vi "SQL_CLIENT_MAIN.vi"() -> ()   [LabVIEW 2020]
uses:
  SQL_CLIENT/MAIN/REF_EDITOR/REF_EDIT_type_filter.ctl
  SQL_CLIENT/MAIN/REPORTS/REPORTS_filters.ctl
  SQL_CLIENT/MAIN/REPORTS/REPORT_filter.ctl
  SQL_CLIENT/MAIN/REPORTS/GEAR/typedef/REPORT_GEAR_header_data_display.ctl
  SQL_CLIENT/MAIN/REPORTS/OPERATION/typedef/REPORT_OPRTN_operation.ctl
  SQL_CLIENT/MAIN/REPORTS/CONFIG_HISTORY/typedef/REPORT_CFG_types.ctl
  SQL_CLIENT/MAIN/REPORTS/REWORKS/typedef/REPORT_REWORKS_stations.ctl
  SQL_CLIENT/ini/typedef/CLIENT_all_config_info.ctl
  SQL_CLIENT/ini/typedef/CLIENT_main_ini_file.ctl
  SQL_CLIENT/queues/typedef/CLIENT_queue_refnums.ctl
  SQL_CLIENT/queues/typedef/SQL_EDITOR_queue_element.ctl
  SQL_CLIENT/MAIN/SQL_EDITOR/SQL_EDITOR_sequence_state.ctl
  SQL_CLIENT/queues/typedef/CLIENT_SCANNER_queue_element.ctl
  SQL_CLIENT/MAIN/SCANNER/SCANNER_sequence_state.ctl
  SQL_CLIENT/queues/typedef/CLIENT_REF_CHG_queue_element.ctl
  SQL_CLIENT/MAIN/reference_changed_connection/CLIENT_REF_CHG_sequence_state.ctl
  SQL_CLIENT/FGV/error_buffer/FGV_CLIENT_error_buffer.ctl
  SQL_CLIENT/FGV/SQL_EDITOR_records_display/FGV_SQL_EDITOR_records_display.ctl
  SQL_CLIENT/FGV/SQL_EDITOR_status_display/FGV_SQL_EDITOR_status_display.ctl
  SQL_CLIENT/FGV/SQL_connection/FGV_CLIENT_SQL_connection.ctl
  SQL_CLIENT/FGV/REF_EDITOR_records_display/FGV_REF_EDITOR_records_display.ctl
  SQL_CLIENT/FGV/REF_EDITOR_status_display/FGV_REF_EDITOR_status_display.ctl
  SQL_CLIENT/MAIN/CLIENT_event_structure_shift_register.ctl
  SQL_CLIENT/FGV/ARCH_EDITOR_status_display/FGV_ARCH_EDITOR_status_display.ctl
  SQL_CLIENT/FGV/ARCH_EDITOR_records_display/FGV_ARCH_EDITOR_records_display.ctl
  SQL_CLIENT/FGV/SQL_TEXT_status_display/FGV_SQL_TEXT_status_display.ctl
  SQL_CLIENT/FGV/SQL_TEXT_records_display/FGV_SQL_TEXT_records_display.ctl
  SQL_CLIENT/FGV/USER_EDITOR_status_display/FGV_USER_EDITOR_status_display.ctl
  SQL_CLIENT/FGV/USER_EDITOR_records_display/FGV_USER_EDITOR_records_display.ctl
  SQL_CLIENT/FGV/login/FGV_login.ctl
  SQL_CLIENT/FGV/REPORTS_status_display/FGV_REPORTS_status_display.ctl
  SQL_CLIENT/FGV/REPORTS_records_display/FGV_REPORTS_records_display.ctl
  SQL_CLIENT/FGV/REPORTS_records_display/REPORTS_references.ctl
  _misc/directions.ctl
  SQL_CLIENT/MAIN/REPORTS/AUDIT/typedef/REPORT_AUDIT_filters.ctl
  <vilib>/Utility/miscctls.llb/LVRowAndColumnTypeDef.ctl
  SQL_CLIENT/MAIN/REPORTS/CONFIG_HISTORY/typedef/REPORT_CFG_filters.ctl
  SQL_CLIENT/MAIN/REPORTS/DATES/typedef/REPORT_DATES_filters.ctl
  SQL_CLIENT/MAIN/REPORTS/OPERATION/typedef/REPORT_OPRTN_filters.ctl
  SQL_CLIENT/MAIN/REPORTS/PRODUCTION_BATCH/typedef/REPORT_PBATCH_filters.ctl
  SQL_CLIENT/MAIN/thread_name.ctl
  _misc/AULocalize/SubVIs/RegisterVI.vi
  _misc/AULocalize/SubVIs/Get Localized Phrase Compact Interface 0D.vi
  <vilib>/Instr/_visa.llb/VISA Configure Serial Port (Instr).vi
  <vilib>/regexp/Match Regular Expression.xnode
panel:
  out "app_title":string caption="A603 - SQL Client"
  out "PLC_PROXY_connection_indicator":bool=TRUE caption="PLC Proxy Connection Status:"
  in  "USER_login_logout":bool
  out "SQL_connection_indicator":bool=TRUE caption="SQL Connection Status:"
  in  "STOP":bool
  out "error_indicator_global":bool caption="Application Status:"
  in  "current_access_level":i32=10 caption="Access level:"
  in  "current_username":string="jlonga" caption="Logged in as:"
  in  "main_tab":T1(tab)
  in  "REPORT_save_csv":bool
  in  "REPORT_clear":bool
  out "REPORT_page_counter":string
  in  "REPORT_page_last":bool
  in  "REPORT_page_next":bool
  in  "REPORT_page_previous":bool
  in  "REPORT_page_first":bool
  in  "REPORT_save_pdf":bool
  in  "REPORT_get":bool
  in  "REPORT_filters":T2
  out "REPORT_GEAR_serial_display":string
  in  "REPORT_GEAR_toggle_all_results":bool
  in  "REPORT_GEAR_station":T3 caption="OP Filter:" items=["ALL", "10", "20", "30", "40"]
  in  "REPORT_GEAR_scan_barcode":bool
  in  "REPORT_GEAR_serial":string caption="Gear Serial:"
  out "REPORT_GEAR_header_data_display":T4
  out "gear_info_summary_header":string caption="GEAR INFO SUMMARY"
  in  "REPORT_DATES_last_status":T3 caption="Last Status:" items=["ALL", "0", "IN OPERATION", "INTERRUPTED", "NOK", "OK"]
  in  "REPORT_DATES_last_op":T3 caption="Last OP:" items=["ALL", "0", "10", "20", "40", "50", "60", "70", "80", "90", "100", "110", "120", "130", "160", "165"]
  in  "REPORT_DATES_time_end":timestamp caption="End:" format="%<%H:%M:%S>T"
  in  "REPORT_DATES_time_start":timestamp caption="Start:" format="%<%H:%M:%S>T"
  in  "REPORT_DATES_start":timestamp caption="From:" format="%<%x %H:%M:%S>T"
  in  "REPORT_DATES_start_btn":bool
  in  "REPORT_DATES_end":timestamp caption="To:" format="%<%x %H:%M:%S>T"
  in  "REPORT_DATES_end_btn":bool
  in  "REPORT_DATES_order_selection":enum32{"old_to_new", "new_to_old"}(radio)
  out "timeframe_header":string caption="TIMEFRAME"
  out "timeofday_header":string caption="TIME OF DAY / SHIFT"
  out "order_header":string caption="ORDER"
  out "filters_header":string caption="FILTERS"
  in  "REPORT_PBATCH_last_status":T3 caption="Last Status:" items=[" -"]
  in  "REPORT_PBATCH_last_op":T3 caption="Last OP:" items=[" -"]
  in  "REPORT_PBATCH_order_selection":enum32{"old_to_new", "new_to_old"}(radio)
  in  "REPORT_PBATCH_batch_no":string caption="Batch No:"
  out "batch_header":string caption="BATCH"
  out "order_header":string caption="ORDER"
  out "filters_header":string caption="FILTERS"
  in  "REPORT_OPRTN_order_selection":enum32{"old_to_new", "new_to_old"}(radio)
  in  "REPORT_OPRTN_end_btn":bool
  in  "REPORT_OPRTN_end":timestamp caption="To:" format="%<%x %H:%M:%S>T"
  in  "REPORT_OPRTN_start_btn":bool
  in  "REPORT_OPRTN_start":timestamp caption="From:" format="%<%x %H:%M:%S>T"
  in  "REPORT_OPRTN_time_start":timestamp caption="Start:" format="%<%H:%M:%S>T"
  in  "REPORT_OPRTN_time_end":timestamp caption="End:" format="%<%H:%M:%S>T"
  in  "REPORT_OPRTN_last_status":T3 caption="Last Status:" items=[" -"]
  in  "REPORT_OPRTN_operation":T5 caption="OP:" items=["10"=10, "20"=20, "30"=30, "40"=40, "50"=50, "60"=60, "70"=70, "80"=80, "90"=90, "100"=100, "110"=110, "120"=120, "130"=130, "140"=140, "150"=150, "160"=160, "165"=165]
  in  "REPORT_OPRTN_filter_columns":bool
  in  "REPORT_OPRTN_unfilter_columns":bool
  out "operation_header":string caption="OPERATION"
  out "timeframe_header":string caption="TIMEFRAME"
  out "timeofday_header":string caption="TIME OF DAY / SHIFT"
  out "order_header":string caption="ORDER"
  out "filters_header":string caption="FILTERS"
  in  "REPORT_CFG_type":T6 caption="Config:"
  in  "REPORT_CFG_time_end":timestamp caption="End:" format="%<%H:%M:%S>T"
  in  "REPORT_CFG_time_start":timestamp caption="Start:" format="%<%H:%M:%S>T"
  in  "REPORT_CFG_start":timestamp caption="From:" format="%<%x %H:%M:%S>T"
  in  "REPORT_CFG_start_btn":bool
  in  "REPORT_CFG_end":timestamp caption="To:" format="%<%x %H:%M:%S>T"
  in  "REPORT_CFG_end_btn":bool
  in  "REPORT_CFG_order_selection":enum32{"old_to_new", "new_to_old"}(radio)
  in  "REPORT_CFG_op_filter":T3 caption="OP:" items=[" -"]
  out "configtype_header":string caption="CONFIG TYPE"
  out "timeframe_header":string caption="TIMEFRAME"
  out "timeofday_header":string caption="TIME OF DAY / SHIFT"
  out "order_header":string caption="ORDER"
  out "filters_header":string caption="FILTERS"
  in  "REPORT_AUDIT_order_selection":enum32{"old_to_new", "new_to_old"}(radio)
  in  "REPORT_AUDIT_end_btn":bool
  in  "REPORT_AUDIT_end":timestamp caption="To:" format="%<%x %H:%M:%S>T"
  in  "REPORT_AUDIT_start_btn":bool
  in  "REPORT_AUDIT_start":timestamp caption="From:" format="%<%x %H:%M:%S>T"
  in  "REPORT_AUDIT_time_start":timestamp caption="Start:" format="%<%H:%M:%S>T"
  in  "REPORT_AUDIT_time_end":timestamp caption="End:" format="%<%H:%M:%S>T"
  in  "REPORT_AUDIT_OP_filter":T3 caption="Audit OP:" items=["ALL", "10", "20", "30", "40", "50", "60", "70", "80", "90", "100", "120", "165"]
  in  "REPORT_AUDIT_status_filter":T3 caption="Audit Status:" items=["ALL", "0", "NOK", "OK"]
  out "timeframe_header":string caption="TIMEFRAME"
  out "timeofday_header":string caption="TIME OF DAY / SHIFT"
  out "order_header":string caption="ORDER"
  out "filters_header":string caption="FILTERS"
  in  "REPORT_AUDIT_toggle_all_results":bool
  in  "REPORT_OKNOK_time_end":timestamp caption="End:" format="%<%H:%M:%S>T"
  in  "REPORT_OKNOK_time_start":timestamp caption="Start:" format="%<%H:%M:%S>T"
  in  "REPORT_OKNOK_start":timestamp caption="From:" format="%<%x %H:%M:%S>T"
  in  "REPORT_OKNOK_start_btn":bool
  in  "REPORT_OKNOK_end":timestamp caption="To:" format="%<%x %H:%M:%S>T"
  in  "REPORT_OKNOK_end_btn":bool
  out "timeframe_header":string caption="TIMEFRAME"
  out "timeofday_header":string caption="TIME OF DAY / SHIFT"
  in  "REPORT_REWORKS_end_btn":bool
  in  "REPORT_REWORKS_end":timestamp caption="To:" format="%<%x %H:%M:%S>T"
  in  "REPORT_REWORKS_start_btn":bool
  in  "REPORT_REWORKS_start":timestamp caption="From:" format="%<%x %H:%M:%S>T"
  in  "REPORT_REWORKS_time_start":timestamp caption="Start:" format="%<%H:%M:%S>T"
  in  "REPORT_REWORKS_time_end":timestamp caption="End:" format="%<%H:%M:%S>T"
  in  "REPORT_REWORKS_to_OP":T7 caption="To OP:" items=["0"=0, "10"=10, "20"=20, "30"=30, "40"=40, "50"=50, "60"=60, "70"=70, "80"=80, "90"=90, "100"=100, "110"=110, "120"=120, "130"=130, "140"=140, "150"=150, "160"=160, "165"=165]
  in  "REPORT_REWORKS_from_OP":T7 caption="From OP:" items=["0"=0, "10"=10, "20"=20, "30"=30, "40"=40, "50"=50, "60"=60, "70"=70, "80"=80, "90"=90, "100"=100, "110"=110, "120"=120, "130"=130, "140"=140, "150"=150, "160"=160, "165"=165]
  in  "REPORT_REWORKS_order_selection":enum32{"old_to_new", "new_to_old"}(radio)
  out "timeframe_header":string caption="TIMEFRAME"
  out "timeofday_header":string caption="TIME OF DAY / SHIFT"
  out "sourcedestination_header":string caption="SOURCE AND DESTIONATION"
  out "order_header":string caption="ORDER"
  in  "REPORT_PACE_end_btn":bool
  in  "REPORT_PACE_end":timestamp caption="To:" format="%<%x %H:%M:%S>T"
  in  "REPORT_PACE_start_btn":bool
  in  "REPORT_PACE_start":timestamp caption="From:" format="%<%x %H:%M:%S>T"
  in  "REPORT_PACE_time_start":timestamp caption="Start:" format="%<%H:%M:%S>T"
  in  "REPORT_PACE_time_end":timestamp caption="End:" format="%<%H:%M:%S>T"
  in  "REPORT_PACE_low_limit":u16 caption="Low:" step=1
  in  "REPORT_PACE_high_limit":u16 caption="High:" step=1
  out "timeframe_header":string caption="TIMEFRAME"
  out "timeofday_header":string caption="TIME OF DAY / SHIFT"
  out "pacelimits_header":string caption="PACE LIMITS (SECONDS)"
  in  "REPORT_CBATCH_batch_code":string caption="Batch:"
  in  "REPORT_CBATCH_scan_barcode":bool
  in  "REPORT_CBATCH_order_selection":enum32{"old_to_new", "new_to_old"}(radio)
  out "order_header":string caption="ORDER"
  in  "REPORT_CMPNT_scan_barcode":bool
  in  "REPORT_CMPNT_gear_serial":string caption="Gear Serial:"
  in  "REPORT_records":i32(listbox)=-1
  out "REPORT_status":string
  in  "REF_EDIT_type_filter":T8 caption="Type:"
  in  "REF_EDIT_records":i32(listbox)
  in  "REF_EDIT_station":u16(ring) caption="Station:" items=["10", "20", "30", "40", "50", "60", "70", "80", "90", "100", "110", "120", "130", "160", "165"]
  out "REF_EDIT_status":string
  in  "REF_EDIT_refresh":bool
  in  "REF_EDIT_delete":bool
  in  "REF_EDIT_insert_update":bool
  in  "REF_EDIT_clear_status":bool
  in  "REF_EDIT_discard":bool
  in  "ARCH_EDIT_type_filter":T8 caption="Type:"
  in  "ARCH_EDIT_records":i32(listbox)
  in  "ARCH_EDIT_station":u16(ring) caption="Station:" items=["10", "20", "30", "40", "50", "60", "70", "80", "90", "100", "110", "120", "130", "140", "160", "165"]
  out "ARCH_EDIT_status":string
  in  "ARCH_EDIT_refresh":bool
  in  "ARCH_EDIT_delete":bool
  in  "ARCH_EDIT_insert_update":bool
  in  "ARCH_EDIT_clear_status":bool
  in  "ARCH_EDIT_discard":bool
  in  "USER_EDIT_refresh":bool
  out "USER_EDIT_status":string
  in  "USER_EDIT_records":i32(listbox)
  in  "USER_EDIT_insert_update":bool
  in  "USER_EDIT_delete":bool
  in  "USER_EDIT_clear_status":bool
  in  "USER_EDIT_discard":bool
  in  "USER_EDIT_update_barcode":bool
  in  "SQL_EDIT_asc_desc":enum32{"ASC", "DESC"}(radio)
  in  "SQL_EDIT_order_by":u16(ring) caption="Order by:" items=["ID", "CREATION_TIME", "REFERENCE_NAME", "STATION_NMB", "DESCRIPTION", "UNIT", "PLC_TAG_TYPE", "PLC_TAG_ADDRESS", "CREATED_BY"]
  in  "SQL_EDIT_discard":bool
  in  "SQL_EDIT_clear_status":bool
  in  "SQL_EDIT_select":bool
  in  "SQL_EDIT_value":string caption="Value:"
  in  "SQL_EDIT_table":u16(ring) caption="Table:" items=["ARCHIVISATION_AUDIT", "ARCHIVISATION_CFG", "ARCHIVISATION_CFG_HISTORY", "AUDIT_RESULTS", "AUDIT_RESULTS_REAL", "DOCK_AUDIT_BATCH_COUNT", "DOCK_AUDIT_BATCH_SIZE", "DOCK_AUDIT_BATCHES", "MAX_REPEAT_COUNT", "OEE_AVAILABILITY", "OEE_CONFIG", "OEE_SHIFT_TIMES", "OEE_tmp_operations_memory_optimized", "PRODUCTION_BATCHES", "PRODUCTION_BATCHES_OPERATIONS", "PRODUCTION_PARTS", "PRODUCTION_PARTS_OPERATIONS", "PRODUCTION_PARTS_OPERATIONS_RESULTS_REAL", "PRODUCTION_PARTS_OPERATIONS_RESULTS_STRING", "PRODUCTION_PINIONS", "REFERENCE", "REFERENCE_HISTORY", "REWORK", "ROUTING", "USER_DATA", "USER_DATA_HISTORY"]
  in  "SQL_EDIT_column":u16(ring) caption="Column:" items=["ID", "CREATION_TIME", "REFERENCE_NAME", "STATION_NMB", "DESCRIPTION", "UNIT", "PLC_TAG_TYPE", "PLC_TAG_ADDRESS", "CREATED_BY"]
  in  "SQL_EDIT_insert_update":bool
  in  "SQL_EDIT_delete":bool
  in  "SQL_EDIT_records":i32(listbox)=-1
  out "SQL_EDIT_status":string
  in  "SQL_TEXT_execute":bool
  in  "SQL_TEXT_clear_status":bool
  in  "SQL_TEXT_input":string
  out "SQL_TEXT_status":string
  in  "SQL_TEXT_records":i32(listbox)
  in  "main_error":i32(listbox)
  in  "ERRORS_clear":bool
  out "error_indicator_tab":bool
  # "Access Levels:"
  # "1 - Operator, 2 - Leader, 3 - Maintenance, 7 - Engineer, 10 - Admin"
  # "WARNING! - SQL COMMANDS EXECUTED IN THIS WINDOW ARE NOT VALIDATED IN ANY WAY AND CAN IRREVERSIBLY DAMAGE THE DATABASE! - PROCEED WITH EXTREME CAUTION!"
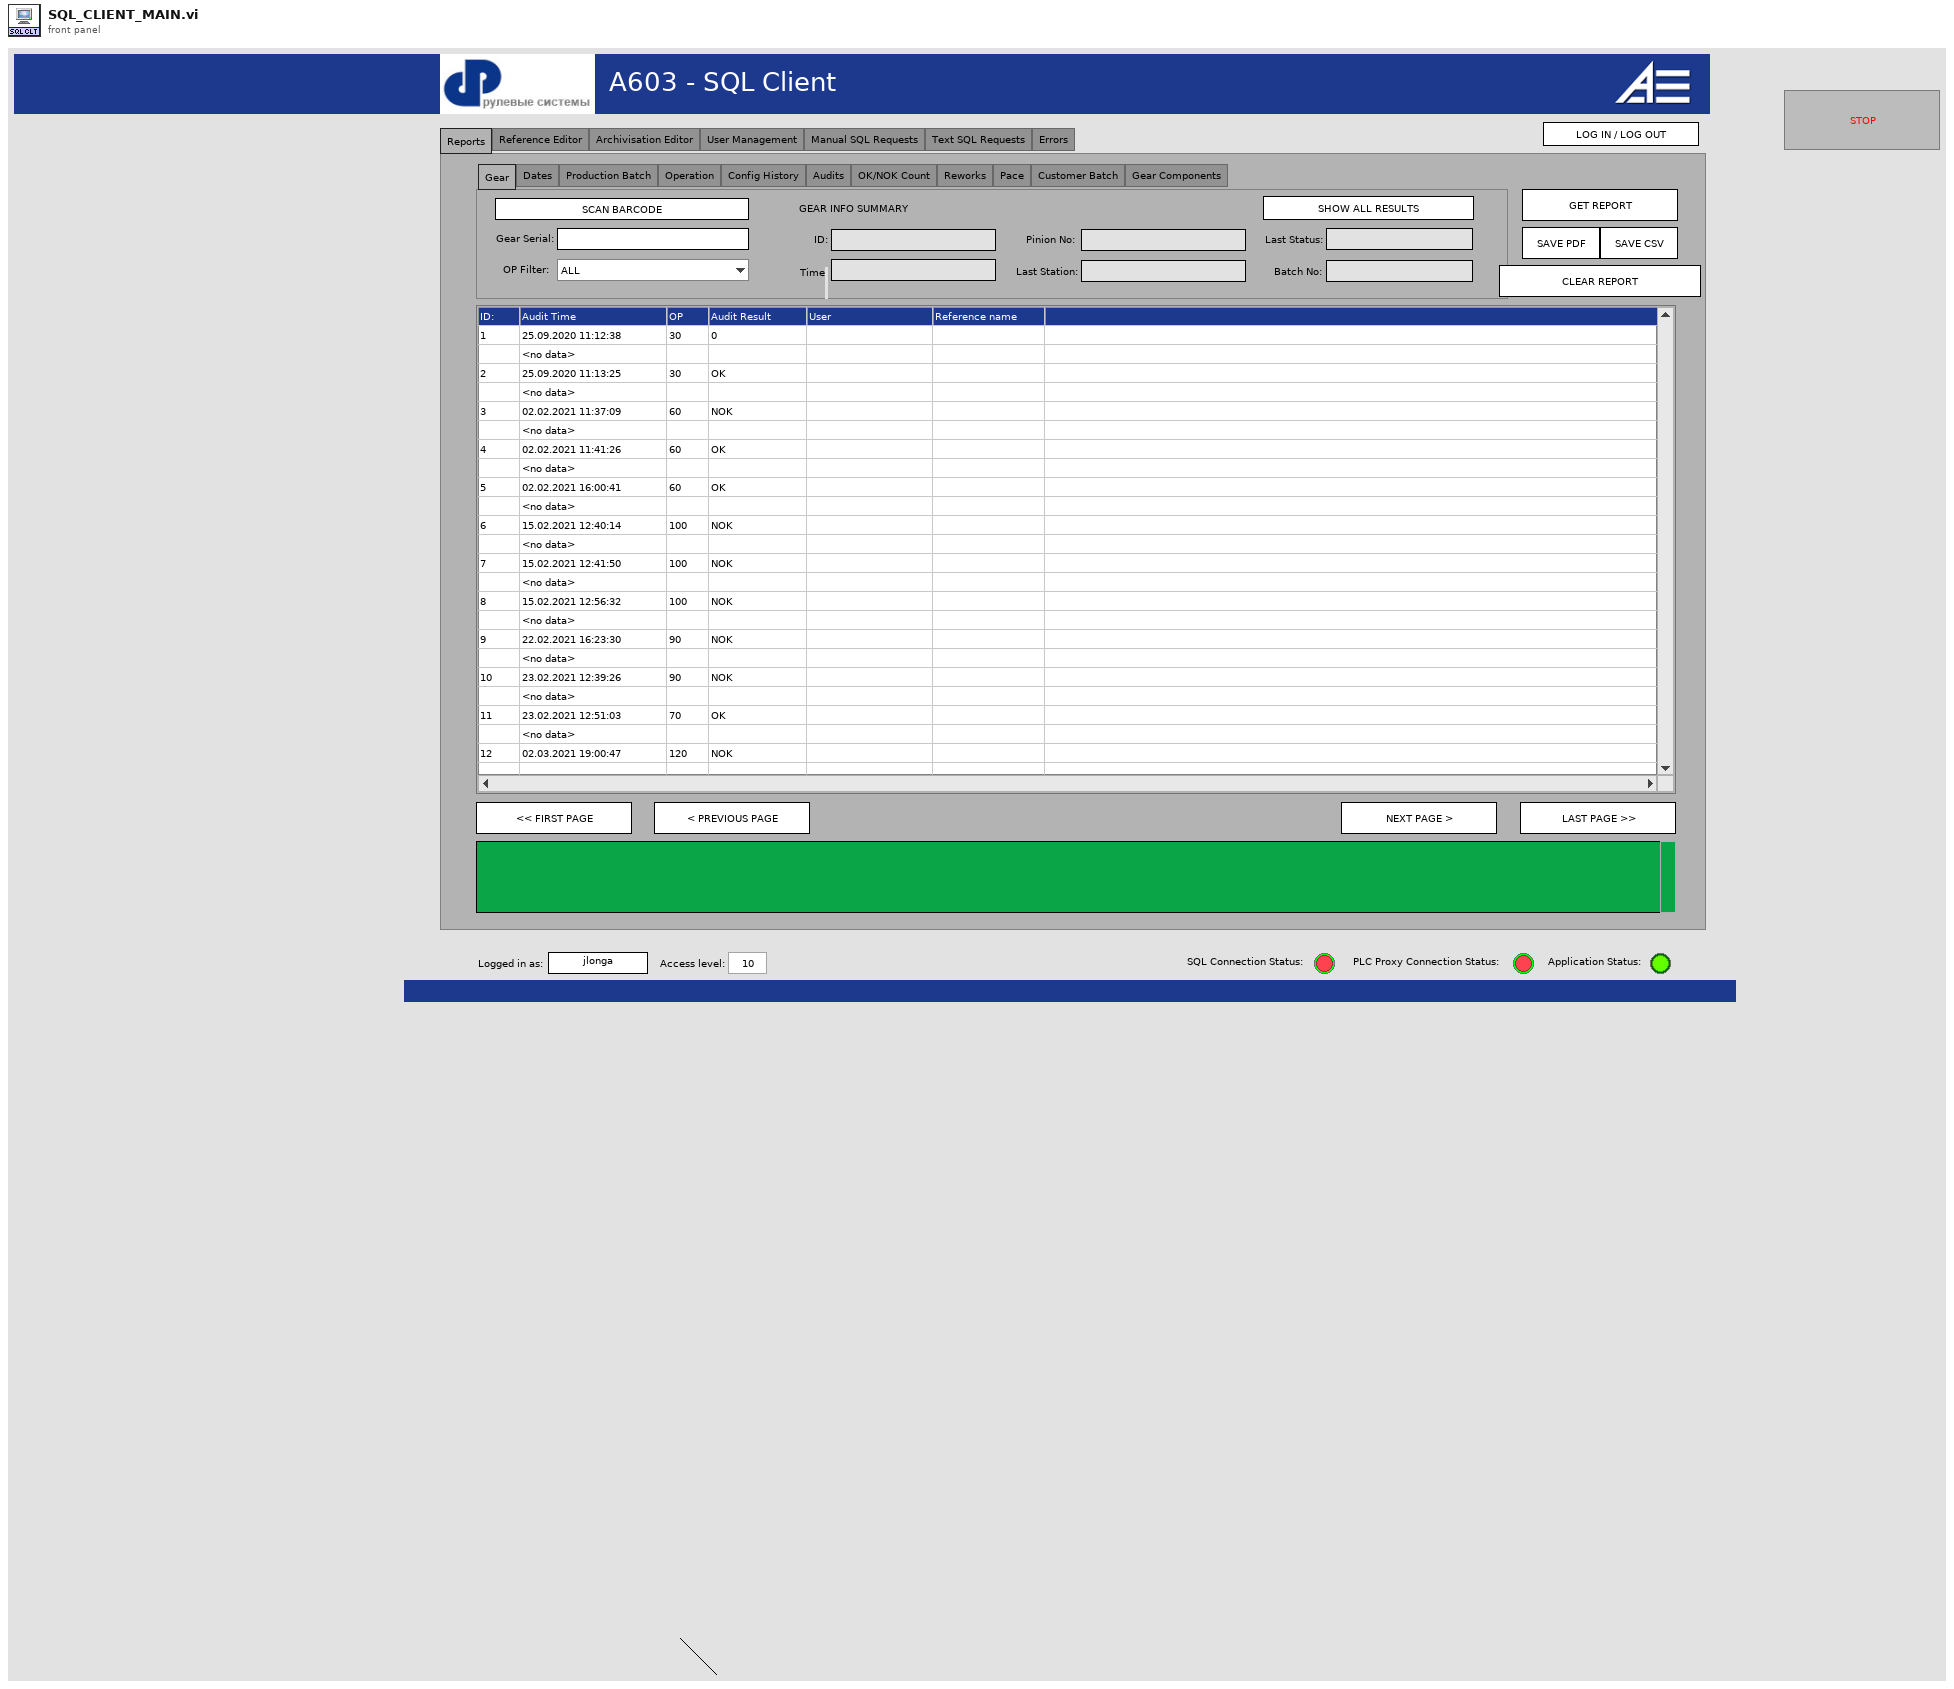
[diagram p1: front panel]
types:
  T1 = enum32{"Reports", "Reference Editor", "Archivisation Editor", "User Management", "Manual SQL Requests", "Text SQL Requests", "Errors"}
  T2 = typedef "REPORTS_filters.ctl" = enum32{"Gear", "Dates", "Production Batch", "Operation", "Config History", "Audits", "OK/NOK Count", "Reworks", "Pace", "Customer Batch", "Gear Components"}
  T3 = typedef "REPORT_filter.ctl" = u16
  T4 = typedef "REPORT_GEAR_header_data_display.ctl" = cluster{"ID":string, "creation_time":string, "last_station":string, "last_status":string, "pinion_serial":string, "batch_code":string}
  T5 = typedef "REPORT_OPRTN_operation.ctl" = u16
  T6 = typedef "REPORT_CFG_types.ctl" = enum16{"REFERENCE", "ARCHIVISATION", "USERS"}
  T7 = typedef "REPORT_REWORKS_stations.ctl" = u16
  T8 = typedef "REF_EDIT_type_filter.ctl" = enum32{"ALL", "INT", "REAL", "STRING"}
  T9 = typedef "CLIENT_REF_CHG_sequence_state.ctl" = enum16{"initialize", "get_next_state", "reference_changed", "ping", "error", "stop"}
  T10 = typedef "REPORTS_references.ctl" = cluster{"front_panel_reference":refnum<vi>, "SQL_listbox_reference":refnum<vi>, "REPORT_page_first":refnum<vi>, "REPORT_page_previous":refnum<vi>, "REPORT_page_next":refnum<vi>, "REPORT_page_last":refnum<vi>, "REPORT_page_counter":refnum<vi>, "REPORT_GEAR_serial":refnum<vi>, "REPORT_GEAR_serial_display":refnum<vi>, "REPORT_GEAR_station":refnum<vi>, "REPORT_GEAR_header_data_display":refnum<vi>, "REPORT_DATES_start":refnum<vi>, "REPORT_DATES_end":refnum<vi>, "REPORT_DATES_time_start":refnum<vi>, "REPORT_DATES_time_end":refnum<vi>, "REPORT_DATES_order_selection":refnum<vi>, "REPORT_DATES_last_OP":refnum<vi>, "REPORT_DATES_last_status":refnum<vi>, "REPORT_PBATCH_batch_no":refnum<vi>, "REPORT_PBATCH_order_selection":refnum<vi>, "REPORT_PBATCH_last_op":refnum<vi>, "REPORT_PBATCH_last_status":refnum<vi>, "REPORT_OPRTN_operation":refnum<vi>, "REPORT_OPRTN_start":refnum<vi>, "REPORT_OPRTN_end":refnum<vi>, "REPORT_OPRTN_time_start":refnum<vi>, "REPORT_OPRTN_time_end":refnum<vi>, "REPORT_OPRTN_order_selection":refnum<vi>, "REPORT_OPRTN_last_status":refnum<vi>, "REPORT_CFG_type":refnum<vi>, "REPORT_CFG_start":refnum<vi>, "REPORT_CFG_end":refnum<vi>, "REPORT_CFG_time_start":refnum<vi>, "REPORT_CFG_time_end":refnum<vi>, "REPORT_CFG_order_selection":refnum<vi>, "REPORT_CFG_op_filter":refnum<vi>, "REPORT_AUDIT_start":refnum<vi>, "REPORT_AUDIT_end":refnum<vi>, "REPORT_AUDIT_time_start":refnum<vi>, "REPORT_AUDIT_time_end":refnum<vi>, "REPORT_AUDIT_order_selection":refnum<vi>, "REPORT_AUDIT_op_filter":refnum<vi>, "REPORT_AUDIT_status_filter":refnum<vi>, "REPORT_OKNOK_start":refnum<vi>, "REPORT_OKNOK_end":refnum<vi>, "REPORT_OKNOK_time_start":refnum<vi>, "REPORT_OKNOK_time_end":refnum<vi>, "REPORT_REWORKS_start":refnum<vi>, "REPORT_REWORKS_end":refnum<vi>, "REPORT_REWORKS_time_start":refnum<vi>, "REPORT_REWORKS_time_end":refnum<vi>, "REPORT_REWORKS_from_OP":refnum<vi>, "REPORT_REWORKS_to_OP":refnum<vi>, "REPORT_REWORKS_order_selection":refnum<vi>, "REPORT_PACE_start":refnum<vi>, "REPORT_PACE_end":refnum<vi>, "REPORT_PACE_time_start":refnum<vi>, "REPORT_PACE_time_end":refnum<vi>, "REPORT_PACE_low_limit":refnum<vi>, "REPORT_PACE_high_limit":refnum<vi>, "REPORT_CBATCH_batch_code":refnum<vi>, "REPORT_CBATCH_order_selection":refnum<vi>, "REPORT_CMPNT_gear_serial":refnum<vi>}
  T11 = typedef "FGV_REPORTS_records_display.ctl" = enum16{"initialize", "GEAR_set_serial", "GEAR_set_header", "GEAR_set_operations", "GEAR_set_results", "GEAR_set_batches", "GEAR_get_serial", "GEAR_get_operation_IDs", "GEAR_toggle_results", "GEAR_show_all_results", "GEAR_hide_all_results", "GEAR_display", "GEAR_filter", "GEAR_restore", "GEAR_clear", "GEAR_get_all_info", "DATES_set_dates", "DATES_set_gears", "DATES_display", "DATES_filter", "DATES_first_page", "DATES_previous_page", "DATES_next_page", "DATES_last_page", "DATES_restore", "DATES_clear", "DATES_get_all_info", "PBATCH_set_batch_no", "PBATCH_set_gears", "PBATCH_display", "PBATCH_filter", "PBATCH_first_page", "PBATCH_previous_page", "PBATCH_next_page", "PBATCH_last_page", "PBATCH_restore", "PBATCH_clear", "PBATCH_get_all_info", "OPRTN_set_OP", "OPRTN_set_dates", "OPRTN_set_gears", "OPRTN_set_hidden_columns", "OPRTN_display", "OPRTN_filter", "OPRTN_filter_no_page_reset", "OPRTN_first_page", "OPRTN_previous_page", "OPRTN_next_page", "OPRTN_last_page", "OPRTN_restore", "OPRTN_clear", "OPRTN_get_all_info", "CFG_set_type", "CFG_set_dates", "CFG_set_records", "CFG_display", "CFG_filter", "CFG_first_page", "CFG_previous_page", "CFG_next_page", "CFG_last_page", "CFG_restore", "CFG_clear", "CFG_get_all_info", "AUDIT_set_dates", "AUDIT_set_records", "AUDIT_display", "AUDIT_filter", "AUDIT_first_page", "AUDIT_previous_page", "AUDIT_next_page", "AUDIT_last_page", "AUDIT_restore", "AUDIT_clear", "AUDIT_set_results", "AUDIT_get_all_info", "AUDIT_toggle_results", "AUDIT_show_all_results", "AUDIT_hide_all_results", "OKNOK_set_dates", "OKNOK_set_records", "OKNOK_display", "OKNOK_restore", "OKNOK_clear", "OKNOK_get_all_info", "REWORKS_set_dates", "REWORKS_set_from_to", "REWORKS_set_records", "REWORKS_display", "REWORKS_filter", "REWORKS_first_page", "REWORKS_previous_page", "REWORKS_next_page", "REWORKS_last_page", "REWORKS_restore", "REWORKS_clear", "REWORKS_get_all_info", "PACE_set_dates", "PACE_set_limits", "PACE_set_records", "PACE_display", "PACE_restore", "PACE_clear", "PACE_get_all_info", "CBATCH_set_code", "CBATCH_set_records", "CBATCH_display", "CBATCH_filter", "CBATCH_first_page", "CBATCH_previous_page", "CBATCH_next_page", "CBATCH_last_page", "CBATCH_restore", "CBATCH_clear", "CBATCH_get_all_info", "CMPNT_set_serial", "CMPNT_set_records", "CMPNT_display", "CMPNT_first_page", "CMPNT_previous_page", "CMPNT_next_page", "CMPNT_last_page", "CMPNT_restore", "CMPNT_clear", "CMPNT_get_all_info", "clear"}
  T12 = typedef "FGV_REPORTS_status_display.ctl" = enum16{"initialize", "display", "clear"}
  T13 = typedef "FGV_login.ctl" = enum16{"initialize", "login", "logout", "get_login_info"}
  T14 = typedef "FGV_USER_EDITOR_records_display.ctl" = enum16{"initialize", "set_user_edit_tables_names", "set_headers", "set_records", "get_user_edit_table_name", "get_user_edit_hist_table_name", "get_headers", "get_uneditable_columns", "get_all_info", "record_added?", "record_inserted?", "record_edited?", "record_updated?", "record_deleted?", "discard_changes"}
  T15 = typedef "FGV_USER_EDITOR_status_display.ctl" = enum16{"initialize", "display", "clear"}
  T16 = typedef "FGV_SQL_TEXT_records_display.ctl" = enum16{"initialize", "set", "clear"}
  T17 = typedef "FGV_SQL_TEXT_status_display.ctl" = enum16{"initialize", "display", "clear"}
  T18 = typedef "SCANNER_sequence_state.ctl" = enum16{"initialize", "get_next_state", "read", "cancel_read", "error", "stop"}
  T19 = typedef "FGV_ARCH_EDITOR_records_display.ctl" = enum16{"initialize", "set_arch_cfg_tables_names", "set_station_number", "set_type_filter", "set_headers", "set_records", "get_arch_cfg_table_name", "get_arch_cfg_hist_table_name", "get_station_number", "get_type_filter", "get_headers", "get_uneditable_columns", "get_all_info", "record_added?", "record_inserted?", "record_edited?", "record_updated?", "record_deleted?", "discard_changes"}
  T20 = typedef "FGV_ARCH_EDITOR_status_display.ctl" = enum16{"initialize", "display", "clear"}
  T21 = typedef "CLIENT_event_structure_shift_register.ctl" = cluster{"REF_EDIT_clicked_row":i32, "REF_EDIT_selected_row":i32, "SQL_EDIT_clicked_row":i32, "SQL_EDIT_selected_row":i32, "ARCH_EDIT_selected_row":i32, "ARCH_EDIT_clicked_row":i32, "USER_EDIT_selected_row":i32, "USER_EDIT_clicked_row":i32, "REPORT_GEAR_toggle_all_results":bool, "REPORT_AUDIT_toggle_all_results":bool}
  T22 = typedef "FGV_REF_EDITOR_status_display.ctl" = enum16{"initialize", "display", "clear"}
  T23 = typedef "FGV_REF_EDITOR_records_display.ctl" = enum16{"initialize", "set_reference_tables_names", "set_station_number", "set_type_filter", "set_headers", "set_records", "get_ref_table_name", "get_ref_hist_table_name", "get_station_number", "get_type_filter", "get_headers", "get_uneditable_columns", "get_all_info", "record_added?", "record_inserted?", "record_edited?", "record_updated?", "record_deleted?", "discard_changes"}
  T24 = typedef "FGV_CLIENT_SQL_connection.ctl" = enum16{"initialize", "connect", "read_tables", "read_columns", "SELECT", "INSERT", "UPDATE", "DELETE", "EXEC + headers", "EXEC", "TRANSACTION", "connection_active?", "disconnect"}
  T25 = typedef "SQL_EDITOR_sequence_state.ctl" = enum16{"initialize", "get_next_state", "REF_read_columns", "REF_read_stations", "REF_select_station_records", "REF_insert_record", "REF_update_record", "REF_delete_record", "REF_send_reference_updated_to_PLC", "ARCH_read_columns", "ARCH_read_stations", "ARCH_select_station_records", "ARCH_insert_record", "ARCH_update_record", "ARCH_delete_record", "USER_read_columns", "USER_select_records", "USER_insert_record", "USER_update_record", "USER_delete_record", "USER_update_barcode", "USER_login", "USER_logout", "SQL_read_tables", "SQL_read_columns", "SQL_select_records", "SQL_insert_record", "SQL_update_record", "SQL_delete_record", "SQL_TEXT_execute", "REPORT_GEAR_scan_barcode", "REPORT_GEAR_get", "REPORT_DATES_get", "REPORT_PBATCH_get", "REPORT_OPRTN_get", "REPORT_CFG_get", "REPORT_AUDIT_get", "REPORT_OKNOK_get", "REPORT_REWORKS_get", "REPORT_PACE_get", "REPORT_CBATCH_scan_barcode", "REPORT_CBATCH_get", "REPORT_CMPNT_scan_barcode", "REPORT_CMPNT_get", "REPORT_save_pdf", "REPORT_save_csv", "error", "stop"}
  T26 = typedef "FGV_SQL_EDITOR_status_display.ctl" = enum16{"initialize", "display", "clear"}
  T27 = typedef "FGV_SQL_EDITOR_records_display.ctl" = enum16{"initialize", "set_table_name", "set_column_name", "set_value_to_select", "set_order_by", "set_asc_desc", "set_headers", "set_records", "get_table_name", "get_column_name", "get_value_to_select", "get_headers", "get_all_info", "record_added?", "record_inserted?", "record_edited?", "record_updated?", "record_deleted?", "discard_changes"}
  T28 = typedef "FGV_CLIENT_error_buffer.ctl" = enum16{"initialize", "clear", "display", "get_status"}
  T29 = typedef "CLIENT_all_config_info.ctl" = cluster{"main_ini_file":T30, "SQL Password":string, "queue_refnums":T31}
  T30 = typedef "CLIENT_main_ini_file.ctl" = cluster{"SQL Driver":string, "SQL Server":string, "SQL Database":string, "SQL UID":string, "Reference table":string, "Reference history":string, "Archivisation CFG table":string, "Archivisation CFG history":string, "User table":string, "User history":string, "logout timeout [ms]":i32, "records per page":i32, "default language":string, "REF CHG connection IP":string, "REF CHG remote port":i32, "REF CHG local port":i32, "SCANNER COM port":u16, "SCANNER Baud rate":u32, "SCANNER Data bits":u16, "SCANNER Pairity":enum16{"None", "Odd", "Even", "Mark", "Space"}, "SCANNER Stop bits":u16, "SCANNER Flow control":u16, "SCANNER Termination char":u8}
  T31 = typedef "CLIENT_queue_refnums.ctl" = cluster{"SQL_EDITOR_queue":refnum<queue>, "SCANNER_queue":refnum<queue>, "SCANNER_data":refnum<queue>, "CLIENT_REF_CHG_queue":refnum<queue>}
  T32 = typedef "SQL_EDITOR_queue_element.ctl" = cluster{"state":T25, "variable":variant}
  T33 = typedef "directions.ctl" = enum16{"UP", "DOWN", "LEFT", "RIGHT"}
  T34 = enum32{"Page Enabled", "Page Disabled", "Page Disabled & Grayed"}
  T35 = typedef "REPORT_AUDIT_filters.ctl" = cluster{"order_selection":enum32{"old_to_new", "new_to_old"}, "OP_filter":string, "status_filter":string, "show_hidden?":bool}
  T36 = typedef "LVRowAndColumnTypeDef.ctl" = cluster{"Row":i32, "Column":i32}
  T37 = typedef "REPORT_CFG_filters.ctl" = cluster{"order_selection":enum32{"old_to_new", "new_to_old"}, "OP":string}
  T38 = typedef "REPORT_DATES_filters.ctl" = cluster{"order_selection":enum32{"old_to_new", "new_to_old"}, "last_OP":string, "last_status":string}
  T39 = typedef "REPORT_OPRTN_filters.ctl" = cluster{"order_selection":enum32{"old_to_new", "new_to_old"}, "last_status":string}
  T40 = typedef "REPORT_PBATCH_filters.ctl" = cluster{"order_selection":enum32{"old_to_new", "new_to_old"}, "last_OP":string, "last_status":string}
  T41 = typedef "CLIENT_REF_CHG_queue_element.ctl" = cluster{"state":T9, "variable":variant}
  T42 = typedef "CLIENT_SCANNER_queue_element.ctl" = cluster{"state":T18, "variable":variant}
  T43 = typedef "ARCH_EDITOR_all_info.ctl" = cluster{"station_number":string, "type_filter":string, "archivisation_cfg_table":string, "archivisation_cfg_history":string, "column_names":string[], "uneditable_columns":string[], "uneditable_columns":i32[], "editable_columns":i32[], "values_in_database":string[][], "size":cluster{"columns":i32, "SQL_rows":i32, "disp_rows":i32}, "ARCH_record_states":T44[]}
  T44 = typedef "SQL_record_states.ctl" = enum16{"Equal", "Added", "Edited", "Deleted"}
  T45 = typedef "LVPoint32TypeDef.ctl" = cluster{"Horizontal":i32, "Vertical":i32}
  T46 = enum32{"Reports", "Reference Editor", "Archivisation Editor", "User Management", "Manual SQL Requests", "Text SQL Requests", "Errors"}[]
  T47 = typedef "REF_EDITOR_all_info.ctl" = cluster{"station_number":string, "type_filter":string, "reference_table":string, "reference_history":string, "headers":string[], "uneditable_columns":string[], "uneditable_columns":i32[], "editable_columns":i32[], "values_in_database":string[][], "size":cluster{"columns":i32, "SQL_rows":i32, "disp_rows":i32}, "REF_record_states":T44[]}
  T48 = typedef "SQL_EDITOR_all_info.ctl" = cluster{"table":string, "column":string, "value_to_select":string, "order_by":string, "asc_desc":string, "headers":string[], "uneditable_columns":string[], "uneditable_columns":i32[], "editable_columns":i32[], "values_in_database":string[][], "size":cluster{"columns":i32, "SQL_rows":i32, "disp_rows":i32}, "SQL_record_states":T44[]}
  T49 = typedef "USER_EDITOR_all_info.ctl" = cluster{"user_table":string, "user_history":string, "headers":string[], "uneditable_columns":string[], "uneditable_columns":i32[], "editable_columns":i32[], "values_in_database":string[][], "size":cluster{"columns":i32, "SQL_rows":i32, "disp_rows":i32}, "USER_record_states":T44[]}
  T50 = typedef "thread_name.ctl" = enum16{"MAIN"}
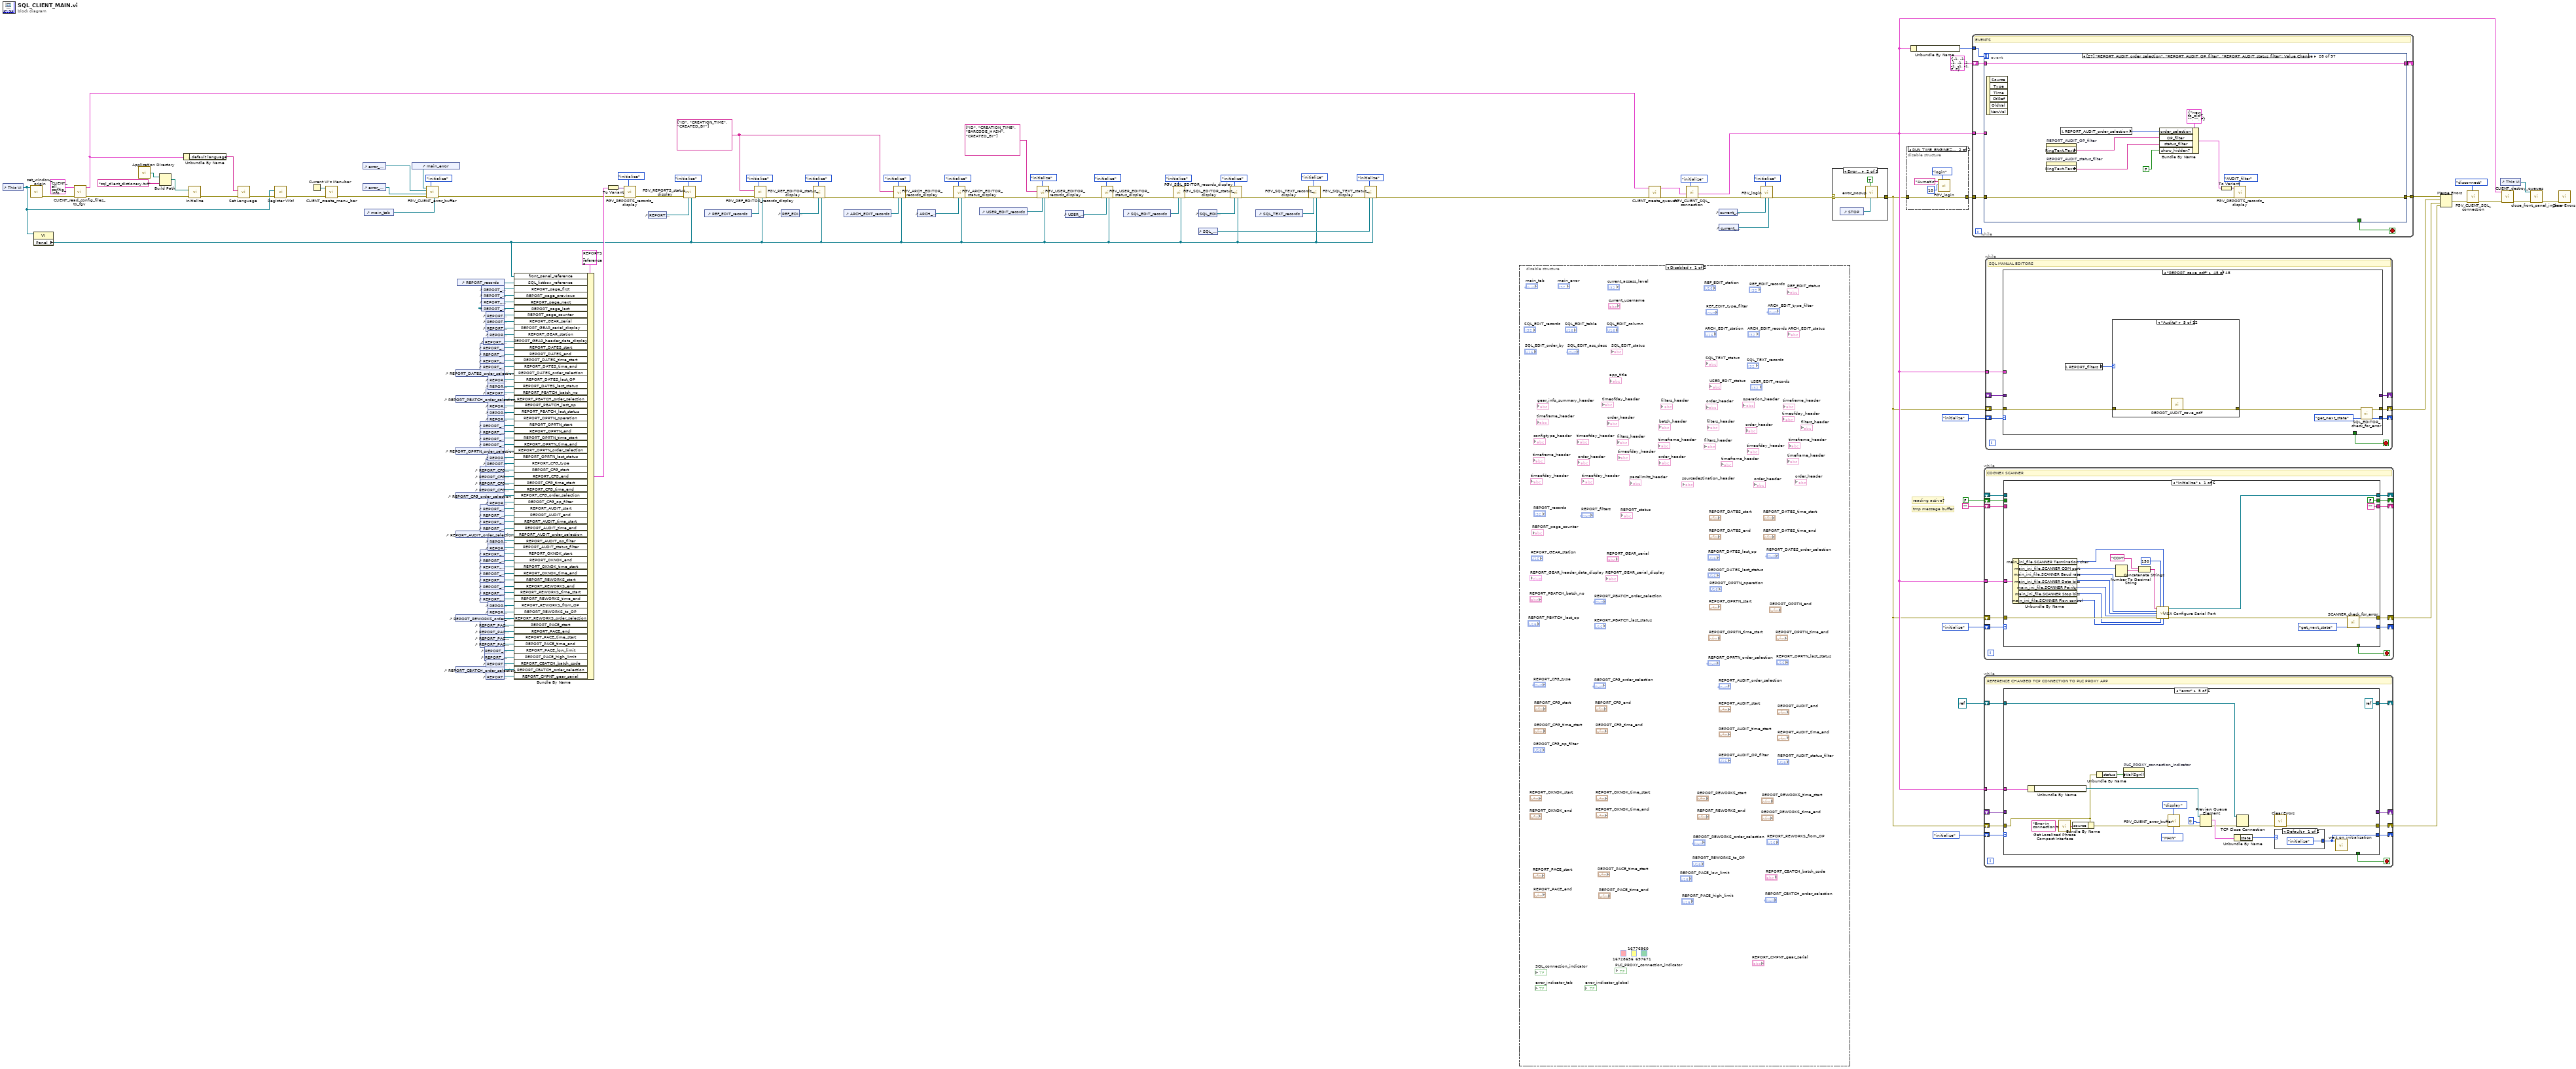
[diagram p0: block diagram]
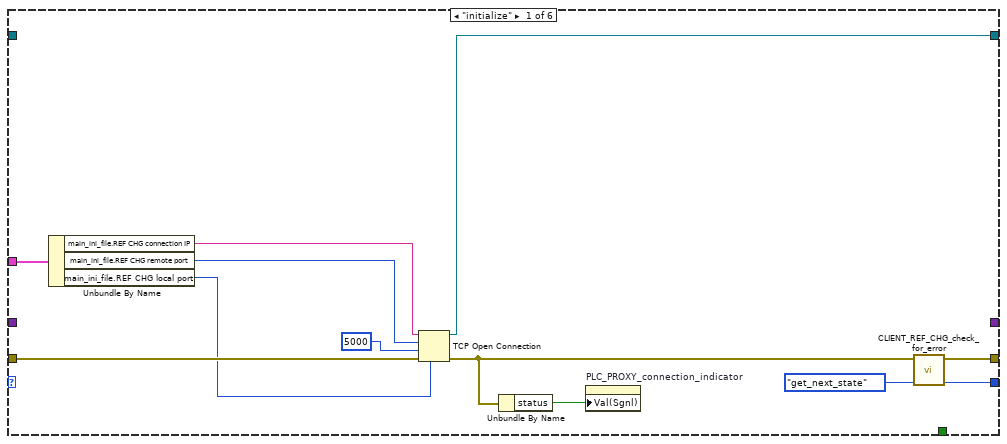
[diagram p3: hidden frame]
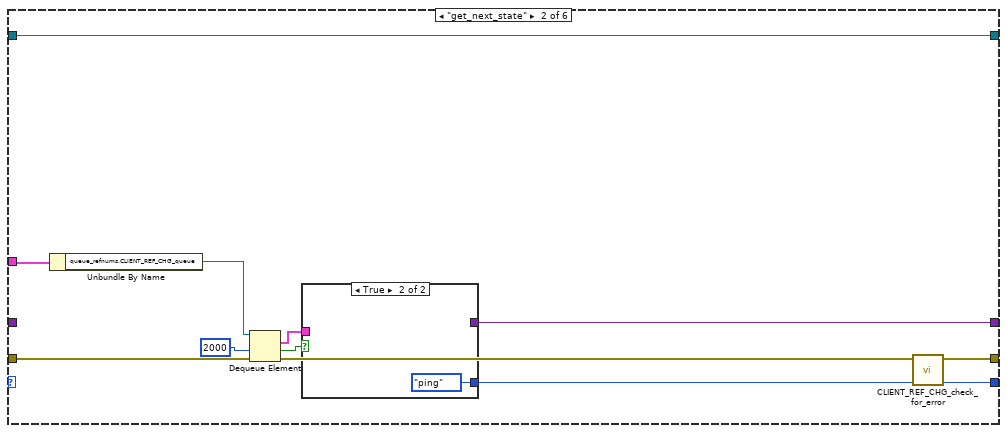
[diagram p4: hidden frame]
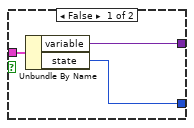
[diagram p5: hidden frame]
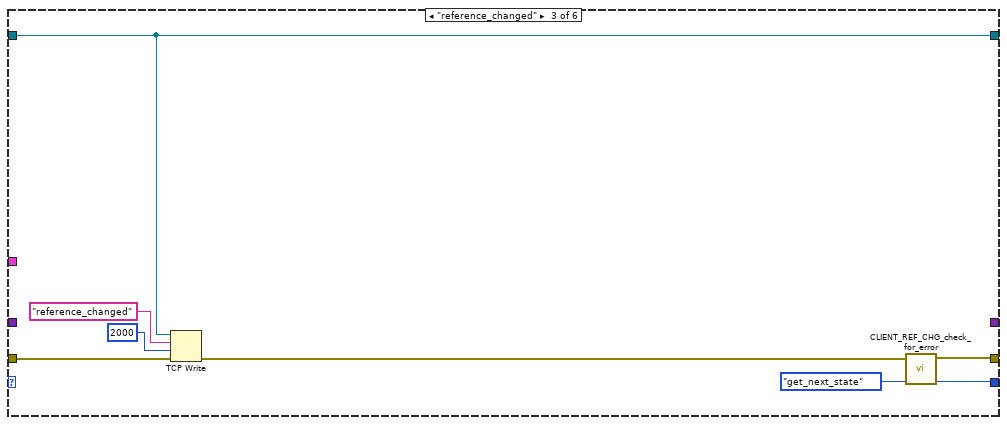
[diagram p6: hidden frame]
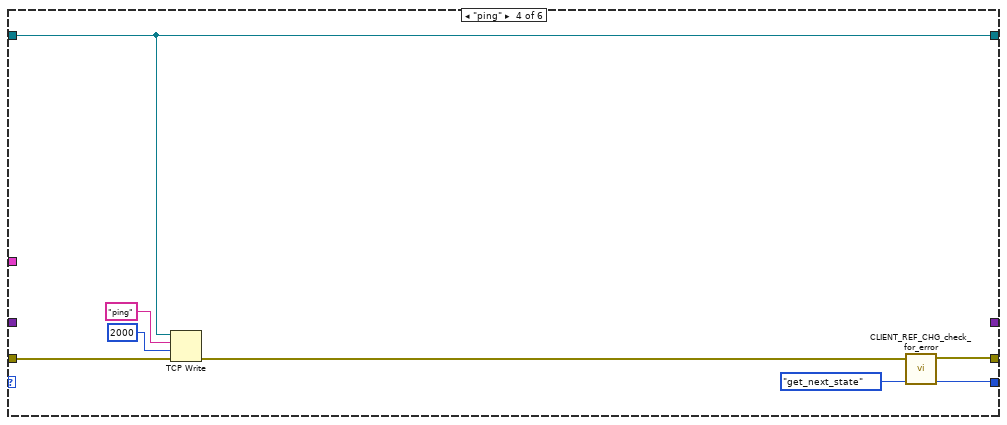
[diagram p7: hidden frame]
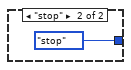
[diagram p8: hidden frame]
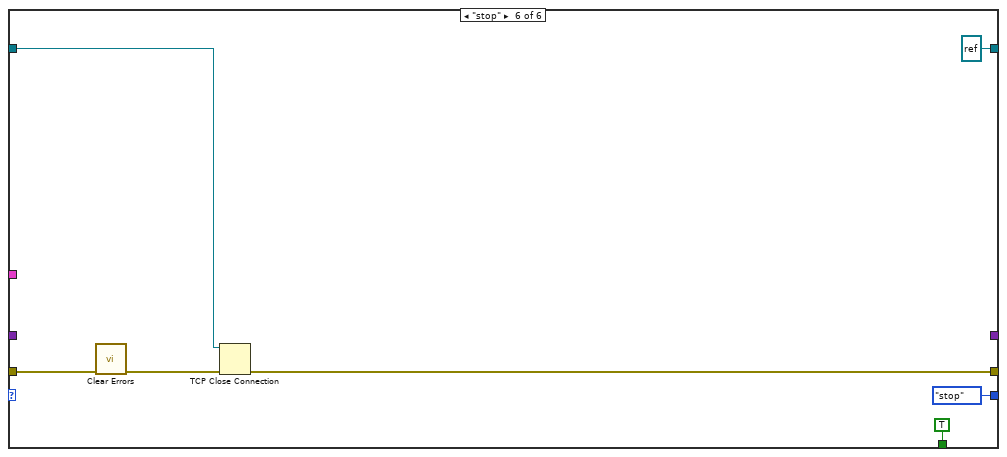
[diagram p9: hidden frame]
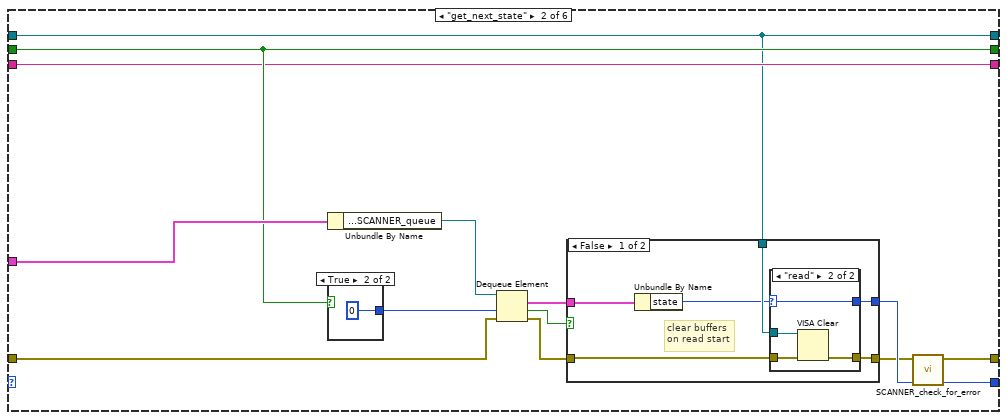
[diagram p10: hidden frame]
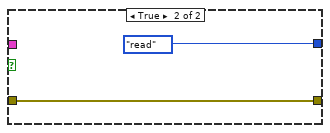
[diagram p12: hidden frame]
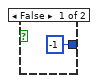
[diagram p13: hidden frame]
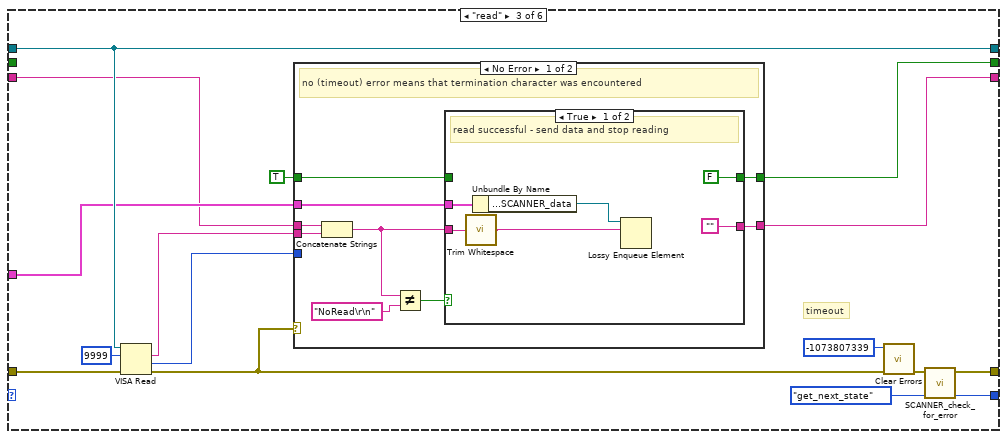
[diagram p14: hidden frame]
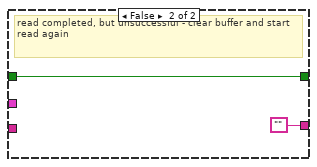
[diagram p15: hidden frame]
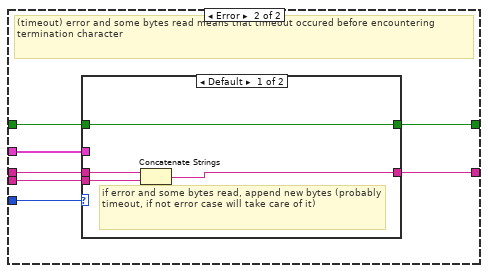
[diagram p16: hidden frame]
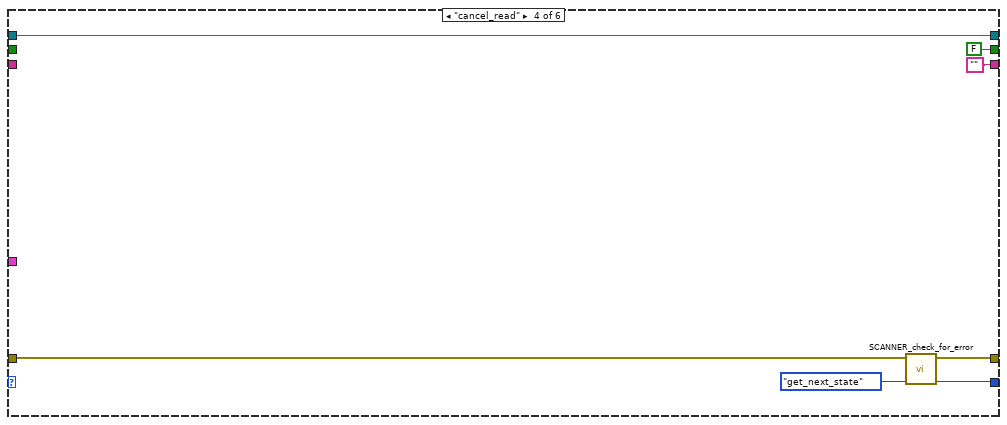
[diagram p18: hidden frame]
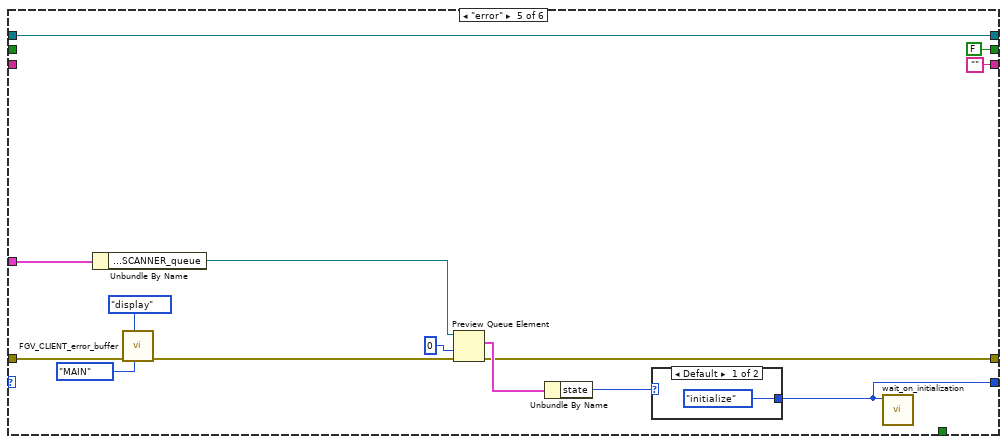
[diagram p19: hidden frame]
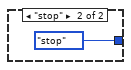
[diagram p20: hidden frame]
diagram:
  w122 = string[] ["ID", "CREATION_TIME", "CREATED_BY"]
  # "tmp message buffer"
  # "reading active?"
  n1 = control-ref of="This VI"() -> (w2:refnum<vi>)
  n2 = call "set_window_origin.vi"("this_vi_reference"=w2) -> ("error_out"=w12:errorcluster)  [unwired: 10 in]
  n3 = property class="VI"(reference=w2) -> ("Panel"=w88:refnum<vi>)  [unwired: 1 in, 2 out]
  n4 = call "CLIENT_read_config_files_to_fgv.vi"("error_in"=w12, "all_config_info_in"=T29 {"main_ini_file"={"SQL Driver"="", "SQL Server"="", "SQL Database"="", "SQL UID"="", "Reference table"="", "Reference history"="", "Archivisation CFG table"="", "Archivisation CFG history"="", "User table"="", "User history"="", "logout timeout [ms]"=0, "records per page"=0, "default language"="", "REF CHG connection IP"="", "REF CHG remote port"=0, "REF CHG local port"=0, "SCANNER COM port"=0, "SCANNER Baud rate"=0, "SCANNER Data bits"=0, "SCANNER Pairity"=enum."None", "SCANNER Stop bits"=10, "SCANNER Flow control"=0, "SCANNER Termination char"=0}, "SQL Password"="", "queue_refnums"={"SQL_EDITOR_queue"=refnum, "SCANNER_queue"=refnum, "SCANNER_data"=refnum, "CLIENT_REF_CHG_queue"=refnum}} ("all_config_info")) -> ("error_out"=w3:errorcluster, "all_config_info_out"=w1:T29)  [unwired: 8 in]
  n5 = call <vilib>:"Application Directory.vi"() -> ("Application Directory"=w10:path)
  n6 = Build Path(base path=w10, name or relative path="sql_client_dictionary.txt") -> (appended path=w8:path)
  n7 = Unbundle By Name(w1) -> ("main_ini_file.default language"=w5:string)
  n8 = call "Initialize.vi"("Dictionary File Path"=w8, "error in"=w3) -> ("error out"=w7:errorcluster)  [unwired: 8 in, 5 out]
  n9 = call "Set Language.vi"("error in"=w7, "Target Language (current lang)"=w5) -> ("error out"=w6:errorcluster)  [unwired: 8 in, 1 out]
  n10 = call-poly "Register VI(s).vi"("error in"=w6, "VI Ref"=w2) -> ("error out"=w4:errorcluster)  [unwired: 8 in, 1 out]
  n11 = Current VI's Menubar() -> (w13:refnum<k9>)
  n12 = call "CLIENT_create_menu_bar.vi"("error_in"=w4, "menu_bar_refnum"=w13) -> ("error_out"=w11:errorcluster)  [unwired: 9 in]
  n13 = control-ref of="error_indicator_tab"() -> (w120:refnum<vi>)
  n14 = control-ref of="error_indicator_global"() -> (w119:refnum<vi>)
  n15 = control-ref of="main_tab"() -> (w18:refnum<vi>)
  n16 = control-ref of="main_error"() -> (w148:refnum<vi>)
  n17 = call "FGV_CLIENT_error_buffer.vi"("main_tab"=w18, "option"=FGV_CLIENT_error_buffer."initialize", "error_in"=w11, "error_indicator_global"=w119, "error_indicator_tab"=w120, "error_display_ref"=w148) -> ("error_out"=w24:errorcluster)  [unwired: 4 in, 1 out]
  n18 = control-ref of="REPORT_DATES_order_selection"() -> (w79:refnum<vi>)
  n19 = control-ref of="REPORT_PBATCH_order_selection"() -> (w66:refnum<vi>)
  n20 = control-ref of="REPORT_OPRTN_order_selection"() -> (w59:refnum<vi>)
  n21 = control-ref of="REPORT_CFG_order_selection"() -> (w53:refnum<vi>)
  n22 = control-ref of="REPORT_AUDIT_order_selection"() -> (w46:refnum<vi>)
  n23 = control-ref of="REPORT_REWORKS_order_selection"() -> (w33:refnum<vi>)
  n24 = control-ref of="REPORT_CBATCH_order_selection"() -> (w25:refnum<vi>)
  n25 = control-ref of="REPORT_records"() -> (w89:refnum<vi>)
  n26 = control-ref of="REPORT_DATES_start"() -> (w83:refnum<vi>)
  n27 = control-ref of="REPORT_DATES_end"() -> (w82:refnum<vi>)
  n28 = control-ref of="REPORT_DATES_time_start"() -> (w81:refnum<vi>)
  n29 = control-ref of="REPORT_DATES_time_end"() -> (w80:refnum<vi>)
  n30 = control-ref of="REPORT_OPRTN_start"() -> (w63:refnum<vi>)
  n31 = control-ref of="REPORT_OPRTN_end"() -> (w62:refnum<vi>)
  n32 = control-ref of="REPORT_OPRTN_time_start"() -> (w61:refnum<vi>)
  n33 = control-ref of="REPORT_OPRTN_time_end"() -> (w60:refnum<vi>)
  n34 = control-ref of="REPORT_CFG_start"() -> (w57:refnum<vi>)
  n35 = control-ref of="REPORT_CFG_end"() -> (w56:refnum<vi>)
  n36 = control-ref of="REPORT_CFG_time_start"() -> (w55:refnum<vi>)
  n37 = control-ref of="REPORT_CFG_time_end"() -> (w54:refnum<vi>)
  n38 = control-ref of="REPORT_AUDIT_start"() -> (w50:refnum<vi>)
  n39 = control-ref of="REPORT_AUDIT_end"() -> (w49:refnum<vi>)
  n40 = control-ref of="REPORT_AUDIT_time_start"() -> (w48:refnum<vi>)
  n41 = control-ref of="REPORT_AUDIT_time_end"() -> (w47:refnum<vi>)
  n42 = control-ref of="REPORT_OKNOK_start"() -> (w43:refnum<vi>)
  n43 = control-ref of="REPORT_OKNOK_end"() -> (w42:refnum<vi>)
  n44 = control-ref of="REPORT_OKNOK_time_start"() -> (w41:refnum<vi>)
  n45 = control-ref of="REPORT_OKNOK_time_end"() -> (w40:refnum<vi>)
  n46 = control-ref of="REPORT_REWORKS_start"() -> (w39:refnum<vi>)
  n47 = control-ref of="REPORT_REWORKS_end"() -> (w38:refnum<vi>)
  n48 = control-ref of="REPORT_REWORKS_time_start"() -> (w37:refnum<vi>)
  n49 = control-ref of="REPORT_REWORKS_time_end"() -> (w36:refnum<vi>)
  n50 = control-ref of="REPORT_PACE_start"() -> (w32:refnum<vi>)
  n51 = control-ref of="REPORT_PACE_end"() -> (w31:refnum<vi>)
  n52 = control-ref of="REPORT_PACE_time_start"() -> (w30:refnum<vi>)
  n53 = control-ref of="REPORT_PACE_time_end"() -> (w29:refnum<vi>)
  n54 = control-ref of="REPORT_page_first"() -> (w72:refnum<vi>)
  n55 = control-ref of="REPORT_page_previous"() -> (w71:refnum<vi>)
  n56 = control-ref of="REPORT_page_next"() -> (w70:refnum<vi>)
  n57 = control-ref of="REPORT_page_last"() -> (w69:refnum<vi>)
  n58 = control-ref of="REPORT_GEAR_header_data_display"() -> (w87:refnum<vi>)
  n59 = control-ref of="REPORT_PACE_low_limit"() -> (w28:refnum<vi>)
  n60 = control-ref of="REPORT_PACE_high_limit"() -> (w27:refnum<vi>)
  n61 = control-ref of="REPORT_page_counter"() -> (w76:refnum<vi>)
  n62 = control-ref of="REPORT_GEAR_serial"() -> (w75:refnum<vi>)
  n63 = control-ref of="REPORT_GEAR_serial_display"() -> (w74:refnum<vi>)
  n64 = control-ref of="REPORT_PBATCH_batch_no"() -> (w65:refnum<vi>)
  n65 = control-ref of="REPORT_CFG_type"() -> (w52:refnum<vi>)
  n66 = control-ref of="REPORT_CBATCH_batch_code"() -> (w26:refnum<vi>)
  n67 = control-ref of="REPORT_CMPNT_gear_serial"() -> (w17:refnum<vi>)
  n68 = control-ref of="REPORT_GEAR_station"() -> (w73:refnum<vi>)
  n69 = control-ref of="REPORT_DATES_last_OP"() -> (w78:refnum<vi>)
  n70 = control-ref of="REPORT_DATES_last_status"() -> (w77:refnum<vi>)
  n71 = control-ref of="REPORT_PBATCH_last_op"() -> (w68:refnum<vi>)
  n72 = control-ref of="REPORT_PBATCH_last_status"() -> (w67:refnum<vi>)
  n73 = control-ref of="REPORT_OPRTN_operation"() -> (w64:refnum<vi>)
  n74 = control-ref of="REPORT_OPRTN_last_status"() -> (w58:refnum<vi>)
  n75 = control-ref of="REPORT_CFG_op_filter"() -> (w51:refnum<vi>)
  n76 = control-ref of="REPORT_AUDIT_op_filter"() -> (w45:refnum<vi>)
  n77 = control-ref of="REPORT_AUDIT_status_filter"() -> (w44:refnum<vi>)
  n78 = control-ref of="REPORT_REWORKS_from_OP"() -> (w35:refnum<vi>)
  n79 = control-ref of="REPORT_REWORKS_to_OP"() -> (w34:refnum<vi>)
  n80 = Bundle By Name(cluster=T10 {"front_panel_reference"=refnum, "SQL_listbox_reference"=refnum, "REPORT_page_first"=refnum, "REPORT_page_previous"=refnum, "REPORT_page_next"=refnum, "REPORT_page_last"=refnum, "REPORT_page_counter"=refnum, "REPORT_GEAR_serial"=refnum, "REPORT_GEAR_serial_display"=refnum, "REPORT_GEAR_station"=refnum, "REPORT_GEAR_header_data_display"=refnum, "REPORT_DATES_start"=refnum, "REPORT_DATES_end"=refnum, "REPORT_DATES_time_start"=refnum, "REPORT_DATES_time_end"=refnum, "REPORT_DATES_order_selection"=refnum, "REPORT_DATES_last_OP"=refnum, "REPORT_DATES_last_status"=refnum, "REPORT_PBATCH_batch_no"=refnum, "REPORT_PBATCH_order_selection"=refnum, "REPORT_PBATCH_last_op"=refnum, "REPORT_PBATCH_last_status"=refnum, "REPORT_OPRTN_operation"=refnum, "REPORT_OPRTN_start"=refnum, "REPORT_OPRTN_end"=refnum, "REPORT_OPRTN_time_start"=refnum, "REPORT_OPRTN_time_end"=refnum, "REPORT_OPRTN_order_selection"=refnum, "REPORT_OPRTN_last_status"=refnum, "REPORT_CFG_type"=refnum, "REPORT_CFG_start"=refnum, "REPORT_CFG_end"=refnum, "REPORT_CFG_time_start"=refnum, "REPORT_CFG_time_end"=refnum, "REPORT_CFG_order_selection"=refnum, "REPORT_CFG_op_filter"=refnum, "REPORT_AUDIT_start"=refnum, "REPORT_AUDIT_end"=refnum, "REPORT_AUDIT_time_start"=refnum, "REPORT_AUDIT_time_end"=refnum, "REPORT_AUDIT_order_selection"=refnum, "REPORT_AUDIT_op_filter"=refnum, "REPORT_AUDIT_status_filter"=refnum, "REPORT_OKNOK_start"=refnum, "REPORT_OKNOK_end"=refnum, "REPORT_OKNOK_time_start"=refnum, "REPORT_OKNOK_time_end"=refnum, "REPORT_REWORKS_start"=refnum, "REPORT_REWORKS_end"=refnum, "REPORT_REWORKS_time_start"=refnum, "REPORT_REWORKS_time_end"=refnum, "REPORT_REWORKS_from_OP"=refnum, "REPORT_REWORKS_to_OP"=refnum, "REPORT_REWORKS_order_selection"=refnum, "REPORT_PACE_start"=refnum, "REPORT_PACE_end"=refnum, "REPORT_PACE_time_start"=refnum, "REPORT_PACE_time_end"=refnum, "REPORT_PACE_low_limit"=refnum, "REPORT_PACE_high_limit"=refnum, "REPORT_CBATCH_batch_code"=refnum, "REPORT_CBATCH_order_selection"=refnum, "REPORT_CMPNT_gear_serial"=refnum} ("REPORTS_references"), "front_panel_reference"=w88, "SQL_listbox_reference"=w89, "REPORT_page_first"=w72, "REPORT_page_previous"=w71, "REPORT_page_next"=w70, "REPORT_page_last"=w69, "REPORT_page_counter"=w76, "REPORT_GEAR_serial"=w75, "REPORT_GEAR_serial_display"=w74, "REPORT_GEAR_station"=w73, "REPORT_GEAR_header_data_display"=w87, "REPORT_DATES_start"=w83, "REPORT_DATES_end"=w82, "REPORT_DATES_time_start"=w81, "REPORT_DATES_time_end"=w80, "REPORT_DATES_order_selection"=w79, "REPORT_DATES_last_OP"=w78, "REPORT_DATES_last_status"=w77, "REPORT_PBATCH_batch_no"=w65, "REPORT_PBATCH_order_selection"=w66, "REPORT_PBATCH_last_op"=w68, "REPORT_PBATCH_last_status"=w67, "REPORT_OPRTN_operation"=w64, "REPORT_OPRTN_start"=w63, "REPORT_OPRTN_end"=w62, "REPORT_OPRTN_time_start"=w61, "REPORT_OPRTN_time_end"=w60, "REPORT_OPRTN_order_selection"=w59, "REPORT_OPRTN_last_status"=w58, "REPORT_CFG_type"=w52, "REPORT_CFG_start"=w57, "REPORT_CFG_end"=w56, "REPORT_CFG_time_start"=w55, "REPORT_CFG_time_end"=w54, "REPORT_CFG_order_selection"=w53, "REPORT_CFG_op_filter"=w51, "REPORT_AUDIT_start"=w50, "REPORT_AUDIT_end"=w49, "REPORT_AUDIT_time_start"=w48, "REPORT_AUDIT_time_end"=w47, "REPORT_AUDIT_order_selection"=w46, "REPORT_AUDIT_op_filter"=w45, "REPORT_AUDIT_status_filter"=w44, "REPORT_OKNOK_start"=w43, "REPORT_OKNOK_end"=w42, "REPORT_OKNOK_time_start"=w41, "REPORT_OKNOK_time_end"=w40, "REPORT_REWORKS_start"=w39, "REPORT_REWORKS_end"=w38, "REPORT_REWORKS_time_start"=w37, "REPORT_REWORKS_time_end"=w36, "REPORT_REWORKS_from_OP"=w35, "REPORT_REWORKS_to_OP"=w34, "REPORT_REWORKS_order_selection"=w33, "REPORT_PACE_start"=w32, "REPORT_PACE_end"=w31, "REPORT_PACE_time_start"=w30, "REPORT_PACE_time_end"=w29, "REPORT_PACE_low_limit"=w28, "REPORT_PACE_high_limit"=w27, "REPORT_CBATCH_batch_code"=w26, "REPORT_CBATCH_order_selection"=w25, "REPORT_CMPNT_gear_serial"=w17) -> (w90:T10)
  n81 = To Variant(anything=w90) -> (Variant=w91:variant)
  n82 = call "FGV_REPORTS_records_display.vi"("options"=FGV_REPORTS_records_display."initialize", "error_in"=w24, "input"=w91) -> ("error_out"=w94:errorcluster)  [unwired: 7 in, 1 out]
  n83 = control-ref of="REPORT_status"() -> (w96:refnum<vi>)
  n84 = call "FGV_REPORTS_status_display.vi"("front_panel_reference"=w88, "REP_status_display_reference"=w96, "options"=FGV_REPORTS_status_display."initialize", "error_in"=w94) -> ("error_out"=w97:errorcluster)  [unwired: 7 in]
  n85 = control-ref of="REF_EDIT_records"() -> (w133:refnum<vi>)
  n86 = call "FGV_REF_EDITOR_records_display.vi"("front_panel_reference"=w88, "SQL_listbox_reference"=w133, "options"=FGV_REF_EDITOR_records_display."initialize", "error_in"=w97, "uneditable_columns"=w122) -> ("error_out"=w129:errorcluster)  [unwired: 3 in, 3 out]
  n87 = control-ref of="REF_EDIT_status"() -> (w131:refnum<vi>)
  n88 = call "FGV_REF_EDITOR_status_display.vi"("front_panel_reference"=w88, "REF_status_display_reference"=w131, "options"=FGV_REF_EDITOR_status_display."initialize", "error_in"=w129) -> ("error_out"=w126:errorcluster)  [unwired: 7 in]
  n89 = control-ref of="ARCH_EDIT_records"() -> (w123:refnum<vi>)
  n90 = call "FGV_ARCH_EDITOR_records_display.vi"("front_panel_reference"=w88, "SQL_listbox_reference"=w123, "options"=FGV_ARCH_EDITOR_records_display."initialize", "error_in"=w126, "uneditable_columns"=w122) -> ("error_out"=w125:errorcluster)  [unwired: 3 in, 3 out]
  n91 = control-ref of="ARCH_EDIT_status"() -> (w127:refnum<vi>)
  n92 = call "FGV_ARCH_EDITOR_status_display.vi"("front_panel_reference"=w88, "ARCH_status_display_reference"=w127, "options"=FGV_ARCH_EDITOR_status_display."initialize", "error_in"=w125) -> ("error_out"=w106:errorcluster)  [unwired: 7 in]
  n93 = control-ref of="USER_EDIT_records"() -> (w103:refnum<vi>)
  n94 = call "FGV_USER_EDITOR_records_display.vi"("front_panel_reference"=w88, "SQL_listbox_reference"=w103, "options"=FGV_USER_EDITOR_records_display."initialize", "error_in"=w106, "uneditable_columns"=string[] ["ID", "CREATION_TIME", "BARCODE_HASH", "CREATED_BY"]) -> ("error_out"=w105:errorcluster)  [unwired: 3 in, 3 out]
  n95 = control-ref of="USER_EDIT_status"() -> (w107:refnum<vi>)
  n96 = call "FGV_USER_EDITOR_status_display.vi"("front_panel_reference"=w88, "USER_status_display_reference"=w107, "options"=FGV_USER_EDITOR_status_display."initialize", "error_in"=w105) -> ("error_out"=w109:errorcluster)  [unwired: 7 in]
  n97 = control-ref of="SQL_EDIT_records"() -> (w143:refnum<vi>)
  n98 = call "FGV_SQL_EDITOR_records_display.vi"("front_panel_reference"=w88, "SQL_listbox_reference"=w143, "options"=FGV_SQL_EDITOR_records_display."initialize", "error_in"=w109) -> ("error_out"=w141:errorcluster)  [unwired: 4 in, 3 out]
  n99 = control-ref of="SQL_EDIT_status"() -> (w140:refnum<vi>)
  n100 = control-ref of="SQL_TEXT_status"() -> (w114:refnum<vi>)
  n101 = call "FGV_SQL_EDITOR_status_display.vi"("front_panel_reference"=w88, "SQL_status_display_reference"=w140, "options"=FGV_SQL_EDITOR_status_display."initialize", "error_in"=w141) -> ("error_out"=w113:errorcluster)  [unwired: 7 in]
  n102 = control-ref of="SQL_TEXT_records"() -> (w110:refnum<vi>)
  n103 = call "FGV_SQL_TEXT_records_display.vi"("front_panel_reference"=w88, "SQL_listbox_reference"=w110, "options"=FGV_SQL_TEXT_records_display."initialize", "error_in"=w113) -> ("error_out"=w112:errorcluster)  [unwired: 7 in]
  n104 = call "FGV_SQL_TEXT_status_display.vi"("front_panel_reference"=w88, "SQL_status_display_reference"=w114, "options"=FGV_SQL_TEXT_status_display."initialize", "error_in"=w112) -> ("error_out"=w23:errorcluster)  [unwired: 7 in]
  n105 = disable-structure shown="Disabled" {
    frame Disabled {
      (unwired) u32 16728656
      (unwired) u32 16776960
      (unwired) u32 697671
    }
    frame Enabled {
    }
  }
  n106 = call "CLIENT_create_queues.vi"("error_in"=w23, "all_config_info_in"=w1) -> ("error_out"=w121:errorcluster, "all_config_info_out"=w86:T29)  [unwired: 8 in]
  n107 = call "FGV_CLIENT_SQL_connection.vi"("options"=FGV_CLIENT_SQL_connection."initialize", "error_in"=w121, "all_config_info_in"=w86) -> ("error_out"=w101:errorcluster, "all_config_info_out"=w21:T29)  [unwired: 4 in, 3 out]
  n108 = control-ref of="current_username"() -> (w99:refnum<vi>)
  n109 = control-ref of="current_access_level"() -> (w98:refnum<vi>)
  n110 = call "FGV_login.vi"("current_access_level"=w98, "current_username"=w99, "options"=FGV_login."initialize", "error_in"=w101) -> ("error_out"=w16:errorcluster)  [unwired: 5 in, 2 out]
  n111 = case shown="Error .." w16 {
    selector: w16 -> [w153 w156]
    tunnel: [w153 w157] -> w15
    frame No Error {
    }
    frame Error {
      n112 = control-ref of="STOP"() -> (w155:refnum<vi>)
      n113 = call "error_popup.vi"("STOP_button_reference"=w155, "EXIT App If Error? (F)"=TRUE, "error_in"=w156) -> ("error_out"=w157:errorcluster)  [unwired: 8 in]
    }
  }
  n114 = disable-structure shown="RUN_TIME_ENGINE==False" {
    disable-tunnel: w15 -> [w158 w159]
    disable-tunnel: [w158 w159] -> w14
    frame condition #0 {
    }
    frame condition #1 (active) {
      n115 = call "FGV_login.vi"("options"=FGV_login."login", "access_level_in"=10, "username_in"="Aumatic") -> ()  [unwired: 6 in, 3 out]
    }
  }
  n116 = Unbundle By Name(w21) -> ("main_ini_file.logout timeout [ms]"=w84:i32)
  n117 = while {
    tunnel: w14 -> [w168]
    tunnel: [w169] -> w146
    tunnel: w21 -> [w166]
    shift-right: [w165] -> _
    shift-left: T21 {"REF_EDIT_clicked_row"=-1, "REF_EDIT_selected_row"=-1, "SQL_EDIT_clicked_row"=-1, "SQL_EDIT_selected_row"=-1, "ARCH_EDIT_selected_row"=-1, "ARCH_EDIT_clicked_row"=-1, "USER_EDIT_selected_row"=-1, "USER_EDIT_clicked_row"=-1, "REPORT_GEAR_toggle_all_results"=FALSE, "REPORT_AUDIT_toggle_all_results"=FALSE} -> [w164]
    tunnel: w84 -> [w163]
    stop <- w167 stop-if-true
    # "EVENTS"
    n118 = event shown="[27] \"REPORT_AUDIT_order_selection\", \"REPORT_AUDIT_OP_filter\", \"REPORT_AUDIT_status_filter\": Value Change" {
      selector: _ -> [_ _ _ _ _ _ _ _ _ _ _ _ _ _ _ _ _ _ _ _ _ _ _ _ _ _ _ _ _ _ _ _ _ _ _ _ _ _ _ _ _ _ _ _ _ _ _ _ _ _ _ _ _ _ _ _ _ _ _ _ _ _ _ _ _ _ _ _ _ _ _ _ _ _ _ _ _ _ _ _ _ _ _ _ _ _ _ _ _ _ _ _ _ _ _ _ _]
      dyn-events: _ -> [_ _ _ _ _ _ _ _ _ _ _ _ _ _ _ _ _ _ _ _ _ _ _ _ _ _ _ _ _ _ _ _ _ _ _ _ _ _ _ _ _ _ _ _ _ _ _ _ _ _ _ _ _ _ _ _ _ _ _ _ _ _ _ _ _ _ _ _ _ _ _ _ _ _ _ _ _ _ _ _ _ _ _ _ _ _ _ _ _ _ _ _ _ _ _ _ _]
      timeout: w163 -> [_ _ _ _ _ _ _ _ _ _ _ _ _ _ _ _ _ _ _ _ _ _ _ _ _ _ _ _ _ _ _ _ _ _ _ _ _ _ _ _ _ _ _ _ _ _ _ _ _ _ _ _ _ _ _ _ _ _ _ _ _ _ _ _ _ _ _ _ _ _ _ _ _ _ _ _ _ _ _ _ _ _ _ _ _ _ _ _ _ _ _ _ _ _ _ _ _]
      tunnel: [_ _ _ _ _ _ _ _ _ _ _ _ _ _ _ _ _ _ _ _ _ _ _ _ _ _ _ _ _ _ _ _ _ _ _ _ _ _ _ _ _ _ _ _ _ _ _ _ _ _ _ _ _ _ _ _ _ _ _ _ _ _ _ _ _ _ _ _ _ _ _ _ _ _ _ _ _ _ _ _ _ _ w1580 _ _ _ _ _ _ _ _ _ _ _ _ _ _] -> w167
      tunnel: w168 -> [w172 w177 w192 w204 w239 w251 w261 w325 w333 w342 w355 w364 w377 w383 w391 w396 w411 w423 w454 w466 w473 w606 w671 w679 w688 w702 w709 w721 w726 w730 w773 w779 w794 w804 w809 w815 w855 w870 w881 w886 w890 w931 w945 w953 w983 w1064 w1070 w1076 w1082 w1100 w1105 w1112 w1124 w1130 w1134 w1164 w1194 w1224 w1261 w1267 w1329 w1335 w1342 w1347 w1353 w1359 w1366 w1370 w1376 w1382 w1397 w1409 w1447 w1451 w1463 w1471 w1536 w1546 w1552 w1562 w1572 w1577 w1583 w1617 w1623 w1638 w1650 w1685 w1697 w1707 w1771 w1779 w1785 w1811 w1839 w1861 w1864]
      tunnel: [w171 w176 w191 w203 w239 w251 w261 w325 w336 w347 w358 w363 w377 w383 w390 w395 w410 w422 w454 w466 w473 w606 w671 w682 w693 w704 w709 w720 w726 w729 w772 w780 w794 w803 w809 w814 w856 w870 w880 w886 w889 w932 w946 w954 w982 w1064 w1070 w1076 w1080 w1099 w1105 w1119 w1124 w1130 w1133 w1163 w1193 w1223 w1260 w1268 w1329 w1335 w1341 w1347 w1352 w1358 w1365 w1369 w1375 w1381 w1396 w1408 w1446 w1451 w1463 w1471 w1536 w1546 w1555 w1566 w1568 w1576 w1584 w1616 w1622 w1637 w1649 w1685 w1697 w1707 w1771 w1782 w1786 w1814 w1839 w1861 w1863] -> w169
      tunnel: w166 -> [_ w175 _ w202 _ _ _ _ w337 w348 w359 _ _ _ _ w394 _ w421 _ _ _ _ _ w683 w694 w705 _ _ _ _ _ w778 _ _ _ w813 w854 _ _ _ _ w930 _ _ w981 _ _ _ _ _ _ _ _ _ _ _ _ _ _ w1265 _ _ _ _ w1351 w1357 _ _ _ w1380 _ w1407 _ _ _ _ _ _ w1556 w1567 _ w1575 w1586 _ w1621 _ w1648 _ _ _ _ w1783 w1784 w1813 _ _ _]
      tunnel: [w173 w178 w194 w205 w238 w250 w265 w320 w334 w343 w356 w366 w375 w384 w392 w397 w413 w424 w453 w465 w478 w610 w667 w680 w689 w703 w710 w722 w727 w731 w774 w781 w795 w805 w810 w812 w857 w871 w882 w887 w892 w933 w948 w950 w979 w1065 w1071 w1077 w1083 w1101 w1106 w1120 w1125 w1131 w1136 w1166 w1196 w1226 w1262 w1263 w1331 w1336 w1343 w1348 w1355 w1361 w1363 w1368 w1372 w1383 w1399 w1410 w1443 w1450 w1462 w1475 w1532 w1543 w1548 w1558 w1573 w1579 w1585 w1619 w1624 w1640 w1651 w1684 w1696 w1711 w1766 w1780 w1788 w1815 w1838 w1858 w1865] -> w165
      tunnel: w164 -> [w173 w178 w194 w205 w238 w250 w265 w322 w334 w343 w356 w366 w375 w384 w392 w397 w413 w424 w453 w465 w478 w610 w664 w680 w689 w703 w710 w722 w727 w732 w774 w781 w795 w805 w810 w812 w857 w871 w882 w887 w892 w933 w948 w951 w980 w1065 w1071 w1077 w1083 w1101 w1106 w1120 w1125 w1131 w1136 w1166 w1196 w1226 w1262 w1264 w1331 w1336 w1343 w1348 w1355 w1361 w1363 w1368 w1372 w1383 w1399 w1410 w1443 w1450 w1462 w1475 w1530 w1545 w1548 w1558 w1573 w1579 w1585 w1619 w1624 w1640 w1651 w1684 w1696 w1711 w1768 w1780 w1788 w1815 w1838 w1858 w1865]
      event "ARCH_EDIT_clear_status": Value Change {
        n119 = event-data() -> ()  [unwired: 1 in, 6 out]
        n120 = call "FGV_ARCH_EDITOR_status_display.vi"("options"=FGV_ARCH_EDITOR_status_display."clear", "error_in"=w172) -> ("error_out"=w171:errorcluster)  [unwired: 9 in]
      }
      event "ARCH_EDIT_delete": Value Change {
        n121 = event-data() -> ()  [unwired: 1 in, 6 out]
        n122 = local read "ARCH_EDIT_records"() -> (w174:i32)
        n123 = case shown="-1" w174 {
          tunnel: w177 -> [_ w189]
          tunnel: [w185 w188] -> w176
          tunnel: w175 -> [_ w187]
          frame -1 {
            n124 = call-poly "Get Localized Phrase Compact Interface.vi"("Key"="No record selected for DELETE" ("source")) -> ("Translated Phrase"=w179:string)
            n125 = Bundle By Name(cluster=errorcluster {"status"=FALSE, "code"=503, "source"=""} ("error out"), "source"=w179) -> (w181:errorcluster)
            n126 = call "FGV_ARCH_EDITOR_status_display.vi"("options"=FGV_ARCH_EDITOR_status_display."display", "error_in"=w181, "display_source"="DELETE") -> ("error_out"=w185:errorcluster)  [unwired: 8 in]
          }
          frame Default {
            n127 = Unbundle By Name(w187) -> ("queue_refnums.SQL_EDITOR_queue"=w190:refnum<queue>)
            n128 = Enqueue Element(queue=w190, element=T32 {"state"=enum."ARCH_delete_record", "variable"=variant}, error in (no error)=w189) -> (error out=w188:errorcluster)  [unwired: 1 in, 2 out]
          }
        }
      }
      event "ARCH_EDIT_discard": Value Change {
        n129 = event-data() -> ()  [unwired: 1 in, 6 out]
        n130 = local read "ARCH_EDIT_records"() -> (w193:i32)
        n131 = case shown="Default" w193 {
          selector: w193 -> [_ w200]
          tunnel: w192 -> [w195 w198]
          tunnel: [w195 w197] -> w191
          frame -1 {
          }
          frame Default {
            n132 = To Variant(anything=w200) -> (Variant=w199:variant)
            n133 = call "FGV_ARCH_EDITOR_records_display.vi"("options"=FGV_ARCH_EDITOR_records_display."discard_changes", "error_in"=w198, "input"=w199) -> ("error_out"=w197:errorcluster)  [unwired: 5 in, 3 out]
          }
        }
      }
      event "ARCH_EDIT_insert_update": Value Change {
        n134 = event-data() -> ()  [unwired: 1 in, 6 out]
        n135 = local read "ARCH_EDIT_records"() -> (w201:i32)
        n136 = case shown="Default" w201 {
          selector: w201 -> [_ w216]
          tunnel: w204 -> [_ w220]
          tunnel: [w211 w219] -> w203
          tunnel: w202 -> [_ w218]
          frame -1 {
            n137 = call-poly "Get Localized Phrase Compact Interface.vi"("Key"="No record selected for INSERT / UPDATE" ("source")) -> ("Translated Phrase"=w206:string)
            n138 = Bundle By Name(cluster=errorcluster {"status"=FALSE, "code"=503, "source"=""} ("error out"), "source"=w206) -> (w209:errorcluster)
            n139 = call "FGV_ARCH_EDITOR_status_display.vi"("options"=FGV_ARCH_EDITOR_status_display."display", "error_in"=w209, "display_source"="INSERT / UPDATE") -> ("error_out"=w211:errorcluster)  [unwired: 8 in]
          }
          frame Default {
            n140 = call "FGV_ARCH_EDITOR_records_display.vi"("options"=FGV_ARCH_EDITOR_records_display."get_all_info") -> ("all_info"=w214:T43)  [unwired: 7 in, 3 out]
            n141 = Unbundle By Name(w214) -> ("ARCH_record_states"=w217:T44[])
            n142 = Index Array(array=w217, index=w216) -> (element=w215:T44)
            n143 = case shown="\"Equal\"" w215 {
              tunnel: w220 -> [_ w231 w236]
              tunnel: [w227 w230 w235] -> w219
              tunnel: w218 -> [_ w229 w234]
              frame "Equal" {
                n144 = call-poly "Get Localized Phrase Compact Interface.vi"("Key"="Record is already up to date with database" ("source")) -> ("Translated Phrase"=w223:string)
                n145 = Bundle By Name(cluster=errorcluster {"status"=FALSE, "code"=502, "source"=""} ("error out"), "source"=w223) -> (w221:errorcluster)
                n146 = call "FGV_ARCH_EDITOR_status_display.vi"("options"=FGV_ARCH_EDITOR_status_display."display", "error_in"=w221, "display_source"="INSERT / UPDATE") -> ("error_out"=w227:errorcluster)  [unwired: 8 in]
              }
              frame "Added", "Deleted" {
                n147 = Unbundle By Name(w229) -> ("queue_refnums.SQL_EDITOR_queue"=w232:refnum<queue>)
                n148 = Enqueue Element(queue=w232, element=T32 {"state"=enum."ARCH_insert_record", "variable"=variant}, error in (no error)=w231) -> (error out=w230:errorcluster)  [unwired: 1 in, 2 out]
              }
              frame "Edited" {
                n149 = Unbundle By Name(w234) -> ("queue_refnums.SQL_EDITOR_queue"=w237:refnum<queue>)
                n150 = Enqueue Element(queue=w237, element=T32 {"state"=enum."ARCH_update_record", "variable"=variant}, error in (no error)=w236) -> (error out=w235:errorcluster)  [unwired: 1 in, 2 out]
              }
            }
          }
        }
      }
      event "ARCH_EDIT_records": Double Click {
        # "Workaround for delay of editting multicolumn listbox (without this editting possible after two clicks with 1sec. break between them)"
        n151 = event-data() -> ("CtlRef"=w241:refnum<vi>, "Coords"=w240:T45)  [unwired: 1 in, 4 out]
        n152 = invoke class="MCListbox (strict)" method="Point To Row Column"(reference=w241, "Point"=w240) -> (reference out=w244:refnum<vi>, error out=w243:errorcluster, "CellPosition"=w242:T36)  [unwired: 5 in, 4 out]
        n153 = property class="MCListbox (strict)"(reference=w244, error in=w243, "EditPos"=w242) -> ()  [unwired: 2 out]
      }
      event "ARCH_EDIT_records": Edit Cell {
        n154 = event-data() -> ("Coords.Row"=w245:i32)  [unwired: 1 in]
        n155 = call "FGV_ARCH_EDITOR_records_display.vi"("options"=FGV_ARCH_EDITOR_records_display."get_all_info") -> ("all_info"=w247:T43)  [unwired: 7 in, 3 out]
        n156 = Unbundle By Name(w247) -> ("size.SQL_rows"=w248:i32)
        n157 = local write "ARCH_EDIT_records"(w245) -> ()
        n158 = Greater Or Equal?(x=w245, y=w248) -> (x >= y?=w249:bool)
        n159 = case shown="True" w249 {
          tunnel: w245 -> [w254 w257]
          frame False {
            n160 = To Variant(anything=w254) -> (Variant=w253:variant)
            n161 = call "FGV_ARCH_EDITOR_records_display.vi"("options"=FGV_ARCH_EDITOR_records_display."record_edited?", "input"=w253) -> ()  [unwired: 6 in, 4 out]
          }
          frame True {
            n162 = To Variant(anything=w257) -> (Variant=w256:variant)
            n163 = call "FGV_ARCH_EDITOR_records_display.vi"("options"=FGV_ARCH_EDITOR_records_display."record_added?", "input"=w256) -> ()  [unwired: 6 in, 4 out]
          }
        }
      }
      event "ARCH_EDIT_records": Key Down? {
        n164 = event-data() -> ("CtlRef"=w262:refnum<vi>, "ScanCode"=w264:i16, "PlatMods.Shift"=w260:bool)  [unwired: 1 in, 1 out]
        n165 = call "FGV_ARCH_EDITOR_records_display.vi"("options"=FGV_ARCH_EDITOR_records_display."get_all_info") -> ("all_info"=w258:T43)  [unwired: 7 in, 3 out]
        n166 = case shown="72" w264 {
          tunnel: [_ TRUE w273 w284 w295 w306] -> w263
          tunnel: w262 -> [_ w270 w275 w286 w297 w308]
          tunnel: w260 -> [_ _ w274 w285 w296 w307]
          tunnel: w258 -> [_ w266 w272 w283 w294 w305]
          frame Default {
          }
          frame 15 {
            # "15 = Tab"
            n167 = Unbundle By Name(w266) -> ("editable_columns"=w268:i32[], "size.SQL_rows"=w267:i32)
            n168 = call "EDITORS_calculate_next_pos_for_keyboard_events.vi"("direction"=directions."RIGHT", "SQL_rows"=w267, "editable_columns"=w268, "reference"=w270) -> ()  [unwired: 8 in]
          }
          frame 75 {
            # "75 = Left Arrow"
            n169 = case shown="True" w274 {
              tunnel: w275 -> [_ w282]
              tunnel: [FALSE TRUE] -> w273
              tunnel: w272 -> [_ w277]
              frame False {
              }
              frame True {
                n170 = Unbundle By Name(w277) -> ("editable_columns"=w279:i32[], "size.SQL_rows"=w278:i32)
                n171 = call "EDITORS_calculate_next_pos_for_keyboard_events.vi"("direction"=directions."LEFT", "SQL_rows"=w278, "editable_columns"=w279, "reference"=w282) -> ()  [unwired: 8 in]
              }
            }
          }
          frame 77 {
            # "77 = Right Arrow"
            n172 = case shown="True" w285 {
              tunnel: w286 -> [_ w293]
              tunnel: [FALSE TRUE] -> w284
              tunnel: w283 -> [_ w288]
              frame False {
              }
              frame True {
                n173 = Unbundle By Name(w288) -> ("editable_columns"=w290:i32[], "size.SQL_rows"=w289:i32)
                n174 = call "EDITORS_calculate_next_pos_for_keyboard_events.vi"("direction"=directions."RIGHT", "SQL_rows"=w289, "editable_columns"=w290, "reference"=w293) -> ()  [unwired: 8 in]
              }
            }
          }
          frame 72 {
            # "72 = Up Arrow"
            n175 = case shown="True" w296 {
              tunnel: w297 -> [_ w304]
              tunnel: [FALSE TRUE] -> w295
              tunnel: w294 -> [_ w299]
              frame False {
              }
              frame True {
                n176 = Unbundle By Name(w299) -> ("editable_columns"=w301:i32[], "size.SQL_rows"=w300:i32)
                n177 = call "EDITORS_calculate_next_pos_for_keyboard_events.vi"("direction"=directions."UP", "SQL_rows"=w300, "editable_columns"=w301, "reference"=w304) -> ()  [unwired: 8 in]
              }
            }
          }
          frame 80 {
            # "80 = Down Arrow"
            n178 = case shown="True" w307 {
              tunnel: w308 -> [_ w315]
              tunnel: [FALSE TRUE] -> w306
              tunnel: w305 -> [_ w310]
              frame False {
              }
              frame True {
                n179 = Unbundle By Name(w310) -> ("editable_columns"=w312:i32[], "size.SQL_rows"=w311:i32)
                n180 = call "EDITORS_calculate_next_pos_for_keyboard_events.vi"("direction"=directions."DOWN", "SQL_rows"=w311, "editable_columns"=w312, "reference"=w315) -> ()  [unwired: 8 in]
              }
            }
          }
        }
        n181 = event-data("Discard?"=w263) -> ()  [unwired: 1 in, 1 out]
      }
      event "ARCH_EDIT_records": Mouse Down? {
        n182 = event-data() -> ("CtlRef"=w324:refnum<vi>, "Coords"=w323:T45)  [unwired: 1 in]
        n183 = invoke class="MCListbox (strict)" method="Point To Row Column"(reference=w324, "Point"=w323) -> ("InBounds"=w316:bool, "CellPosition"=w318:T36)  [unwired: 5 in, 5 out]
        n184 = local read "ARCH_EDIT_records"() -> (w321:i32)
        n185 = Bundle By Name(cluster=w322, "ARCH_EDIT_selected_row"=w321) -> (w319:T21)
        n186 = case shown="True" w316 {
          selector: w316 -> [w327 _]
          tunnel: [w326 w331] -> w320
          tunnel: w319 -> [w326 w330]
          tunnel: w318 -> [_ w329]
          tunnel: [w327 w328] -> w317
          frame False {
          }
          frame True {
            n187 = call "ARCH_EDITOR_records_click_discard.vi"("CellPosition"=w329, "event_structure_shift_register_in"=w330) -> ("Discard?"=w328:bool, "event_structure_shift_register_out"=w331:T21)  [unwired: 8 in]
          }
        }
        n188 = event-data("Discard?"=w317) -> ()  [unwired: 1 in, 1 out]
      }
      event "ARCH_EDIT_refresh": Value Change {
        n189 = event-data() -> ()  [unwired: 1 in, 6 out]
        n190 = Unbundle By Name(w337) -> ("queue_refnums.SQL_EDITOR_queue"=w335:refnum<queue>)
        n191 = Enqueue Element(queue=w335, element=T32 {"state"=enum."ARCH_read_stations", "variable"=variant}, error in (no error)=w333) -> (error out=w336:errorcluster)  [unwired: 1 in, 2 out]
      }
      event "ARCH_EDIT_station": Value Change {
        n192 = event-data() -> ("CtlRef"=w345:refnum<vi>)  [unwired: 1 in, 5 out]
        n193 = property class="Ring (strict)"(reference=w345) -> ("RingText.Text"=w344:string)  [unwired: 1 in, 2 out]
        n194 = To Variant(anything=w344) -> (Variant=w340:variant)
        n195 = call "FGV_ARCH_EDITOR_records_display.vi"("options"=FGV_ARCH_EDITOR_records_display."set_station_number", "error_in"=w342, "input"=w340) -> ("error_out"=w341:errorcluster)  [unwired: 5 in, 3 out]
        n196 = Unbundle By Name(w348) -> ("queue_refnums.SQL_EDITOR_queue"=w346:refnum<queue>)
        n197 = Enqueue Element(queue=w346, element=T32 {"state"=enum."ARCH_select_station_records", "variable"=variant}, error in (no error)=w341) -> (error out=w347:errorcluster)  [unwired: 1 in, 2 out]
      }
      event Value Change {
        n198 = event-data() -> ("NewVal"=w350:T8)  [unwired: 1 in, 5 out]
        n199 = Format Into String(w350) -> (resulting string=w349:string)  [unwired: 3 in, 1 out]
        n200 = To Variant(anything=w349) -> (Variant=w353:variant)
        n201 = call "FGV_ARCH_EDITOR_records_display.vi"("options"=FGV_ARCH_EDITOR_records_display."set_type_filter", "error_in"=w355, "input"=w353) -> ("error_out"=w354:errorcluster)  [unwired: 5 in, 3 out]
        n202 = Unbundle By Name(w359) -> ("queue_refnums.SQL_EDITOR_queue"=w357:refnum<queue>)
        n203 = Enqueue Element(queue=w357, element=T32 {"state"=enum."ARCH_select_station_records", "variable"=variant}, error in (no error)=w354) -> (error out=w358:errorcluster)  [unwired: 1 in, 2 out]
      }
      event "current_access_level": Value Change {
        n204 = event-data() -> ("NewVal"=w365:i32)  [unwired: 1 in]
        n205 = case shown="7..9" w365 {
          tunnel: w364 -> [w368 w370 w372 w374]
          tunnel: [w368 w370 w372 w374] -> w363
          tunnel: [w367 w369 w371 w373] -> w361
          frame Default {
            w367 = T46 [enum."Errors"] items=["Reports", "Reference Editor", "Archivisation Editor", "User Management", "Manual SQL Requests", "Text SQL Requests", "Errors"]
          }
          frame 1..6 {
            w369 = T46 [enum."Errors", enum."Reports"] items=["Reports", "Reference Editor", "Archivisation Editor", "User Management", "Manual SQL Requests", "Text SQL Requests", "Errors"]
          }
          frame 7..9 {
            w371 = T46 [enum."Errors", enum."Reports", enum."Reference Editor", enum."Archivisation Editor"] items=["Reports", "Reference Editor", "Archivisation Editor", "User Management", "Manual SQL Requests", "Text SQL Requests", "Errors"]
          }
          frame 10 {
            w373 = T46 [enum."Errors", enum."Reports", enum."Reference Editor", enum."Archivisation Editor", enum."User Management", enum."Manual SQL Requests", enum."Text SQL Requests"] items=["Reports", "Reference Editor", "Archivisation Editor", "User Management", "Manual SQL Requests", "Text SQL Requests", "Errors"]
          }
        }
        n206 = control-ref of="main_tab"() -> (w360:refnum<vi>)
        n207 = control-ref of="This VI"() -> (w362:refnum<vi>)
        n208 = call "CLIENT_show_hide_pages.vi"("This VI"=w362, "visible_pages"=w361, "main_tab_ref"=w360) -> ()  [unwired: 9 in]
      }
      event "ERRORS_clear": Value Change {
        n209 = event-data() -> ()  [unwired: 1 in, 6 out]
        n210 = call "FGV_CLIENT_error_buffer.vi"("option"=FGV_CLIENT_error_buffer."clear") -> ()  [unwired: 9 in, 2 out]
      }
      event "PLC_PROXY_connection_indicator": Value Change {
        n211 = event-data() -> ("NewVal"=w382:bool)  [unwired: 1 in]
        n212 = control-ref of="main_tab"() -> (w381:refnum<vi>)
        n213 = property class="TabCtl (strict)"(reference=w381) -> ("Pages"=w380:refnum<vi>[])  [unwired: 1 in, 2 out]
        n214 = Index Array(array=w380, index=T1."Reference Editor" ("main_tab")) -> (element=w378:refnum<vi>)
        n215 = case shown="True" w382 {
          tunnel: w378 -> [w386 w388]
          frame True {
            n216 = property class="Page"(reference=w386, "PageEnb"=T34."Page Disabled & Grayed" ("Page Enabled State")) -> ()  [unwired: 1 in, 2 out]
          }
          frame False {
            n217 = property class="Page"(reference=w388, "PageEnb"=T34."Page Enabled" ("Page Enabled State")) -> ()  [unwired: 1 in, 2 out]
          }
        }
      }
      event "REF_EDIT_clear_status": Value Change {
        n218 = event-data() -> ()  [unwired: 1 in, 6 out]
        n219 = call "FGV_REF_EDITOR_status_display.vi"("options"=FGV_REF_EDITOR_status_display."clear", "error_in"=w391) -> ("error_out"=w390:errorcluster)  [unwired: 9 in]
      }
      event "REF_EDIT_delete": Value Change {
        n220 = event-data() -> ()  [unwired: 1 in, 6 out]
        n221 = local read "REF_EDIT_records"() -> (w393:i32)
        n222 = case shown="-1" w393 {
          tunnel: w396 -> [_ w408]
          tunnel: [w403 w407] -> w395
          tunnel: w394 -> [_ w406]
          frame -1 {
            n223 = call-poly "Get Localized Phrase Compact Interface.vi"("Key"="No record selected for DELETE" ("source")) -> ("Translated Phrase"=w399:string)
            n224 = Bundle By Name(cluster=errorcluster {"status"=FALSE, "code"=503, "source"=""} ("error out"), "source"=w399) -> (w398:errorcluster)
            n225 = call "FGV_REF_EDITOR_status_display.vi"("options"=FGV_REF_EDITOR_status_display."display", "error_in"=w398, "display_source"="DELETE") -> ("error_out"=w403:errorcluster)  [unwired: 8 in]
          }
          frame Default {
            n226 = Unbundle By Name(w406) -> ("queue_refnums.SQL_EDITOR_queue"=w409:refnum<queue>)
            n227 = Enqueue Element(queue=w409, element=T32 {"state"=enum."REF_delete_record", "variable"=variant}, error in (no error)=w408) -> (error out=w407:errorcluster)  [unwired: 1 in, 2 out]
          }
        }
      }
      event "REF_EDIT_discard": Value Change {
        n228 = event-data() -> ()  [unwired: 1 in, 6 out]
        n229 = local read "REF_EDIT_records"() -> (w412:i32)
        n230 = case shown="Default" w412 {
          selector: w412 -> [_ w419]
          tunnel: w411 -> [w414 w417]
          tunnel: [w414 w416] -> w410
          frame -1 {
          }
          frame Default {
            n231 = To Variant(anything=w419) -> (Variant=w418:variant)
            n232 = call "FGV_REF_EDITOR_records_display.vi"("options"=FGV_REF_EDITOR_records_display."discard_changes", "error_in"=w417, "input"=w418) -> ("error_out"=w416:errorcluster)  [unwired: 5 in, 3 out]
          }
        }
      }
      event "REF_EDIT_insert_update": Value Change {
        n233 = event-data() -> ()  [unwired: 1 in, 6 out]
        n234 = local read "REF_EDIT_records"() -> (w420:i32)
        n235 = case shown="Default" w420 {
          selector: w420 -> [_ w435]
          tunnel: w423 -> [_ w439]
          tunnel: [w430 w438] -> w422
          tunnel: w421 -> [_ w437]
          frame -1 {
            n236 = call-poly "Get Localized Phrase Compact Interface.vi"("Key"="No record selected for INSERT / UPDATE" ("source")) -> ("Translated Phrase"=w426:string)
            n237 = Bundle By Name(cluster=errorcluster {"status"=FALSE, "code"=503, "source"=""} ("error out"), "source"=w426) -> (w425:errorcluster)
            n238 = call "FGV_REF_EDITOR_status_display.vi"("options"=FGV_REF_EDITOR_status_display."display", "error_in"=w425, "display_source"="INSERT / UPDATE") -> ("error_out"=w430:errorcluster)  [unwired: 8 in]
          }
          frame Default {
            n239 = call "FGV_REF_EDITOR_records_display.vi"("options"=FGV_REF_EDITOR_records_display."get_all_info") -> ("all_info"=w433:T47)  [unwired: 7 in, 3 out]
            n240 = Unbundle By Name(w433) -> ("REF_record_states"=w436:T44[])
            n241 = Index Array(array=w436, index=w435) -> (element=w434:T44)
            n242 = case shown="\"Equal\"" w434 {
              tunnel: w439 -> [_ w446 w451]
              tunnel: [w441 w445 w450] -> w438
              tunnel: w437 -> [_ w444 w449]
              frame "Equal" {
                n243 = call "FGV_REF_EDITOR_status_display.vi"("options"=FGV_REF_EDITOR_status_display."display", "display_source"="INSERT / UPDATE") -> ("error_out"=w441:errorcluster)  [unwired: 9 in]
              }
              frame "Added", "Deleted" {
                n244 = Unbundle By Name(w444) -> ("queue_refnums.SQL_EDITOR_queue"=w447:refnum<queue>)
                n245 = Enqueue Element(queue=w447, element=T32 {"state"=enum."REF_insert_record", "variable"=variant}, error in (no error)=w446) -> (error out=w445:errorcluster)  [unwired: 1 in, 2 out]
              }
              frame "Edited" {
                n246 = Unbundle By Name(w449) -> ("queue_refnums.SQL_EDITOR_queue"=w452:refnum<queue>)
                n247 = Enqueue Element(queue=w452, element=T32 {"state"=enum."REF_update_record", "variable"=variant}, error in (no error)=w451) -> (error out=w450:errorcluster)  [unwired: 1 in, 2 out]
              }
            }
          }
        }
      }
      event "REF_EDIT_records": Double Click {
        # "Workaround for delay of editting multicolumn listbox (without this editting possible after two clicks with 1sec. break between them)"
        n248 = event-data() -> ("CtlRef"=w456:refnum<vi>, "Coords"=w455:T45)  [unwired: 1 in, 4 out]
        n249 = invoke class="MCListbox (strict)" method="Point To Row Column"(reference=w456, "Point"=w455) -> (reference out=w459:refnum<vi>, error out=w458:errorcluster, "CellPosition"=w457:T36)  [unwired: 5 in, 4 out]
        n250 = property class="MCListbox (strict)"(reference=w459, error in=w458, "EditPos"=w457) -> ()  [unwired: 2 out]
      }
      event "REF_EDIT_records": Edit Cell {
        n251 = event-data() -> ("Coords.Row"=w460:i32)  [unwired: 1 in]
        n252 = call "FGV_REF_EDITOR_records_display.vi"("options"=FGV_REF_EDITOR_records_display."get_all_info") -> ("all_info"=w462:T47)  [unwired: 7 in, 3 out]
        n253 = Unbundle By Name(w462) -> ("size.SQL_rows"=w463:i32)
        n254 = local write "REF_EDIT_records"(w460) -> ()
        n255 = Greater Or Equal?(x=w460, y=w463) -> (x >= y?=w464:bool)
        n256 = case shown="False" w464 {
          tunnel: w460 -> [w469 w472]
          frame False {
            n257 = To Variant(anything=w469) -> (Variant=w467:variant)
            n258 = call "FGV_REF_EDITOR_records_display.vi"("options"=FGV_REF_EDITOR_records_display."record_edited?", "input"=w467) -> ()  [unwired: 6 in, 4 out]
          }
          frame True {
            n259 = To Variant(anything=w472) -> (Variant=w470:variant)
            n260 = call "FGV_REF_EDITOR_records_display.vi"("options"=FGV_REF_EDITOR_records_display."record_added?", "input"=w470) -> ()  [unwired: 6 in, 4 out]
          }
        }
      }
      event "REF_EDIT_records": Edit Cell? {
        n261 = event-data() -> ("String"=w476:string, "Coords.Column"=w477:i32)  [unwired: 1 in]
        n262 = case shown="5" w477 {
          tunnel: w476 -> [w479 w481]
          tunnel: [w479 w484] -> w475
          frame Default {
          }
          frame 5 {
            # "VALUE"
            n263 = xnode "Match Regular Expression"("input string"=w481, "regular expression"="^(\\d+(?:[\\,]{1}\\d+)+)$") -> ("whole match"=w482:string)  [unwired: 4 in, 4 out]
            n264 = Equal?(x=w481, y=w482) -> (x = y?=w480:bool)
            n265 = case shown="True" w480 {
              tunnel: [w485 w487] -> w484
              tunnel: w481 -> [w485 w486]
              frame False {
              }
              frame True {
                n266 = Search and Replace String(replace all?=TRUE ("replace all? (F)"), input string=w486, search string=",", replace string="." ("replace string (\"\")")) -> (result string=w487:string)  [unwired: 4 in, 3 out]
              }
            }
          }
        }
        n267 = event-data("String"=w475, "Discard?"=FALSE) -> ()  [unwired: 1 in, 1 out]
      }
      event "REF_EDIT_records": Key Down? {
        n268 = event-data() -> ("CtlRef"=w607:refnum<vi>, "ScanCode"=w609:i16, "PlatMods.Shift"=w605:bool)  [unwired: 1 in, 1 out]
        n269 = case shown="80" w609 {
          tunnel: [_ TRUE w618 w629 w640 w651] -> w608
          tunnel: w607 -> [_ w616 w620 w631 w642 w653]
          tunnel: w605 -> [_ _ w619 w630 w641 w652]
          frame Default {
          }
          frame 15 {
            # "15 = Tab"
            n270 = call "FGV_REF_EDITOR_records_display.vi"("options"=FGV_REF_EDITOR_records_display."get_all_info") -> ("all_info"=w614:T47)  [unwired: 7 in, 3 out]
            n271 = Unbundle By Name(w614) -> ("editable_columns"=w612:i32[], "size.SQL_rows"=w611:i32)
            n272 = call "EDITORS_calculate_next_pos_for_keyboard_events.vi"("direction"=directions."RIGHT", "SQL_rows"=w611, "editable_columns"=w612, "reference"=w616) -> ()  [unwired: 8 in]
          }
          frame 75 {
            # "75 = Left Arrow"
            n273 = case shown="True" w619 {
              tunnel: w620 -> [_ w628]
              tunnel: [FALSE TRUE] -> w618
              frame False {
              }
              frame True {
                n274 = call "FGV_REF_EDITOR_records_display.vi"("options"=FGV_REF_EDITOR_records_display."get_all_info") -> ("all_info"=w625:T47)  [unwired: 7 in, 3 out]
                n275 = Unbundle By Name(w625) -> ("editable_columns"=w623:i32[], "size.SQL_rows"=w622:i32)
                n276 = call "EDITORS_calculate_next_pos_for_keyboard_events.vi"("direction"=directions."LEFT", "SQL_rows"=w622, "editable_columns"=w623, "reference"=w628) -> ()  [unwired: 8 in]
              }
            }
          }
          frame 77 {
            # "77 = Right Arrow"
            n277 = case shown="True" w630 {
              tunnel: w631 -> [_ w639]
              tunnel: [FALSE TRUE] -> w629
              frame False {
              }
              frame True {
                n278 = call "FGV_REF_EDITOR_records_display.vi"("options"=FGV_REF_EDITOR_records_display."get_all_info") -> ("all_info"=w636:T47)  [unwired: 7 in, 3 out]
                n279 = Unbundle By Name(w636) -> ("editable_columns"=w634:i32[], "size.SQL_rows"=w633:i32)
                n280 = call "EDITORS_calculate_next_pos_for_keyboard_events.vi"("direction"=directions."RIGHT", "SQL_rows"=w633, "editable_columns"=w634, "reference"=w639) -> ()  [unwired: 8 in]
              }
            }
          }
          frame 72 {
            # "72 = Up Arrow"
            n281 = case shown="True" w641 {
              tunnel: w642 -> [_ w650]
              tunnel: [FALSE TRUE] -> w640
              frame False {
              }
              frame True {
                n282 = call "FGV_REF_EDITOR_records_display.vi"("options"=FGV_REF_EDITOR_records_display."get_all_info") -> ("all_info"=w647:T47)  [unwired: 7 in, 3 out]
                n283 = Unbundle By Name(w647) -> ("editable_columns"=w645:i32[], "size.SQL_rows"=w644:i32)
                n284 = call "EDITORS_calculate_next_pos_for_keyboard_events.vi"("direction"=directions."UP", "SQL_rows"=w644, "editable_columns"=w645, "reference"=w650) -> ()  [unwired: 8 in]
              }
            }
          }
          frame 80 {
            # "80 = Down Arrow"
            n285 = case shown="True" w652 {
              tunnel: w653 -> [_ w661]
              tunnel: [FALSE TRUE] -> w651
              frame False {
              }
              frame True {
                n286 = call "FGV_REF_EDITOR_records_display.vi"("options"=FGV_REF_EDITOR_records_display."get_all_info") -> ("all_info"=w658:T47)  [unwired: 7 in, 3 out]
                n287 = Unbundle By Name(w658) -> ("editable_columns"=w656:i32[], "size.SQL_rows"=w655:i32)
                n288 = call "EDITORS_calculate_next_pos_for_keyboard_events.vi"("direction"=directions."DOWN", "SQL_rows"=w655, "editable_columns"=w656, "reference"=w661) -> ()  [unwired: 8 in]
              }
            }
          }
        }
        n289 = event-data("Discard?"=w608) -> ()  [unwired: 1 in, 1 out]
      }
      event "REF_EDIT_records": Mouse Down? {
        n290 = event-data() -> ("CtlRef"=w670:refnum<vi>, "Coords"=w669:T45)  [unwired: 1 in]
        n291 = invoke class="MCListbox (strict)" method="Point To Row Column"(reference=w670, "Point"=w669) -> ("InBounds"=w662:bool, "CellPosition"=w668:T36)  [unwired: 5 in, 5 out]
        n292 = local read "REF_EDIT_records"() -> (w663:i32)
        n293 = Bundle By Name(cluster=w664, "REF_EDIT_selected_row"=w663) -> (w665:T21)
        n294 = case shown="True" w662 {
          selector: w662 -> [w673 _]
          tunnel: w668 -> [_ w677]
          tunnel: [w672 w676] -> w667
          tunnel: [w673 w675] -> w666
          tunnel: w665 -> [w672 w674]
          frame False {
          }
          frame True {
            n295 = call "REF_EDITOR_records_click_discard.vi"("CellPosition"=w677, "event_structure_shift_register_in"=w674) -> ("Discard?"=w675:bool, "event_structure_shift_register_out"=w676:T21)  [unwired: 8 in]
          }
        }
        n296 = event-data("Discard?"=w666) -> ()  [unwired: 1 in, 1 out]
      }
      event "REF_EDIT_refresh": Value Change {
        n297 = event-data() -> ()  [unwired: 1 in, 6 out]
        n298 = Unbundle By Name(w683) -> ("queue_refnums.SQL_EDITOR_queue"=w681:refnum<queue>)
        n299 = Enqueue Element(queue=w681, element=T32 {"state"=enum."REF_read_stations", "variable"=variant}, error in (no error)=w679) -> (error out=w682:errorcluster)  [unwired: 1 in, 2 out]
      }
      event "REF_EDIT_station": Value Change {
        n300 = event-data() -> ("CtlRef"=w691:refnum<vi>)  [unwired: 1 in, 5 out]
        n301 = property class="Ring (strict)"(reference=w691) -> ("RingText.Text"=w690:string)  [unwired: 1 in, 2 out]
        n302 = To Variant(anything=w690) -> (Variant=w686:variant)
        n303 = call "FGV_REF_EDITOR_records_display.vi"("options"=FGV_REF_EDITOR_records_display."set_station_number", "error_in"=w688, "input"=w686) -> ("error_out"=w687:errorcluster)  [unwired: 5 in, 3 out]
        n304 = Unbundle By Name(w694) -> ("queue_refnums.SQL_EDITOR_queue"=w692:refnum<queue>)
        n305 = Enqueue Element(queue=w692, element=T32 {"state"=enum."REF_select_station_records", "variable"=variant}, error in (no error)=w687) -> (error out=w693:errorcluster)  [unwired: 1 in, 2 out]
      }
      event Value Change {
        n306 = event-data() -> ("NewVal"=w698:T8)  [unwired: 1 in, 5 out]
        n307 = Format Into String(w698) -> (resulting string=w697:string)  [unwired: 3 in, 1 out]
        n308 = To Variant(anything=w697) -> (Variant=w700:variant)
        n309 = call "FGV_REF_EDITOR_records_display.vi"("options"=FGV_REF_EDITOR_records_display."set_type_filter", "error_in"=w702, "input"=w700) -> ("error_out"=w701:errorcluster)  [unwired: 5 in, 3 out]
        n310 = Unbundle By Name(w705) -> ("queue_refnums.SQL_EDITOR_queue"=w696:refnum<queue>)
        n311 = Enqueue Element(queue=w696, element=T32 {"state"=enum."REF_select_station_records", "variable"=variant}, error in (no error)=w701) -> (error out=w704:errorcluster)  [unwired: 1 in, 2 out]
      }
      event "REPORT_AUDIT_end_btn": Value Change {
        n312 = event-data() -> ()  [unwired: 1 in, 6 out]
        n313 = local read "REPORT_AUDIT_end"() -> (w706:timestamp)
        n314 = call "custom_picktime.vi"("secin"=w706) -> ("ok"=w707:bool, "secout"=w708:timestamp)  [unwired: 9 in]
        n315 = case shown="True" w707 {
          tunnel: w708 -> [_ w711]
          frame False {
          }
          frame True {
            n316 = local write "REPORT_AUDIT_end"(w711) -> ()
          }
        }
      }
      event "REPORT_AUDIT_order_selection": Value Change {
        n317 = event-data() -> ()  [unwired: 1 in, 6 out]
        n318 = property on="REPORT_AUDIT_OP_filter" class="Ring (strict)"() -> ("RingText.Text"=w714:string)  [unwired: 2 in, 2 out]
        n319 = property on="REPORT_AUDIT_status_filter" class="Ring (strict)"() -> ("RingText.Text"=w713:string)  [unwired: 2 in, 2 out]
        n320 = local read "REPORT_AUDIT_order_selection"() -> (w715:enum32{"old_to_new", "new_to_old"})
        n321 = Bundle By Name(cluster=T35 {"order_selection"=enum."new_to_old", "OP_filter"="", "status_filter"="", "show_hidden?"=FALSE}, "order_selection"=w715, "OP_filter"=w714, "status_filter"=w713, "show_hidden?"=FALSE) -> (w717:T35)
        n322 = To Variant(anything=w717) -> (Variant=w718:variant)
        n323 = call "FGV_REPORTS_records_display.vi"("options"=FGV_REPORTS_records_display."AUDIT_filter", "error_in"=w721, "input"=w718) -> ("error_out"=w720:errorcluster)  [unwired: 7 in, 1 out]
      }
      event "REPORT_AUDIT_start_btn": Value Change {
        n324 = event-data() -> ()  [unwired: 1 in, 6 out]
        n325 = local read "REPORT_AUDIT_start"() -> (w723:timestamp)
        n326 = call "custom_picktime.vi"("secin"=w723) -> ("ok"=w724:bool, "secout"=w725:timestamp)  [unwired: 9 in]
        n327 = case shown="True" w724 {
          tunnel: w725 -> [_ w728]
          frame False {
          }
          frame True {
            n328 = local write "REPORT_AUDIT_start"(w728) -> ()
          }
        }
      }
      event "REPORT_AUDIT_toggle_all_results": Value Change {
        n329 = event-data() -> ()  [unwired: 1 in, 1 out]
        n330 = Unbundle By Name(w732) -> ("REPORT_AUDIT_toggle_all_results"=w734:bool)
        n331 = case shown="True" w734 {
          selector: w734 -> [w751 w768]
          tunnel: [w750 w767] -> w733
          tunnel: w730 -> [w746 w754]
          tunnel: [w739 w753] -> w729
          frame False {
            n332 = local read "REPORT_AUDIT_order_selection"() -> (w736:enum32{"old_to_new", "new_to_old"})
            n333 = property on="REPORT_AUDIT_OP_filter" class="Ring (strict)"() -> ("RingText.Text"=w744:string)  [unwired: 2 in, 2 out]
            n334 = property on="REPORT_AUDIT_status_filter" class="Ring (strict)"() -> ("RingText.Text"=w745:string)  [unwired: 2 in, 2 out]
            n335 = call "FGV_REPORTS_records_display.vi"("options"=FGV_REPORTS_records_display."AUDIT_show_all_results", "error_in"=w746) -> ("error_out"=w740:errorcluster)  [unwired: 8 in, 1 out]
            n336 = call-poly "Get Localized Phrase Compact Interface.vi"("Key"="HIDE ALL RESULTS" ("Boolean Text.Text")) -> ("Translated Phrase"=w748:string)
            n337 = Not(x=w751) -> (.not. x?=w750:bool)
            n338 = property on="REPORT_AUDIT_toggle_all_results" class="Bool"("BoolText.Text"=w748) -> ()  [unwired: 2 in, 2 out]
            n339 = Bundle By Name(cluster=T35 {"order_selection"=enum."new_to_old", "OP_filter"="", "status_filter"="", "show_hidden?"=FALSE}, "order_selection"=w736, "OP_filter"=w744, "status_filter"=w745, "show_hidden?"=TRUE) -> (w737:T35)
            n340 = To Variant(anything=w737) -> (Variant=w738:variant)
            n341 = property on="REPORT_records" class="MCListbox (strict)"("TopLeft"=T36 {"Row"=0, "Column"=0} ("Active Cell:Active Cell")) -> ()  [unwired: 2 in, 2 out]
            n342 = call "FGV_REPORTS_records_display.vi"("options"=FGV_REPORTS_records_display."AUDIT_filter", "error_in"=w740, "input"=w738) -> ("error_out"=w739:errorcluster)  [unwired: 7 in, 1 out]
          }
          frame True {
            n343 = local read "REPORT_AUDIT_order_selection"() -> (w752:enum32{"old_to_new", "new_to_old"})
            n344 = property on="REPORT_AUDIT_OP_filter" class="Ring (strict)"() -> ("RingText.Text"=w761:string)  [unwired: 2 in, 2 out]
            n345 = property on="REPORT_AUDIT_status_filter" class="Ring (strict)"() -> ("RingText.Text"=w762:string)  [unwired: 2 in, 2 out]
            n346 = call "FGV_REPORTS_records_display.vi"("options"=FGV_REPORTS_records_display."AUDIT_hide_all_results", "error_in"=w754) -> ("error_out"=w757:errorcluster)  [unwired: 8 in, 1 out]
            n347 = call-poly "Get Localized Phrase Compact Interface.vi"("Key"="SHOW ALL RESULTS" ("Boolean Text.Text")) -> ("Translated Phrase"=w766:string)
            n348 = Not(x=w768) -> (.not. x?=w767:bool)
            n349 = property on="REPORT_AUDIT_toggle_all_results" class="Bool"("BoolText.Text"=w766) -> ()  [unwired: 2 in, 2 out]
            n350 = Bundle By Name(cluster=T35 {"order_selection"=enum."new_to_old", "OP_filter"="", "status_filter"="", "show_hidden?"=FALSE}, "order_selection"=w752, "OP_filter"=w761, "status_filter"=w762, "show_hidden?"=TRUE) -> (w755:T35)
            n351 = To Variant(anything=w755) -> (Variant=w756:variant)
            n352 = call "FGV_REPORTS_records_display.vi"("options"=FGV_REPORTS_records_display."AUDIT_filter", "error_in"=w757, "input"=w756) -> ("error_out"=w753:errorcluster)  [unwired: 7 in, 1 out]
            n353 = property on="REPORT_records" class="MCListbox (strict)"("TopLeft"=T36 {"Row"=0, "Column"=0} ("Active Cell:Active Cell")) -> ()  [unwired: 2 in, 2 out]
          }
        }
        n354 = Bundle By Name(cluster=w732, "REPORT_AUDIT_toggle_all_results"=w733) -> (w731:T21)
      }
      event "REPORT_CBATCH_order_selection": Value Change {
        n355 = event-data() -> ()  [unwired: 1 in, 6 out]
        n356 = local read "REPORT_CBATCH_order_selection"() -> (w769:enum32{"old_to_new", "new_to_old"})
        n357 = To Variant(anything=w769) -> (Variant=w770:variant)
        n358 = call "FGV_REPORTS_records_display.vi"("options"=FGV_REPORTS_records_display."CBATCH_filter", "error_in"=w773, "input"=w770) -> ("error_out"=w772:errorcluster)  [unwired: 7 in, 1 out]
      }
      event "REPORT_CBATCH_scan_barcode": Value Change {
        n359 = event-data() -> ()  [unwired: 1 in, 6 out]
        n360 = call "USER_EDITOR_scan_barcode.vi"("error_in"=w779, "all_config_info"=w778) -> ("error_out"=w777:errorcluster, "Canceled?"=w775:bool, "barcode"=w776:string)  [unwired: 7 in]
        n361 = case shown="False" w775 {
          tunnel: [w788 w790] -> w780
          tunnel: w777 -> [w787 w790]
          tunnel: w778 -> [w786 _]
          tunnel: w776 -> [w782 _]
          frame False {
            n362 = Unbundle By Name(w786) -> ("queue_refnums.SQL_EDITOR_queue"=w789:refnum<queue>)
            n363 = To Variant(anything=w782) -> (Variant=w783:variant)
            n364 = Bundle By Name(cluster=T32 {"state"=enum."REPORT_GEAR_scan_barcode", "variable"=variant} ("element"), "variable"=w783) -> (w784:T32)
            n365 = Enqueue Element(queue=w789, element=w784, error in (no error)=w787) -> (error out=w788:errorcluster)  [unwired: 1 in, 2 out]
          }
          frame True {
          }
        }
      }
      event "REPORT_CFG_end_btn": Value Change {
        n366 = event-data() -> ()  [unwired: 1 in, 6 out]
        n367 = local read "REPORT_CFG_end"() -> (w791:timestamp)
        n368 = call "custom_picktime.vi"("secin"=w791) -> ("ok"=w792:bool, "secout"=w793:timestamp)  [unwired: 9 in]
        n369 = case shown="True" w792 {
          tunnel: w793 -> [_ w796]
          frame False {
          }
          frame True {
            n370 = local write "REPORT_CFG_end"(w796) -> ()
          }
        }
      }
      event "REPORT_CFG_order_selection": Value Change {
        n371 = event-data() -> ()  [unwired: 1 in, 6 out]
        n372 = property on="REPORT_CFG_op_filter" class="Ring (strict)"() -> ("RingText.Text"=w798:string)  [unwired: 2 in, 2 out]
        n373 = local read "REPORT_CFG_order_selection"() -> (w799:enum32{"old_to_new", "new_to_old"})
        n374 = Bundle By Name(cluster=T37 {"order_selection"=enum."new_to_old", "OP"=""} ("REPORT_DATES_filters"), "order_selection"=w799, "OP"=w798) -> (w800:T37)
        n375 = To Variant(anything=w800) -> (Variant=w801:variant)
        n376 = call "FGV_REPORTS_records_display.vi"("options"=FGV_REPORTS_records_display."CFG_filter", "error_in"=w804, "input"=w801) -> ("error_out"=w803:errorcluster)  [unwired: 7 in, 1 out]
      }
      event "REPORT_CFG_start_btn": Value Change {
        n377 = event-data() -> ()  [unwired: 1 in, 6 out]
        n378 = local read "REPORT_CFG_start"() -> (w806:timestamp)
        n379 = call "custom_picktime.vi"("secin"=w806) -> ("ok"=w807:bool, "secout"=w808:timestamp)  [unwired: 9 in]
        n380 = case shown="True" w807 {
          tunnel: w808 -> [_ w811]
          frame False {
          }
          frame True {
            n381 = local write "REPORT_CFG_start"(w811) -> ()
          }
        }
      }
      event "REPORT_clear": Value Change {
        n382 = event-data() -> ()  [unwired: 1 in, 1 out]
        n383 = local read "REPORT_filters"() -> (w816:T2)
        n384 = case shown="\"OK/NOK Count\"" w816 {
          tunnel: w815 -> [w819 w822 w825 w828 w831 w834 w837 w840 w843 w846 w849 w850]
          tunnel: [w818 w821 w824 w827 w830 w833 w836 w839 w842 w845 w848 w850] -> w814
          tunnel: w813 -> [_ _ _ _ _ _ _ _ _ _ _ _]
          frame "Gear" {
            n385 = call "FGV_REPORTS_records_display.vi"("options"=FGV_REPORTS_records_display."GEAR_clear", "error_in"=w819) -> ("error_out"=w818:errorcluster)  [unwired: 8 in, 1 out]
          }
          frame "Dates" {
            n386 = call "FGV_REPORTS_records_display.vi"("options"=FGV_REPORTS_records_display."DATES_clear", "error_in"=w822) -> ("error_out"=w821:errorcluster)  [unwired: 8 in, 1 out]
          }
          frame "Production Batch" {
            n387 = call "FGV_REPORTS_records_display.vi"("options"=FGV_REPORTS_records_display."PBATCH_clear", "error_in"=w825) -> ("error_out"=w824:errorcluster)  [unwired: 8 in, 1 out]
          }
          frame "Operation" {
            n388 = call "FGV_REPORTS_records_display.vi"("options"=FGV_REPORTS_records_display."OPRTN_clear", "error_in"=w828) -> ("error_out"=w827:errorcluster)  [unwired: 8 in, 1 out]
          }
          frame "Config History" {
            n389 = call "FGV_REPORTS_records_display.vi"("options"=FGV_REPORTS_records_display."CFG_clear", "error_in"=w831) -> ("error_out"=w830:errorcluster)  [unwired: 8 in, 1 out]
          }
          frame "Audits" {
            n390 = call "FGV_REPORTS_records_display.vi"("options"=FGV_REPORTS_records_display."AUDIT_clear", "error_in"=w834) -> ("error_out"=w833:errorcluster)  [unwired: 8 in, 1 out]
          }
          frame "OK/NOK Count" {
            n391 = call "FGV_REPORTS_records_display.vi"("options"=FGV_REPORTS_records_display."OKNOK_clear", "error_in"=w837) -> ("error_out"=w836:errorcluster)  [unwired: 8 in, 1 out]
          }
          frame "Reworks" {
            n392 = call "FGV_REPORTS_records_display.vi"("options"=FGV_REPORTS_records_display."REWORKS_clear", "error_in"=w840) -> ("error_out"=w839:errorcluster)  [unwired: 8 in, 1 out]
          }
          frame "Pace" {
            n393 = call "FGV_REPORTS_records_display.vi"("options"=FGV_REPORTS_records_display."PACE_clear", "error_in"=w843) -> ("error_out"=w842:errorcluster)  [unwired: 8 in, 1 out]
          }
          frame "Customer Batch" {
            n394 = call "FGV_REPORTS_records_display.vi"("options"=FGV_REPORTS_records_display."CBATCH_clear", "error_in"=w846) -> ("error_out"=w845:errorcluster)  [unwired: 8 in, 1 out]
          }
          frame "Gear Components" {
            n395 = call "FGV_REPORTS_records_display.vi"("options"=FGV_REPORTS_records_display."CMPNT_clear", "error_in"=w849) -> ("error_out"=w848:errorcluster)  [unwired: 8 in, 1 out]
          }
          frame Default {
          }
        }
      }
      event "REPORT_CMPNT_scan_barcode": Value Change {
        n396 = event-data() -> ()  [unwired: 1 in, 6 out]
        n397 = call "USER_EDITOR_scan_barcode.vi"("error_in"=w855, "all_config_info"=w854) -> ("error_out"=w853:errorcluster, "Canceled?"=w851:bool, "barcode"=w852:string)  [unwired: 7 in]
        n398 = case shown="False" w851 {
          tunnel: [w864 w866] -> w856
          tunnel: w853 -> [w863 w866]
          tunnel: w854 -> [w862 _]
          tunnel: w852 -> [w858 _]
          frame False {
            n399 = Unbundle By Name(w862) -> ("queue_refnums.SQL_EDITOR_queue"=w865:refnum<queue>)
            n400 = To Variant(anything=w858) -> (Variant=w859:variant)
            n401 = Bundle By Name(cluster=T32 {"state"=enum."REPORT_CMPNT_scan_barcode", "variable"=variant} ("element"), "variable"=w859) -> (w860:T32)
            n402 = Enqueue Element(queue=w865, element=w860, error in (no error)=w863) -> (error out=w864:errorcluster)  [unwired: 1 in, 2 out]
          }
          frame True {
          }
        }
      }
      event "REPORT_DATES_end_btn": Value Change {
        n403 = event-data() -> ()  [unwired: 1 in, 6 out]
        n404 = local read "REPORT_DATES_end"() -> (w867:timestamp)
        n405 = call "custom_picktime.vi"("secin"=w867) -> ("ok"=w868:bool, "secout"=w869:timestamp)  [unwired: 9 in]
        n406 = case shown="True" w868 {
          tunnel: w869 -> [_ w872]
          frame False {
          }
          frame True {
            n407 = local write "REPORT_DATES_end"(w872) -> ()
          }
        }
      }
      event "REPORT_DATES_order_selection": Value Change {
        n408 = event-data() -> ()  [unwired: 1 in, 6 out]
        n409 = property on="REPORT_DATES_last_op" class="Ring (strict)"() -> ("RingText.Text"=w874:string)  [unwired: 2 in, 2 out]
        n410 = property on="REPORT_DATES_last_status" class="Ring (strict)"() -> ("RingText.Text"=w873:string)  [unwired: 2 in, 2 out]
        n411 = local read "REPORT_DATES_order_selection"() -> (w875:enum32{"old_to_new", "new_to_old"})
        n412 = Bundle By Name(cluster=T38 {"order_selection"=enum."new_to_old", "last_OP"="", "last_status"=""}, "order_selection"=w875, "last_OP"=w874, "last_status"=w873) -> (w877:T38)
        n413 = To Variant(anything=w877) -> (Variant=w878:variant)
        n414 = call "FGV_REPORTS_records_display.vi"("options"=FGV_REPORTS_records_display."DATES_filter", "error_in"=w881, "input"=w878) -> ("error_out"=w880:errorcluster)  [unwired: 7 in, 1 out]
      }
      event "REPORT_DATES_start_btn": Value Change {
        n415 = event-data() -> ()  [unwired: 1 in, 6 out]
        n416 = local read "REPORT_DATES_start"() -> (w883:timestamp)
        n417 = call "custom_picktime.vi"("secin"=w883) -> ("ok"=w884:bool, "secout"=w885:timestamp)  [unwired: 9 in]
        n418 = case shown="True" w884 {
          tunnel: w885 -> [_ w888]
          frame False {
          }
          frame True {
            n419 = local write "REPORT_DATES_start"(w888) -> ()
          }
        }
      }
      event Value Change {
        n420 = event-data() -> ("NewVal"=w891:T2)  [unwired: 1 in]
        n421 = case shown="\"OK/NOK Count\"" w891 {
          tunnel: w890 -> [w895 w898 w901 w904 w907 w910 w913 w916 w919 w922 w925 w926]
          tunnel: [w894 w897 w900 w903 w906 w909 w912 w915 w918 w921 w924 w926] -> w889
          frame "Gear" {
            n422 = call "FGV_REPORTS_records_display.vi"("options"=FGV_REPORTS_records_display."GEAR_restore", "error_in"=w895) -> ("error_out"=w894:errorcluster)  [unwired: 8 in, 1 out]
          }
          frame "Dates" {
            n423 = call "FGV_REPORTS_records_display.vi"("options"=FGV_REPORTS_records_display."DATES_restore", "error_in"=w898) -> ("error_out"=w897:errorcluster)  [unwired: 8 in, 1 out]
          }
          frame "Production Batch" {
            n424 = call "FGV_REPORTS_records_display.vi"("options"=FGV_REPORTS_records_display."PBATCH_restore", "error_in"=w901) -> ("error_out"=w900:errorcluster)  [unwired: 8 in, 1 out]
          }
          frame "Operation" {
            n425 = call "FGV_REPORTS_records_display.vi"("options"=FGV_REPORTS_records_display."OPRTN_restore", "error_in"=w904) -> ("error_out"=w903:errorcluster)  [unwired: 8 in, 1 out]
          }
          frame "Config History" {
            n426 = call "FGV_REPORTS_records_display.vi"("options"=FGV_REPORTS_records_display."CFG_restore", "error_in"=w907) -> ("error_out"=w906:errorcluster)  [unwired: 8 in, 1 out]
          }
          frame "Audits" {
            n427 = call "FGV_REPORTS_records_display.vi"("options"=FGV_REPORTS_records_display."AUDIT_restore", "error_in"=w910) -> ("error_out"=w909:errorcluster)  [unwired: 8 in, 1 out]
          }
          frame "OK/NOK Count" {
            n428 = call "FGV_REPORTS_records_display.vi"("options"=FGV_REPORTS_records_display."OKNOK_restore", "error_in"=w913) -> ("error_out"=w912:errorcluster)  [unwired: 8 in, 1 out]
          }
          frame "Reworks" {
            n429 = call "FGV_REPORTS_records_display.vi"("options"=FGV_REPORTS_records_display."REWORKS_restore", "error_in"=w916) -> ("error_out"=w915:errorcluster)  [unwired: 8 in, 1 out]
          }
          frame "Pace" {
            n430 = call "FGV_REPORTS_records_display.vi"("options"=FGV_REPORTS_records_display."PACE_restore", "error_in"=w919) -> ("error_out"=w918:errorcluster)  [unwired: 8 in, 1 out]
          }
          frame "Customer Batch" {
            n431 = call "FGV_REPORTS_records_display.vi"("options"=FGV_REPORTS_records_display."CBATCH_restore", "error_in"=w922) -> ("error_out"=w921:errorcluster)  [unwired: 8 in, 1 out]
          }
          frame "Gear Components" {
            n432 = call "FGV_REPORTS_records_display.vi"("options"=FGV_REPORTS_records_display."CMPNT_restore", "error_in"=w925) -> ("error_out"=w924:errorcluster)  [unwired: 8 in, 1 out]
          }
          frame Default {
          }
        }
      }
      event "REPORT_GEAR_scan_barcode": Value Change {
        n433 = event-data() -> ()  [unwired: 1 in, 6 out]
        n434 = call "USER_EDITOR_scan_barcode.vi"("error_in"=w931, "all_config_info"=w930) -> ("error_out"=w929:errorcluster, "Canceled?"=w927:bool, "barcode"=w928:string)  [unwired: 7 in]
        n435 = case shown="False" w927 {
          tunnel: [w940 w942] -> w932
          tunnel: w929 -> [w939 w942]
          tunnel: w930 -> [w938 _]
          tunnel: w928 -> [w934 _]
          frame False {
            n436 = Unbundle By Name(w938) -> ("queue_refnums.SQL_EDITOR_queue"=w941:refnum<queue>)
            n437 = To Variant(anything=w934) -> (Variant=w935:variant)
            n438 = Bundle By Name(cluster=T32 {"state"=enum."REPORT_GEAR_scan_barcode", "variable"=variant} ("element"), "variable"=w935) -> (w936:T32)
            n439 = Enqueue Element(queue=w941, element=w936, error in (no error)=w939) -> (error out=w940:errorcluster)  [unwired: 1 in, 2 out]
          }
          frame True {
          }
        }
      }
      event Value Change {
        n440 = event-data() -> ()  [unwired: 1 in, 6 out]
        n441 = property on="REPORT_GEAR_station" class="Ring (strict)"() -> ("RingText.Text"=w943:string)  [unwired: 2 in, 2 out]
        n442 = To Variant(anything=w943) -> (Variant=w944:variant)
        n443 = call "FGV_REPORTS_records_display.vi"("options"=FGV_REPORTS_records_display."GEAR_filter", "error_in"=w945, "input"=w944) -> ("error_out"=w946:errorcluster)  [unwired: 7 in, 1 out]
      }
      event "REPORT_GEAR_toggle_all_results": Value Change {
        n444 = event-data() -> ()  [unwired: 1 in, 1 out]
        n445 = Unbundle By Name(w951) -> ("REPORT_GEAR_toggle_all_results"=w952:bool)
        n446 = case shown="False" w952 {
          selector: w952 -> [w960 w971]
          tunnel: [w963 w975] -> w954
          tunnel: w953 -> [w966 w978]
          tunnel: [w959 w970] -> w949
          frame True {
            n447 = call "FGV_REPORTS_records_display.vi"("options"=FGV_REPORTS_records_display."GEAR_hide_all_results", "error_in"=w966) -> ("error_out"=w964:errorcluster)  [unwired: 8 in, 1 out]
            n448 = call-poly "Get Localized Phrase Compact Interface.vi"("Key"="SHOW ALL RESULTS" ("Boolean Text.Text")) -> ("Translated Phrase"=w955:string)
            n449 = property on="REPORT_GEAR_toggle_all_results" class="Bool"("BoolText.Text"=w955) -> ()  [unwired: 2 in, 2 out]
            n450 = property on="REPORT_GEAR_station" class="Ring (strict)"() -> ("RingText.Text"=w956:string)  [unwired: 2 in, 2 out]
            n451 = To Variant(anything=w956) -> (Variant=w961:variant)
            n452 = property on="REPORT_records" class="MCListbox (strict)"("TopLeft"=T36 {"Row"=0, "Column"=0} ("Active Cell:Active Cell")) -> ()  [unwired: 2 in, 2 out]
            n453 = call "FGV_REPORTS_records_display.vi"("options"=FGV_REPORTS_records_display."GEAR_filter", "error_in"=w964, "input"=w961) -> ("error_out"=w963:errorcluster)  [unwired: 7 in, 1 out]
            n454 = Not(x=w960) -> (.not. x?=w959:bool)
          }
          frame False {
            n455 = call "FGV_REPORTS_records_display.vi"("options"=FGV_REPORTS_records_display."GEAR_show_all_results", "error_in"=w978) -> ("error_out"=w976:errorcluster)  [unwired: 8 in, 1 out]
            n456 = call-poly "Get Localized Phrase Compact Interface.vi"("Key"="HIDE ALL RESULTS" ("Boolean Text.Text")) -> ("Translated Phrase"=w967:string)
            n457 = property on="REPORT_GEAR_toggle_all_results" class="Bool"("BoolText.Text"=w967) -> ()  [unwired: 2 in, 2 out]
            n458 = local read "REPORT_GEAR_station"() -> (w973:T3)
            n459 = To Variant(anything=w973) -> (Variant=w972:variant)
            n460 = property on="REPORT_records" class="MCListbox (strict)"("TopLeft"=T36 {"Row"=0, "Column"=0} ("Active Cell:Active Cell")) -> ()  [unwired: 2 in, 2 out]
            n461 = call "FGV_REPORTS_records_display.vi"("options"=FGV_REPORTS_records_display."GEAR_display", "error_in"=w976, "input"=w972) -> ("error_out"=w975:errorcluster)  [unwired: 7 in, 1 out]
            n462 = Not(x=w971) -> (.not. x?=w970:bool)
          }
        }
        n463 = Bundle By Name(cluster=w951, "REPORT_GEAR_toggle_all_results"=w949) -> (w950:T21)
      }
      event "REPORT_get": Value Change {
        n464 = event-data() -> ()  [unwired: 1 in, 1 out]
        n465 = local read "REPORT_filters"() -> (w984:T2)
        n466 = case shown="\"Audits\"" w984 {
          tunnel: w983 -> [w992 w998 w1004 w1010 w1016 w1026 w1032 w1038 w1044 w1050 w1056 w1060]
          tunnel: [w991 w997 w1003 w1009 w1015 w1025 w1031 w1037 w1043 w1049 w1055 w1060] -> w982
          tunnel: w981 -> [w990 w996 w1002 w1008 w1014 w1024 w1030 w1036 w1042 w1048 w1054 _]
          tunnel: w980 -> [w989 w995 w1001 w1007 w1013 w1020 w1029 w1035 w1041 w1047 w1053 w1059]
          tunnel: [w987 w995 w1001 w1007 w1013 w1019 w1029 w1035 w1041 w1047 w1053 w1059] -> w979
          frame "Gear" {
            n467 = Unbundle By Name(w990) -> ("queue_refnums.SQL_EDITOR_queue"=w994:refnum<queue>)
            n468 = Enqueue Element(queue=w994, element=T32 {"state"=enum."REPORT_GEAR_get", "variable"=variant}, error in (no error)=w992) -> (error out=w991:errorcluster)  [unwired: 1 in, 2 out]
            n469 = Bundle By Name(cluster=w989, "REPORT_GEAR_toggle_all_results"=FALSE) -> (w987:T21)
            n470 = call-poly "Get Localized Phrase Compact Interface.vi"("Key"="SHOW ALL RESULTS" ("Boolean Text.Text")) -> ("Translated Phrase"=w985:string)
            n471 = property on="REPORT_GEAR_toggle_all_results" class="Bool"("BoolText.Text"=w985) -> ()  [unwired: 2 in, 2 out]
          }
          frame "Dates" {
            n472 = Unbundle By Name(w996) -> ("queue_refnums.SQL_EDITOR_queue"=w1000:refnum<queue>)
            n473 = Enqueue Element(queue=w1000, element=T32 {"state"=enum."REPORT_DATES_get", "variable"=variant}, error in (no error)=w998) -> (error out=w997:errorcluster)  [unwired: 1 in, 2 out]
          }
          frame "Production Batch" {
            n474 = Unbundle By Name(w1002) -> ("queue_refnums.SQL_EDITOR_queue"=w1006:refnum<queue>)
            n475 = Enqueue Element(queue=w1006, element=T32 {"state"=enum."REPORT_PBATCH_get", "variable"=variant}, error in (no error)=w1004) -> (error out=w1003:errorcluster)  [unwired: 1 in, 2 out]
          }
          frame "Operation" {
            n476 = Unbundle By Name(w1008) -> ("queue_refnums.SQL_EDITOR_queue"=w1012:refnum<queue>)
            n477 = Enqueue Element(queue=w1012, element=T32 {"state"=enum."REPORT_OPRTN_get", "variable"=variant}, error in (no error)=w1010) -> (error out=w1009:errorcluster)  [unwired: 1 in, 2 out]
          }
          frame "Config History" {
            n478 = Unbundle By Name(w1014) -> ("queue_refnums.SQL_EDITOR_queue"=w1018:refnum<queue>)
            n479 = Enqueue Element(queue=w1018, element=T32 {"state"=enum."REPORT_CFG_get", "variable"=variant}, error in (no error)=w1016) -> (error out=w1015:errorcluster)  [unwired: 1 in, 2 out]
          }
          frame "Audits" {
            n480 = Unbundle By Name(w1024) -> ("queue_refnums.SQL_EDITOR_queue"=w1028:refnum<queue>)
            n481 = Enqueue Element(queue=w1028, element=T32 {"state"=enum."REPORT_AUDIT_get", "variable"=variant}, error in (no error)=w1026) -> (error out=w1025:errorcluster)  [unwired: 1 in, 2 out]
            n482 = Bundle By Name(cluster=w1020, "REPORT_AUDIT_toggle_all_results"=FALSE ("REPORT_GEAR_toggle_all_results")) -> (w1019:T21)
            n483 = call-poly "Get Localized Phrase Compact Interface.vi"("Key"="SHOW ALL RESULTS" ("Boolean Text.Text")) -> ("Translated Phrase"=w1021:string)
            n484 = property on="REPORT_AUDIT_toggle_all_results" class="Bool"("BoolText.Text"=w1021) -> ()  [unwired: 2 in, 2 out]
          }
          frame "OK/NOK Count" {
            n485 = Unbundle By Name(w1030) -> ("queue_refnums.SQL_EDITOR_queue"=w1034:refnum<queue>)
            n486 = Enqueue Element(queue=w1034, element=T32 {"state"=enum."REPORT_OKNOK_get", "variable"=variant}, error in (no error)=w1032) -> (error out=w1031:errorcluster)  [unwired: 1 in, 2 out]
          }
          frame "Reworks" {
            n487 = Unbundle By Name(w1036) -> ("queue_refnums.SQL_EDITOR_queue"=w1040:refnum<queue>)
            n488 = Enqueue Element(queue=w1040, element=T32 {"state"=enum."REPORT_REWORKS_get", "variable"=variant}, error in (no error)=w1038) -> (error out=w1037:errorcluster)  [unwired: 1 in, 2 out]
          }
          frame "Pace" {
            n489 = Unbundle By Name(w1042) -> ("queue_refnums.SQL_EDITOR_queue"=w1046:refnum<queue>)
            n490 = Enqueue Element(queue=w1046, element=T32 {"state"=enum."REPORT_PACE_get", "variable"=variant}, error in (no error)=w1044) -> (error out=w1043:errorcluster)  [unwired: 1 in, 2 out]
          }
          frame "Customer Batch" {
            n491 = Unbundle By Name(w1048) -> ("queue_refnums.SQL_EDITOR_queue"=w1052:refnum<queue>)
            n492 = Enqueue Element(queue=w1052, element=T32 {"state"=enum."REPORT_CBATCH_get", "variable"=variant}, error in (no error)=w1050) -> (error out=w1049:errorcluster)  [unwired: 1 in, 2 out]
          }
          frame "Gear Components" {
            n493 = Unbundle By Name(w1054) -> ("queue_refnums.SQL_EDITOR_queue"=w1058:refnum<queue>)
            n494 = Enqueue Element(queue=w1058, element=T32 {"state"=enum."REPORT_CMPNT_get", "variable"=variant}, error in (no error)=w1056) -> (error out=w1055:errorcluster)  [unwired: 1 in, 2 out]
          }
          frame Default {
          }
        }
      }
      event "REPORT_OKNOK_end_btn": Value Change {
        n495 = event-data() -> ()  [unwired: 1 in, 6 out]
        n496 = local read "REPORT_OKNOK_end"() -> (w1061:timestamp)
        n497 = call "custom_picktime.vi"("secin"=w1061) -> ("ok"=w1062:bool, "secout"=w1063:timestamp)  [unwired: 9 in]
        n498 = case shown="True" w1062 {
          tunnel: w1063 -> [_ w1066]
          frame False {
          }
          frame True {
            n499 = local write "REPORT_OKNOK_end"(w1066) -> ()
          }
        }
      }
      event "REPORT_OKNOK_start_btn": Value Change {
        n500 = event-data() -> ()  [unwired: 1 in, 6 out]
        n501 = local read "REPORT_OKNOK_start"() -> (w1067:timestamp)
        n502 = call "custom_picktime.vi"("secin"=w1067) -> ("ok"=w1068:bool, "secout"=w1069:timestamp)  [unwired: 9 in]
        n503 = case shown="True" w1068 {
          tunnel: w1069 -> [_ w1072]
          frame False {
          }
          frame True {
            n504 = local write "REPORT_OKNOK_start"(w1072) -> ()
          }
        }
      }
      event "REPORT_OPRTN_end_btn": Value Change {
        n505 = event-data() -> ()  [unwired: 1 in, 6 out]
        n506 = local read "REPORT_OPRTN_end"() -> (w1073:timestamp)
        n507 = call "custom_picktime.vi"("secin"=w1073) -> ("ok"=w1074:bool, "secout"=w1075:timestamp)  [unwired: 9 in]
        n508 = case shown="True" w1074 {
          tunnel: w1075 -> [_ w1078]
          frame False {
          }
          frame True {
            n509 = local write "REPORT_OPRTN_end"(w1078) -> ()
          }
        }
      }
      event "REPORT_OPRTN_filter_columns": Value Change {
        n510 = event-data() -> ()  [unwired: 1 in, 6 out]
        n511 = call "REPORT_OPRTN_filter_columns.vi"("error_in"=w1082) -> ("error_out"=w1081:errorcluster, "Canceled?"=w1079:bool)  [unwired: 9 in]
        n512 = case shown="False" w1079 {
          tunnel: w1081 -> [w1091 w1092]
          tunnel: [w1090 w1092] -> w1080
          frame False {
            n513 = local read "REPORT_OPRTN_order_selection"() -> (w1088:enum32{"old_to_new", "new_to_old"})
            n514 = property on="REPORT_OPRTN_last_status" class="Ring (strict)"() -> ("RingText.Text"=w1087:string)  [unwired: 2 in, 2 out]
            n515 = Bundle By Name(cluster=T39 {"order_selection"=enum."new_to_old", "last_status"=""} ("REPORT_DATES_filters"), "order_selection"=w1088, "last_status"=w1087) -> (w1084:T39)
            n516 = To Variant(anything=w1084) -> (Variant=w1085:variant)
            n517 = call "FGV_REPORTS_records_display.vi"("options"=FGV_REPORTS_records_display."OPRTN_filter_no_page_reset", "error_in"=w1091, "input"=w1085) -> ("error_out"=w1090:errorcluster)  [unwired: 7 in, 1 out]
          }
          frame True {
          }
        }
      }
      event "REPORT_OPRTN_order_selection": Value Change {
        n518 = event-data() -> ()  [unwired: 1 in, 6 out]
        n519 = property on="REPORT_OPRTN_last_status" class="Ring (strict)"() -> ("RingText.Text"=w1094:string)  [unwired: 2 in, 2 out]
        n520 = local read "REPORT_OPRTN_order_selection"() -> (w1095:enum32{"old_to_new", "new_to_old"})
        n521 = Bundle By Name(cluster=T39 {"order_selection"=enum."new_to_old", "last_status"=""} ("REPORT_DATES_filters"), "order_selection"=w1095, "last_status"=w1094) -> (w1096:T39)
        n522 = To Variant(anything=w1096) -> (Variant=w1097:variant)
        n523 = call "FGV_REPORTS_records_display.vi"("options"=FGV_REPORTS_records_display."OPRTN_filter", "error_in"=w1100, "input"=w1097) -> ("error_out"=w1099:errorcluster)  [unwired: 7 in, 1 out]
      }
      event "REPORT_OPRTN_start_btn": Value Change {
        n524 = event-data() -> ()  [unwired: 1 in, 6 out]
        n525 = local read "REPORT_OPRTN_start"() -> (w1102:timestamp)
        n526 = call "custom_picktime.vi"("secin"=w1102) -> ("ok"=w1103:bool, "secout"=w1104:timestamp)  [unwired: 9 in]
        n527 = case shown="True" w1103 {
          tunnel: w1104 -> [_ w1107]
          frame False {
          }
          frame True {
            n528 = local write "REPORT_OPRTN_start"(w1107) -> ()
          }
        }
      }
      event "REPORT_OPRTN_unfilter_columns": Value Change {
        n529 = event-data() -> ()  [unwired: 1 in, 6 out]
        n530 = To Variant(anything=i32[] [] ("x+y")) -> (Variant=w1109:variant)
        n531 = call "FGV_REPORTS_records_display.vi"("options"=FGV_REPORTS_records_display."OPRTN_set_hidden_columns", "error_in"=w1112, "input"=w1109) -> ("error_out"=w1111:errorcluster)  [unwired: 7 in, 1 out]
        n532 = local read "REPORT_OPRTN_order_selection"() -> (w1117:enum32{"old_to_new", "new_to_old"})
        n533 = property on="REPORT_OPRTN_last_status" class="Ring (strict)"() -> ("RingText.Text"=w1116:string)  [unwired: 2 in, 2 out]
        n534 = Bundle By Name(cluster=T39 {"order_selection"=enum."new_to_old", "last_status"=""} ("REPORT_DATES_filters"), "order_selection"=w1117, "last_status"=w1116) -> (w1113:T39)
        n535 = To Variant(anything=w1113) -> (Variant=w1114:variant)
        n536 = call "FGV_REPORTS_records_display.vi"("options"=FGV_REPORTS_records_display."OPRTN_filter_no_page_reset", "error_in"=w1111, "input"=w1114) -> ("error_out"=w1119:errorcluster)  [unwired: 7 in, 1 out]
      }
      event "REPORT_PACE_end_btn": Value Change {
        n537 = event-data() -> ()  [unwired: 1 in, 6 out]
        n538 = local read "REPORT_PACE_end"() -> (w1121:timestamp)
        n539 = call "custom_picktime.vi"("secin"=w1121) -> ("ok"=w1122:bool, "secout"=w1123:timestamp)  [unwired: 9 in]
        n540 = case shown="True" w1122 {
          tunnel: w1123 -> [_ w1126]
          frame False {
          }
          frame True {
            n541 = local write "REPORT_PACE_end"(w1126) -> ()
          }
        }
      }
      event "REPORT_PACE_start_btn": Value Change {
        n542 = event-data() -> ()  [unwired: 1 in, 6 out]
        n543 = local read "REPORT_PACE_start"() -> (w1127:timestamp)
        n544 = call "custom_picktime.vi"("secin"=w1127) -> ("ok"=w1128:bool, "secout"=w1129:timestamp)  [unwired: 9 in]
        n545 = case shown="True" w1128 {
          tunnel: w1129 -> [_ w1132]
          frame False {
          }
          frame True {
            n546 = local write "REPORT_PACE_start"(w1132) -> ()
          }
        }
      }
      event "REPORT_page_first": Value Change {
        n547 = event-data() -> ()  [unwired: 1 in, 6 out]
        n548 = local read "REPORT_filters"() -> (w1135:T2)
        n549 = case shown="\"Gear Components\"" w1135 {
          tunnel: w1134 -> [w1137 w1139 w1142 w1145 w1148 w1151 w1154 w1157 w1160 w1162]
          tunnel: [w1137 w1138 w1141 w1144 w1147 w1150 w1153 w1156 w1159 w1162] -> w1133
          frame "Gear" {
          }
          frame "Dates" {
            n550 = call "FGV_REPORTS_records_display.vi"("options"=FGV_REPORTS_records_display."DATES_first_page", "error_in"=w1139) -> ("error_out"=w1138:errorcluster)  [unwired: 8 in, 1 out]
          }
          frame "Production Batch" {
            n551 = call "FGV_REPORTS_records_display.vi"("options"=FGV_REPORTS_records_display."PBATCH_first_page", "error_in"=w1142) -> ("error_out"=w1141:errorcluster)  [unwired: 8 in, 1 out]
          }
          frame "Operation" {
            n552 = call "FGV_REPORTS_records_display.vi"("options"=FGV_REPORTS_records_display."OPRTN_first_page", "error_in"=w1145) -> ("error_out"=w1144:errorcluster)  [unwired: 8 in, 1 out]
          }
          frame "Config History" {
            n553 = call "FGV_REPORTS_records_display.vi"("options"=FGV_REPORTS_records_display."CFG_first_page", "error_in"=w1148) -> ("error_out"=w1147:errorcluster)  [unwired: 8 in, 1 out]
          }
          frame "Audits" {
            n554 = call "FGV_REPORTS_records_display.vi"("options"=FGV_REPORTS_records_display."AUDIT_first_page", "error_in"=w1151) -> ("error_out"=w1150:errorcluster)  [unwired: 8 in, 1 out]
          }
          frame "Reworks" {
            n555 = call "FGV_REPORTS_records_display.vi"("options"=FGV_REPORTS_records_display."REWORKS_first_page", "error_in"=w1154) -> ("error_out"=w1153:errorcluster)  [unwired: 8 in, 1 out]
          }
          frame "Customer Batch" {
            n556 = call "FGV_REPORTS_records_display.vi"("options"=FGV_REPORTS_records_display."CBATCH_first_page", "error_in"=w1157) -> ("error_out"=w1156:errorcluster)  [unwired: 8 in, 1 out]
          }
          frame "Gear Components" {
            n557 = call "FGV_REPORTS_records_display.vi"("options"=FGV_REPORTS_records_display."CMPNT_first_page", "error_in"=w1160) -> ("error_out"=w1159:errorcluster)  [unwired: 8 in, 1 out]
          }
          frame Default {
          }
        }
      }
      event "REPORT_page_last": Value Change {
        n558 = event-data() -> ()  [unwired: 1 in, 6 out]
        n559 = local read "REPORT_filters"() -> (w1165:T2)
        n560 = case shown="\"Audits\"" w1165 {
          tunnel: w1164 -> [w1167 w1169 w1172 w1175 w1178 w1181 w1184 w1187 w1190 w1192]
          tunnel: [w1167 w1168 w1171 w1174 w1177 w1180 w1183 w1186 w1189 w1192] -> w1163
          frame "Gear" {
          }
          frame "Dates" {
            n561 = call "FGV_REPORTS_records_display.vi"("options"=FGV_REPORTS_records_display."DATES_last_page", "error_in"=w1169) -> ("error_out"=w1168:errorcluster)  [unwired: 8 in, 1 out]
          }
          frame "Production Batch" {
            n562 = call "FGV_REPORTS_records_display.vi"("options"=FGV_REPORTS_records_display."PBATCH_last_page", "error_in"=w1172) -> ("error_out"=w1171:errorcluster)  [unwired: 8 in, 1 out]
          }
          frame "Operation" {
            n563 = call "FGV_REPORTS_records_display.vi"("options"=FGV_REPORTS_records_display."OPRTN_last_page", "error_in"=w1175) -> ("error_out"=w1174:errorcluster)  [unwired: 8 in, 1 out]
          }
          frame "Config History" {
            n564 = call "FGV_REPORTS_records_display.vi"("options"=FGV_REPORTS_records_display."CFG_last_page", "error_in"=w1178) -> ("error_out"=w1177:errorcluster)  [unwired: 8 in, 1 out]
          }
          frame "Audits" {
            n565 = call "FGV_REPORTS_records_display.vi"("options"=FGV_REPORTS_records_display."AUDIT_last_page", "error_in"=w1181) -> ("error_out"=w1180:errorcluster)  [unwired: 8 in, 1 out]
          }
          frame "Reworks" {
            n566 = call "FGV_REPORTS_records_display.vi"("options"=FGV_REPORTS_records_display."REWORKS_last_page", "error_in"=w1184) -> ("error_out"=w1183:errorcluster)  [unwired: 8 in, 1 out]
          }
          frame "Customer Batch" {
            n567 = call "FGV_REPORTS_records_display.vi"("options"=FGV_REPORTS_records_display."CBATCH_last_page", "error_in"=w1187) -> ("error_out"=w1186:errorcluster)  [unwired: 8 in, 1 out]
          }
          frame "Gear Components" {
            n568 = call "FGV_REPORTS_records_display.vi"("options"=FGV_REPORTS_records_display."CMPNT_last_page", "error_in"=w1190) -> ("error_out"=w1189:errorcluster)  [unwired: 8 in, 1 out]
          }
          frame Default {
          }
        }
      }
      event "REPORT_page_next": Value Change {
        n569 = event-data() -> ()  [unwired: 1 in, 6 out]
        n570 = local read "REPORT_filters"() -> (w1195:T2)
        n571 = case shown="\"Audits\"" w1195 {
          tunnel: w1194 -> [w1197 w1199 w1202 w1205 w1208 w1211 w1214 w1217 w1220 w1222]
          tunnel: [w1197 w1198 w1201 w1204 w1207 w1210 w1213 w1216 w1219 w1222] -> w1193
          frame "Gear" {
          }
          frame "Dates" {
            n572 = call "FGV_REPORTS_records_display.vi"("options"=FGV_REPORTS_records_display."DATES_next_page", "error_in"=w1199) -> ("error_out"=w1198:errorcluster)  [unwired: 8 in, 1 out]
          }
          frame "Production Batch" {
            n573 = call "FGV_REPORTS_records_display.vi"("options"=FGV_REPORTS_records_display."PBATCH_next_page", "error_in"=w1202) -> ("error_out"=w1201:errorcluster)  [unwired: 8 in, 1 out]
          }
          frame "Operation" {
            n574 = call "FGV_REPORTS_records_display.vi"("options"=FGV_REPORTS_records_display."OPRTN_next_page", "error_in"=w1205) -> ("error_out"=w1204:errorcluster)  [unwired: 8 in, 1 out]
          }
          frame "Config History" {
            n575 = call "FGV_REPORTS_records_display.vi"("options"=FGV_REPORTS_records_display."CFG_next_page", "error_in"=w1208) -> ("error_out"=w1207:errorcluster)  [unwired: 8 in, 1 out]
          }
          frame "Audits" {
            n576 = call "FGV_REPORTS_records_display.vi"("options"=FGV_REPORTS_records_display."AUDIT_next_page", "error_in"=w1211) -> ("error_out"=w1210:errorcluster)  [unwired: 8 in, 1 out]
          }
          frame "Reworks" {
            n577 = call "FGV_REPORTS_records_display.vi"("options"=FGV_REPORTS_records_display."REWORKS_next_page", "error_in"=w1214) -> ("error_out"=w1213:errorcluster)  [unwired: 8 in, 1 out]
          }
          frame "Customer Batch" {
            n578 = call "FGV_REPORTS_records_display.vi"("options"=FGV_REPORTS_records_display."CBATCH_next_page", "error_in"=w1217) -> ("error_out"=w1216:errorcluster)  [unwired: 8 in, 1 out]
          }
          frame "Gear Components" {
            n579 = call "FGV_REPORTS_records_display.vi"("options"=FGV_REPORTS_records_display."CMPNT_next_page", "error_in"=w1220) -> ("error_out"=w1219:errorcluster)  [unwired: 8 in, 1 out]
          }
          frame Default {
          }
        }
      }
      event "REPORT_page_previous": Value Change {
        n580 = event-data() -> ()  [unwired: 1 in, 6 out]
        n581 = local read "REPORT_filters"() -> (w1225:T2)
        n582 = case shown="\"Gear Components\"" w1225 {
          tunnel: w1224 -> [w1227 w1229 w1232 w1235 w1238 w1241 w1244 w1247 w1250 w1252]
          tunnel: [w1227 w1228 w1231 w1234 w1237 w1240 w1243 w1246 w1249 w1252] -> w1223
          frame "Gear" {
          }
          frame "Dates" {
            n583 = call "FGV_REPORTS_records_display.vi"("options"=FGV_REPORTS_records_display."DATES_previous_page", "error_in"=w1229) -> ("error_out"=w1228:errorcluster)  [unwired: 8 in, 1 out]
          }
          frame "Production Batch" {
            n584 = call "FGV_REPORTS_records_display.vi"("options"=FGV_REPORTS_records_display."PBATCH_previous_page", "error_in"=w1232) -> ("error_out"=w1231:errorcluster)  [unwired: 8 in, 1 out]
          }
          frame "Operation" {
            n585 = call "FGV_REPORTS_records_display.vi"("options"=FGV_REPORTS_records_display."OPRTN_previous_page", "error_in"=w1235) -> ("error_out"=w1234:errorcluster)  [unwired: 8 in, 1 out]
          }
          frame "Config History" {
            n586 = call "FGV_REPORTS_records_display.vi"("options"=FGV_REPORTS_records_display."CFG_previous_page", "error_in"=w1238) -> ("error_out"=w1237:errorcluster)  [unwired: 8 in, 1 out]
          }
          frame "Audits" {
            n587 = call "FGV_REPORTS_records_display.vi"("options"=FGV_REPORTS_records_display."AUDIT_previous_page", "error_in"=w1241) -> ("error_out"=w1240:errorcluster)  [unwired: 8 in, 1 out]
          }
          frame "Reworks" {
            n588 = call "FGV_REPORTS_records_display.vi"("options"=FGV_REPORTS_records_display."REWORKS_previous_page", "error_in"=w1244) -> ("error_out"=w1243:errorcluster)  [unwired: 8 in, 1 out]
          }
          frame "Customer Batch" {
            n589 = call "FGV_REPORTS_records_display.vi"("options"=FGV_REPORTS_records_display."CBATCH_previous_page", "error_in"=w1247) -> ("error_out"=w1246:errorcluster)  [unwired: 8 in, 1 out]
          }
          frame "Gear Components" {
            n590 = call "FGV_REPORTS_records_display.vi"("options"=FGV_REPORTS_records_display."CMPNT_previous_page", "error_in"=w1250) -> ("error_out"=w1249:errorcluster)  [unwired: 8 in, 1 out]
          }
          frame Default {
          }
        }
      }
      event "REPORT_PBATCH_order_selection": Value Change {
        n591 = event-data() -> ()  [unwired: 1 in, 6 out]
        n592 = property on="REPORT_PBATCH_last_op" class="Ring (strict)"() -> ("RingText.Text"=w1255:string)  [unwired: 2 in, 2 out]
        n593 = property on="REPORT_PBATCH_last_status" class="Ring (strict)"() -> ("RingText.Text"=w1254:string)  [unwired: 2 in, 2 out]
        n594 = local read "REPORT_PBATCH_order_selection"() -> (w1256:enum32{"old_to_new", "new_to_old"})
        n595 = Bundle By Name(cluster=T40 {"order_selection"=enum."new_to_old", "last_OP"="", "last_status"=""} ("REPORT_DATES_filters"), "order_selection"=w1256, "last_OP"=w1255, "last_status"=w1254) -> (w1257:T40)
        n596 = To Variant(anything=w1257) -> (Variant=w1258:variant)
        n597 = call "FGV_REPORTS_records_display.vi"("options"=FGV_REPORTS_records_display."PBATCH_filter", "error_in"=w1261, "input"=w1258) -> ("error_out"=w1260:errorcluster)  [unwired: 7 in, 1 out]
      }
      event "REPORT_records": Double Click {
        n598 = event-data() -> ("Row"=w1266:i32)  [unwired: 1 in]
        n599 = local read "REPORT_filters"() -> (w1269:T2)
        n600 = case shown="\"Audits\"" w1269 {
          tunnel: [w1274 w1289 w1305 w1316 w1328] -> w1268
          tunnel: w1267 -> [w1279 w1290 w1306 w1322 w1328]
          tunnel: w1266 -> [w1276 w1284 w1300 w1323 _]
          tunnel: w1265 -> [_ w1288 w1304 _ _]
          tunnel: w1264 -> [w1271 w1287 w1303 w1326 w1327]
          tunnel: [w1271 w1286 w1302 w1326 w1327] -> w1263
          frame "Gear" {
            n601 = To Variant(anything=w1276) -> (Variant=w1277:variant)
            n602 = call "FGV_REPORTS_records_display.vi"("options"=FGV_REPORTS_records_display."GEAR_toggle_results", "error_in"=w1279, "input"=w1277) -> ("error_out"=w1275:errorcluster)  [unwired: 7 in, 1 out]
            n603 = property on="REPORT_GEAR_station" class="Ring (strict)"() -> ("RingText.Text"=w1270:string)  [unwired: 2 in, 2 out]
            n604 = To Variant(anything=w1270) -> (Variant=w1272:variant)
            n605 = call "FGV_REPORTS_records_display.vi"("options"=FGV_REPORTS_records_display."GEAR_filter", "error_in"=w1275, "input"=w1272) -> ("error_out"=w1274:errorcluster)  [unwired: 7 in, 1 out]
          }
          frame "Dates", "Production Batch" {
            n606 = property on="REPORT_records" class="MCListbox (strict)"() -> ("ItemNames"=w1285:string[][])  [unwired: 2 in, 2 out]
            n607 = Unbundle By Name(w1288) -> ("queue_refnums.SQL_EDITOR_queue"=w1294:refnum<queue>)
            n608 = Index Array(array=w1285, index (row)=w1284, index (col)=2 ("disabled index (col)")) -> (element=w1281:string)
            n609 = call-poly "Get Localized Phrase Compact Interface.vi"("Key"="SHOW ALL RESULTS" ("Boolean Text.Text")) -> ("Translated Phrase"=w1280:string)
            n610 = property on="REPORT_GEAR_toggle_all_results" class="Bool"("BoolText.Text"=w1280) -> ()  [unwired: 2 in, 2 out]
            n611 = local write "REPORT_GEAR_serial"(w1281) -> ()
            n612 = flat-sequence {
              tunnel: [T32 {"state"=enum."REPORT_GEAR_get", "variable"=variant} ("element")] -> w1293
              tunnel: w1281 -> [_]
              frame #0 {
              }
            }
            n613 = Bundle By Name(cluster=w1287, "REPORT_GEAR_toggle_all_results"=FALSE) -> (w1286:T21)
            n614 = Enqueue Element(queue=w1294, element=w1293, error in (no error)=w1290) -> (error out=w1289:errorcluster)  [unwired: 1 in, 2 out]
            n615 = property on="REPORT_filters" class="TabCtl (strict)"("Val(Sgnl)"=REPORTS_filters."Gear" ("REPORT_filters")) -> ()  [unwired: 2 in, 2 out]
          }
          frame "Operation", "Reworks", "Customer Batch" {
            n616 = property on="REPORT_records" class="MCListbox (strict)"() -> ("ItemNames"=w1301:string[][])  [unwired: 2 in, 2 out]
            n617 = Unbundle By Name(w1304) -> ("queue_refnums.SQL_EDITOR_queue"=w1310:refnum<queue>)
            n618 = Index Array(array=w1301, index (row)=w1300, index (col)=0 ("disabled index (col)")) -> (element=w1297:string)
            n619 = call-poly "Get Localized Phrase Compact Interface.vi"("Key"="SHOW ALL RESULTS" ("Boolean Text.Text")) -> ("Translated Phrase"=w1296:string)
            n620 = property on="REPORT_GEAR_toggle_all_results" class="Bool"("BoolText.Text"=w1296) -> ()  [unwired: 2 in, 2 out]
            n621 = local write "REPORT_GEAR_serial"(w1297) -> ()
            n622 = flat-sequence {
              tunnel: [T32 {"state"=enum."REPORT_GEAR_get", "variable"=variant} ("element")] -> w1309
              tunnel: w1297 -> [_]
              frame #0 {
              }
            }
            n623 = Bundle By Name(cluster=w1303, "REPORT_GEAR_toggle_all_results"=FALSE) -> (w1302:T21)
            n624 = Enqueue Element(queue=w1310, element=w1309, error in (no error)=w1306) -> (error out=w1305:errorcluster)  [unwired: 1 in, 2 out]
            n625 = property on="REPORT_filters" class="TabCtl (strict)"("Val(Sgnl)"=REPORTS_filters."Gear" ("REPORT_filters")) -> ()  [unwired: 2 in, 2 out]
          }
          frame "Audits" {
            n626 = local read "REPORT_AUDIT_order_selection"() -> (w1313:enum32{"old_to_new", "new_to_old"})
            n627 = property on="REPORT_AUDIT_OP_filter" class="Ring (strict)"() -> ("RingText.Text"=w1320:string)  [unwired: 2 in, 2 out]
            n628 = property on="REPORT_AUDIT_status_filter" class="Ring (strict)"() -> ("RingText.Text"=w1319:string)  [unwired: 2 in, 2 out]
            n629 = To Variant(anything=w1323) -> (Variant=w1324:variant)
            n630 = call "FGV_REPORTS_records_display.vi"("options"=FGV_REPORTS_records_display."AUDIT_toggle_results", "error_in"=w1322, "input"=w1324) -> ("error_out"=w1317:errorcluster)  [unwired: 7 in, 1 out]
            n631 = Bundle By Name(cluster=T35 {"order_selection"=enum."new_to_old", "OP_filter"="", "status_filter"="", "show_hidden?"=FALSE}, "order_selection"=w1313, "OP_filter"=w1320, "status_filter"=w1319, "show_hidden?"=TRUE) -> (w1315:T35)
            n632 = To Variant(anything=w1315) -> (Variant=w1314:variant)
            n633 = call "FGV_REPORTS_records_display.vi"("options"=FGV_REPORTS_records_display."AUDIT_filter", "error_in"=w1317, "input"=w1314) -> ("error_out"=w1316:errorcluster)  [unwired: 7 in, 1 out]
          }
          frame Default {
          }
        }
      }
      event "REPORT_records": Edit Cell? {
        n634 = event-data() -> ()  [unwired: 1 in, 1 out]
        n635 = event-data("Discard?"=TRUE) -> ()  [unwired: 1 in, 1 out]
      }
      event "REPORT_REWORKS_end_btn": Value Change {
        n636 = event-data() -> ()  [unwired: 1 in, 6 out]
        n637 = local read "REPORT_REWORKS_end"() -> (w1332:timestamp)
        n638 = call "custom_picktime.vi"("secin"=w1332) -> ("ok"=w1333:bool, "secout"=w1334:timestamp)  [unwired: 9 in]
        n639 = case shown="True" w1333 {
          tunnel: w1334 -> [_ w1337]
          frame False {
          }
          frame True {
            n640 = local write "REPORT_REWORKS_end"(w1337) -> ()
          }
        }
      }
      event "REPORT_REWORKS_order_selection": Value Change {
        n641 = event-data() -> ()  [unwired: 1 in, 6 out]
        n642 = local read "REPORT_REWORKS_order_selection"() -> (w1338:enum32{"old_to_new", "new_to_old"})
        n643 = To Variant(anything=w1338) -> (Variant=w1339:variant)
        n644 = call "FGV_REPORTS_records_display.vi"("options"=FGV_REPORTS_records_display."REWORKS_filter", "error_in"=w1342, "input"=w1339) -> ("error_out"=w1341:errorcluster)  [unwired: 7 in, 1 out]
      }
      event "REPORT_REWORKS_start_btn": Value Change {
        n645 = event-data() -> ()  [unwired: 1 in, 6 out]
        n646 = local read "REPORT_REWORKS_start"() -> (w1344:timestamp)
        n647 = call "custom_picktime.vi"("secin"=w1344) -> ("ok"=w1345:bool, "secout"=w1346:timestamp)  [unwired: 9 in]
        n648 = case shown="True" w1345 {
          tunnel: w1346 -> [_ w1349]
          frame False {
          }
          frame True {
            n649 = local write "REPORT_REWORKS_start"(w1349) -> ()
          }
        }
      }
      event "REPORT_save_csv": Value Change {
        n650 = event-data() -> ()  [unwired: 1 in, 6 out]
        n651 = Unbundle By Name(w1351) -> ("queue_refnums.SQL_EDITOR_queue"=w1354:refnum<queue>)
        n652 = Enqueue Element(queue=w1354, element=T32 {"state"=enum."REPORT_save_csv", "variable"=variant}, error in (no error)=w1353) -> (error out=w1352:errorcluster)  [unwired: 1 in, 2 out]
      }
      event "REPORT_save_pdf": Value Change {
        n653 = event-data() -> ()  [unwired: 1 in, 6 out]
        n654 = Unbundle By Name(w1357) -> ("queue_refnums.SQL_EDITOR_queue"=w1360:refnum<queue>)
        n655 = Enqueue Element(queue=w1360, element=T32 {"state"=enum."REPORT_save_pdf", "variable"=variant}, error in (no error)=w1359) -> (error out=w1358:errorcluster)  [unwired: 1 in, 2 out]
      }
      event "SQL_EDIT_asc_desc": Value Change {
        n656 = event-data() -> ("NewVal"=w1362:enum32{"ASC", "DESC"})  [unwired: 1 in, 5 out]
        n657 = To Variant(anything=w1362) -> (Variant=w1364:variant)
        n658 = call "FGV_SQL_EDITOR_records_display.vi"("options"=FGV_SQL_EDITOR_records_display."set_asc_desc", "error_in"=w1366, "input"=w1364) -> ("error_out"=w1365:errorcluster)  [unwired: 5 in, 3 out]
      }
      event "SQL_EDIT_clear_status": Value Change {
        n659 = event-data() -> ()  [unwired: 1 in, 6 out]
        n660 = call "FGV_SQL_EDITOR_status_display.vi"("options"=FGV_SQL_EDITOR_status_display."clear", "error_in"=w1370) -> ("error_out"=w1369:errorcluster)  [unwired: 9 in]
      }
      event "SQL_EDIT_column": Value Change {
        n661 = event-data() -> ("CtlRef"=w1378:refnum<vi>)  [unwired: 1 in, 5 out]
        n662 = property class="Ring (strict)"(reference=w1378) -> ("RingText.Text"=w1373:string)  [unwired: 1 in, 2 out]
        n663 = To Variant(anything=w1373) -> (Variant=w1374:variant)
        n664 = call "FGV_SQL_EDITOR_records_display.vi"("options"=FGV_SQL_EDITOR_records_display."set_column_name", "error_in"=w1376, "input"=w1374) -> ("error_out"=w1375:errorcluster)  [unwired: 5 in, 3 out]
      }
      event "SQL_EDIT_delete": Value Change {
        n665 = event-data() -> ()  [unwired: 1 in, 6 out]
        n666 = local read "SQL_EDIT_records"() -> (w1379:i32)
        n667 = case shown="-1" w1379 {
          tunnel: w1382 -> [_ w1394]
          tunnel: [w1388 w1393] -> w1381
          tunnel: w1380 -> [_ w1392]
          frame -1 {
            n668 = call-poly "Get Localized Phrase Compact Interface.vi"("Key"="No record selected for DELETE" ("source")) -> ("Translated Phrase"=w1385:string)
            n669 = Bundle By Name(cluster=errorcluster {"status"=FALSE, "code"=503, "source"=""} ("error out"), "source"=w1385) -> (w1384:errorcluster)
            n670 = call "FGV_SQL_EDITOR_status_display.vi"("options"=FGV_SQL_EDITOR_status_display."display", "error_in"=w1384, "display_source"="DELETE") -> ("error_out"=w1388:errorcluster)  [unwired: 8 in]
          }
          frame Default {
            n671 = Unbundle By Name(w1392) -> ("queue_refnums.SQL_EDITOR_queue"=w1395:refnum<queue>)
            n672 = Enqueue Element(queue=w1395, element=T32 {"state"=enum."SQL_delete_record", "variable"=variant}, error in (no error)=w1394) -> (error out=w1393:errorcluster)  [unwired: 1 in, 2 out]
          }
        }
      }
      event "SQL_EDIT_discard": Value Change {
        n673 = event-data() -> ()  [unwired: 1 in, 6 out]
        n674 = local read "SQL_EDIT_records"() -> (w1398:i32)
        n675 = case shown="Default" w1398 {
          selector: w1398 -> [_ w1404]
          tunnel: w1397 -> [w1400 w1402]
          tunnel: [w1400 w1401] -> w1396
          frame -1 {
          }
          frame Default {
            n676 = To Variant(anything=w1404) -> (Variant=w1405:variant)
            n677 = call "FGV_SQL_EDITOR_records_display.vi"("options"=FGV_SQL_EDITOR_records_display."discard_changes", "error_in"=w1402, "input"=w1405) -> ("error_out"=w1401:errorcluster)  [unwired: 5 in, 3 out]
          }
        }
      }
      event "SQL_EDIT_insert_update": Value Change {
        n678 = event-data() -> ()  [unwired: 1 in, 6 out]
        n679 = local read "SQL_EDIT_records"() -> (w1406:i32)
        n680 = case shown="Default" w1406 {
          selector: w1406 -> [_ w1419]
          tunnel: w1409 -> [_ w1425]
          tunnel: [w1415 w1424] -> w1408
          tunnel: w1407 -> [_ w1423]
          frame -1 {
            n681 = call-poly "Get Localized Phrase Compact Interface.vi"("Key"="No record selected for INSERT / UPDATE" ("source")) -> ("Translated Phrase"=w1412:string)
            n682 = Bundle By Name(cluster=errorcluster {"status"=FALSE, "code"=503, "source"=""} ("error out"), "source"=w1412) -> (w1411:errorcluster)
            n683 = call "FGV_SQL_EDITOR_status_display.vi"("options"=FGV_SQL_EDITOR_status_display."display", "error_in"=w1411, "display_source"="INSERT / UPDATE") -> ("error_out"=w1415:errorcluster)  [unwired: 8 in]
          }
          frame Default {
            n684 = call "FGV_SQL_EDITOR_records_display.vi"("options"=FGV_SQL_EDITOR_records_display."get_all_info") -> ("all_info"=w1421:T48)  [unwired: 7 in, 3 out]
            n685 = Unbundle By Name(w1421) -> ("SQL_record_states"=w1420:T44[])
            n686 = Index Array(array=w1420, index=w1419) -> (element=w1418:T44)
            n687 = case shown="\"Equal\"" w1418 {
              tunnel: w1425 -> [_ w1435 w1441]
              tunnel: [w1430 w1434 w1440] -> w1424
              tunnel: w1423 -> [_ w1433 w1439]
              frame "Equal" {
                n688 = call-poly "Get Localized Phrase Compact Interface.vi"("Key"="Record is already up to date with database" ("source")) -> ("Translated Phrase"=w1428:string)
                n689 = Bundle By Name(cluster=errorcluster {"status"=FALSE, "code"=502, "source"=""} ("error out"), "source"=w1428) -> (w1426:errorcluster)
                n690 = call "FGV_SQL_EDITOR_status_display.vi"("options"=FGV_SQL_EDITOR_status_display."display", "error_in"=w1426, "display_source"="INSERT / UPDATE") -> ("error_out"=w1430:errorcluster)  [unwired: 8 in]
              }
              frame "Added", "Deleted" {
                n691 = Unbundle By Name(w1433) -> ("queue_refnums.SQL_EDITOR_queue"=w1437:refnum<queue>)
                n692 = Enqueue Element(queue=w1437, element=T32 {"state"=enum."SQL_insert_record", "variable"=variant}, error in (no error)=w1435) -> (error out=w1434:errorcluster)  [unwired: 1 in, 2 out]
              }
              frame "Edited" {
                n693 = Unbundle By Name(w1439) -> ("queue_refnums.SQL_EDITOR_queue"=w1442:refnum<queue>)
                n694 = Enqueue Element(queue=w1442, element=T32 {"state"=enum."SQL_update_record", "variable"=variant}, error in (no error)=w1441) -> (error out=w1440:errorcluster)  [unwired: 1 in, 2 out]
              }
            }
          }
        }
      }
      event "SQL_EDIT_order_by": Value Change {
        n695 = event-data() -> ("CtlRef"=w1449:refnum<vi>)  [unwired: 1 in, 5 out]
        n696 = property class="Ring (strict)"(reference=w1449) -> ("RingText.Text"=w1444:string)  [unwired: 1 in, 2 out]
        n697 = To Variant(anything=w1444) -> (Variant=w1445:variant)
        n698 = call "FGV_SQL_EDITOR_records_display.vi"("options"=FGV_SQL_EDITOR_records_display."set_order_by", "error_in"=w1447, "input"=w1445) -> ("error_out"=w1446:errorcluster)  [unwired: 5 in, 3 out]
      }
      event "SQL_EDIT_records": Double Click {
        # "Workaround for delay of editting multicolumn listbox (without this editting possible after two clicks with 1sec. break between them)"
        n699 = event-data() -> ("CtlRef"=w1453:refnum<vi>, "Coords"=w1452:T45)  [unwired: 1 in]
        n700 = invoke class="MCListbox (strict)" method="Point To Row Column"(reference=w1453, "Point"=w1452) -> (reference out=w1456:refnum<vi>, error out=w1455:errorcluster, "CellPosition"=w1454:T36)  [unwired: 5 in, 4 out]
        n701 = property class="MCListbox (strict)"(reference=w1456, error in=w1455, "EditPos"=w1454) -> ()  [unwired: 2 out]
      }
      event "SQL_EDIT_records": Edit Cell {
        n702 = event-data() -> ("Coords.Row"=w1457:i32)  [unwired: 1 in]
        n703 = call "FGV_SQL_EDITOR_records_display.vi"("options"=FGV_SQL_EDITOR_records_display."get_all_info") -> ("all_info"=w1460:T48)  [unwired: 7 in, 3 out]
        n704 = Unbundle By Name(w1460) -> ("size.SQL_rows"=w1458:i32)
        n705 = local write "SQL_EDIT_records"(w1457) -> ()
        n706 = Greater Or Equal?(x=w1457, y=w1458) -> (x >= y?=w1459:bool)
        n707 = case shown="True" w1459 {
          tunnel: w1457 -> [w1466 w1469]
          frame False {
            n708 = To Variant(anything=w1466) -> (Variant=w1465:variant)
            n709 = call "FGV_SQL_EDITOR_records_display.vi"("options"=FGV_SQL_EDITOR_records_display."record_edited?", "input"=w1465) -> ()  [unwired: 6 in, 4 out]
          }
          frame True {
            n710 = To Variant(anything=w1469) -> (Variant=w1468:variant)
            n711 = call "FGV_SQL_EDITOR_records_display.vi"("options"=FGV_SQL_EDITOR_records_display."record_added?", "input"=w1468) -> ()  [unwired: 6 in, 4 out]
          }
        }
      }
      event "SQL_EDIT_records": Key Down? {
        n712 = event-data() -> ("CtlRef"=w1472:refnum<vi>, "ScanCode"=w1474:i16, "PlatMods.Shift"=w1470:bool)  [unwired: 1 in, 1 out]
        n713 = case shown="72" w1474 {
          tunnel: [_ TRUE w1483 w1494 w1505 w1516] -> w1473
          tunnel: w1472 -> [_ w1481 w1485 w1496 w1507 w1518]
          tunnel: w1470 -> [_ _ w1484 w1495 w1506 w1517]
          frame Default {
          }
          frame 15 {
            # "15 = Tab"
            n714 = call "FGV_SQL_EDITOR_records_display.vi"("options"=FGV_SQL_EDITOR_records_display."get_all_info") -> ("all_info"=w1476:T48)  [unwired: 7 in, 3 out]
            n715 = Unbundle By Name(w1476) -> ("editable_columns"=w1479:i32[], "size.SQL_rows"=w1478:i32)
            n716 = call "EDITORS_calculate_next_pos_for_keyboard_events.vi"("direction"=directions."RIGHT", "SQL_rows"=w1478, "editable_columns"=w1479, "reference"=w1481) -> ()  [unwired: 8 in]
          }
          frame 75 {
            # "75 = Left Arrow"
            n717 = case shown="True" w1484 {
              tunnel: w1485 -> [_ w1493]
              tunnel: [FALSE TRUE] -> w1483
              frame False {
              }
              frame True {
                n718 = call "FGV_SQL_EDITOR_records_display.vi"("options"=FGV_SQL_EDITOR_records_display."get_all_info") -> ("all_info"=w1487:T48)  [unwired: 7 in, 3 out]
                n719 = Unbundle By Name(w1487) -> ("editable_columns"=w1490:i32[], "size.SQL_rows"=w1489:i32)
                n720 = call "EDITORS_calculate_next_pos_for_keyboard_events.vi"("direction"=directions."LEFT", "SQL_rows"=w1489, "editable_columns"=w1490, "reference"=w1493) -> ()  [unwired: 8 in]
              }
            }
          }
          frame 77 {
            # "77 = Right Arrow"
            n721 = case shown="True" w1495 {
              tunnel: w1496 -> [_ w1504]
              tunnel: [FALSE TRUE] -> w1494
              frame False {
              }
              frame True {
                n722 = call "FGV_SQL_EDITOR_records_display.vi"("options"=FGV_SQL_EDITOR_records_display."get_all_info") -> ("all_info"=w1499:T48)  [unwired: 7 in, 3 out]
                n723 = Unbundle By Name(w1499) -> ("editable_columns"=w1501:i32[], "size.SQL_rows"=w1500:i32)
                n724 = call "EDITORS_calculate_next_pos_for_keyboard_events.vi"("direction"=directions."RIGHT", "SQL_rows"=w1500, "editable_columns"=w1501, "reference"=w1504) -> ()  [unwired: 8 in]
              }
            }
          }
          frame 72 {
            # "72 = Up Arrow"
            n725 = case shown="True" w1506 {
              tunnel: w1507 -> [_ w1515]
              tunnel: [FALSE TRUE] -> w1505
              frame False {
              }
              frame True {
                n726 = call "FGV_SQL_EDITOR_records_display.vi"("options"=FGV_SQL_EDITOR_records_display."get_all_info") -> ("all_info"=w1510:T48)  [unwired: 7 in, 3 out]
                n727 = Unbundle By Name(w1510) -> ("editable_columns"=w1512:i32[], "size.SQL_rows"=w1511:i32)
                n728 = call "EDITORS_calculate_next_pos_for_keyboard_events.vi"("direction"=directions."UP", "SQL_rows"=w1511, "editable_columns"=w1512, "reference"=w1515) -> ()  [unwired: 8 in]
              }
            }
          }
          frame 80 {
            # "80 = Down Arrow"
            n729 = case shown="True" w1517 {
              tunnel: w1518 -> [_ w1526]
              tunnel: [FALSE TRUE] -> w1516
              frame False {
              }
              frame True {
                n730 = call "FGV_SQL_EDITOR_records_display.vi"("options"=FGV_SQL_EDITOR_records_display."get_all_info") -> ("all_info"=w1521:T48)  [unwired: 7 in, 3 out]
                n731 = Unbundle By Name(w1521) -> ("editable_columns"=w1523:i32[], "size.SQL_rows"=w1522:i32)
                n732 = call "EDITORS_calculate_next_pos_for_keyboard_events.vi"("direction"=directions."DOWN", "SQL_rows"=w1522, "editable_columns"=w1523, "reference"=w1526) -> ()  [unwired: 8 in]
              }
            }
          }
        }
        n733 = event-data("Discard?"=w1473) -> ()  [unwired: 1 in, 1 out]
      }
      event "SQL_EDIT_records": Mouse Down? {
        n734 = event-data() -> ("CtlRef"=w1535:refnum<vi>, "Coords"=w1534:T45)  [unwired: 1 in]
        n735 = invoke class="MCListbox (strict)" method="Point To Row Column"(reference=w1535, "Point"=w1534) -> ("InBounds"=w1527:bool, "CellPosition"=w1531:T36)  [unwired: 5 in, 5 out]
        n736 = local read "SQL_EDIT_records"() -> (w1528:i32)
        n737 = Bundle By Name(cluster=w1530, "SQL_EDIT_selected_row"=w1528) -> (w1529:T21)
        n738 = case shown="False" w1527 {
          selector: w1527 -> [w1537 _]
          tunnel: [w1537 w1542] -> w1533
          tunnel: [w1538 w1541] -> w1532
          tunnel: w1531 -> [_ w1540]
          tunnel: w1529 -> [w1538 w1539]
          frame False {
          }
          frame True {
            n739 = call "SQL_EDITOR_records_click_discard.vi"("CellPosition"=w1540, "event_structure_shift_register_in"=w1539) -> ("Discard?"=w1542:bool, "event_structure_shift_register_out"=w1541:T21)  [unwired: 8 in]
          }
        }
        n740 = event-data("Discard?"=w1533) -> ()  [unwired: 1 in, 1 out]
      }
      event "SQL_EDIT_records": Value Change {
        n741 = event-data() -> ("NewVal"=w1544:i32)  [unwired: 1 in, 5 out]
        n742 = Bundle By Name(cluster=w1545, "SQL_EDIT_selected_row"=w1544) -> (w1543:T21)
      }
      event "SQL_EDIT_select": Value Change {
        n743 = event-data() -> ()  [unwired: 1 in, 6 out]
        n744 = To Variant(anything="SQL_EDIT_value") -> (Variant=w1550:variant)
        n745 = call "FGV_SQL_EDITOR_records_display.vi"("options"=FGV_SQL_EDITOR_records_display."set_value_to_select", "error_in"=w1552, "input"=w1550) -> ("error_out"=w1551:errorcluster)  [unwired: 5 in, 3 out]
        n746 = Unbundle By Name(w1556) -> ("queue_refnums.SQL_EDITOR_queue"=w1554:refnum<queue>)
        n747 = Enqueue Element(queue=w1554, element=T32 {"state"=enum."SQL_select_records", "variable"=variant}, error in (no error)=w1551) -> (error out=w1555:errorcluster)  [unwired: 1 in, 2 out]
      }
      event "SQL_EDIT_table": Value Change {
        n748 = event-data() -> ("CtlRef"=w1564:refnum<vi>)  [unwired: 1 in, 5 out]
        n749 = property class="Ring (strict)"(reference=w1564) -> ("RingText.Text"=w1559:string)  [unwired: 1 in, 2 out]
        n750 = To Variant(anything=w1559) -> (Variant=w1560:variant)
        n751 = call "FGV_SQL_EDITOR_records_display.vi"("options"=FGV_SQL_EDITOR_records_display."set_table_name", "error_in"=w1562, "input"=w1560) -> ("error_out"=w1561:errorcluster)  [unwired: 5 in, 3 out]
        n752 = Unbundle By Name(w1567) -> ("queue_refnums.SQL_EDITOR_queue"=w1565:refnum<queue>)
        n753 = Enqueue Element(queue=w1565, element=T32 {"state"=enum."SQL_read_columns", "variable"=variant}, error in (no error)=w1561) -> (error out=w1566:errorcluster)  [unwired: 1 in, 2 out]
      }
      event "SQL_TEXT_clear_status": Value Change {
        n754 = event-data() -> ()  [unwired: 1 in, 6 out]
        n755 = call "FGV_SQL_TEXT_status_display.vi"("options"=FGV_SQL_TEXT_status_display."clear", "error_in"=w1572) -> ("error_out"=w1569:errorcluster)  [unwired: 9 in]
        n756 = call "FGV_SQL_TEXT_records_display.vi"("options"=FGV_SQL_TEXT_records_display."clear", "error_in"=w1569) -> ("error_out"=w1568:errorcluster)  [unwired: 9 in]
      }
      event "SQL_TEXT_execute": Value Change {
        n757 = event-data() -> ()  [unwired: 1 in, 6 out]
        n758 = Unbundle By Name(w1575) -> ("queue_refnums.SQL_EDITOR_queue"=w1578:refnum<queue>)
        n759 = Enqueue Element(queue=w1578, element=T32 {"state"=enum."SQL_TEXT_execute", "variable"=variant}, error in (no error)=w1577) -> (error out=w1576:errorcluster)  [unwired: 1 in, 2 out]
      }
      event "STOP": Value Change {
        n760 = event-data() -> ()  [unwired: 1 in, 1 out]
        n761 = disable-structure shown="RUN_TIME_ENGINE==True" {
          disable-tunnel: [w1589 TRUE ("Result")] -> w1581
          disable-tunnel: w1583 -> [w1588 w1600]
          disable-tunnel: [w1587 w1600] -> w1582
          frame condition #0 {
            n762 = case shown="No Error" w1588 {
              selector: w1588 -> [w1594 w1598]
              tunnel: [w1595 TRUE ("Result")] -> w1589
              tunnel: [w1593 w1598] -> w1587
              frame No Error {
                n763 = call "confirm_popup.vi"("Warning(T)/Inf(F)"=TRUE, "error_in"=w1594, "False Label"="No", "True Label"="Yes", "Message"="Are you sure you want to exit the application?") -> ("error_out"=w1593:errorcluster, "Result"=w1595:bool)  [unwired: 5 in]
              }
              frame Error {
              }
            }
          }
          frame condition #1 (active) {
          }
        }
        n764 = case shown="True" w1581 {
          tunnel: w1586 -> [_ w1615]
          tunnel: w1582 -> [w1602 w1612]
          tunnel: [w1602 w1605] -> w1584
          tunnel: [FALSE TRUE] -> w1580
          frame False {
          }
          frame True {
            n765 = Unbundle By Name(w1615) -> ("queue_refnums.CLIENT_REF_CHG_queue"=w1604:refnum<queue>, "queue_refnums.SCANNER_queue"=w1609:refnum<queue>, "queue_refnums.SQL_EDITOR_queue"=w1614:refnum<queue>)
            n766 = call <vilib>:"Clear Errors.vi"("error in (no error)"=w1612) -> ("error out"=w1611:errorcluster)  [unwired: 5 in, 1 out]
            n767 = Enqueue Element At Opposite End(queue=w1614, element=T32 {"state"=enum."stop", "variable"=variant}, error in (no error)=w1611) -> (error out=w1610:errorcluster)  [unwired: 1 in, 2 out]
            n768 = Enqueue Element At Opposite End(queue=w1609, element=T42 {"state"=enum."stop", "variable"=variant}, error in (no error)=w1610) -> (error out=w1606:errorcluster)  [unwired: 1 in, 2 out]
            n769 = Enqueue Element At Opposite End(queue=w1604, element=T41 {"state"=enum."stop", "variable"=variant}, error in (no error)=w1606) -> (error out=w1605:errorcluster)  [unwired: 1 in, 2 out]
          }
        }
      }
      event "USER_EDIT_clear_status": Value Change {
        n770 = event-data() -> ()  [unwired: 1 in, 6 out]
        n771 = call "FGV_USER_EDITOR_status_display.vi"("options"=FGV_USER_EDITOR_status_display."clear", "error_in"=w1617) -> ("error_out"=w1616:errorcluster)  [unwired: 9 in]
      }
      event "USER_EDIT_delete": Value Change {
        n772 = event-data() -> ()  [unwired: 1 in, 6 out]
        n773 = local read "USER_EDIT_records"() -> (w1620:i32)
        n774 = case shown="-1" w1620 {
          tunnel: w1623 -> [_ w1635]
          tunnel: [w1631 w1634] -> w1622
          tunnel: w1621 -> [_ w1633]
          frame -1 {
            n775 = call-poly "Get Localized Phrase Compact Interface.vi"("Key"="No record selected for DELETE" ("source")) -> ("Translated Phrase"=w1626:string)
            n776 = Bundle By Name(cluster=errorcluster {"status"=FALSE, "code"=503, "source"=""} ("error out"), "source"=w1626) -> (w1625:errorcluster)
            n777 = call "FGV_USER_EDITOR_status_display.vi"("options"=FGV_USER_EDITOR_status_display."display", "error_in"=w1625, "display_source"="DELETE") -> ("error_out"=w1631:errorcluster)  [unwired: 8 in]
          }
          frame Default {
            n778 = Unbundle By Name(w1633) -> ("queue_refnums.SQL_EDITOR_queue"=w1636:refnum<queue>)
            n779 = Enqueue Element(queue=w1636, element=T32 {"state"=enum."USER_delete_record", "variable"=variant}, error in (no error)=w1635) -> (error out=w1634:errorcluster)  [unwired: 1 in, 2 out]
          }
        }
      }
      event "USER_EDIT_discard": Value Change {
        n780 = event-data() -> ()  [unwired: 1 in, 6 out]
        n781 = local read "USER_EDIT_records"() -> (w1639:i32)
        n782 = case shown="Default" w1639 {
          selector: w1639 -> [_ w1646]
          tunnel: w1638 -> [w1641 w1644]
          tunnel: [w1641 w1643] -> w1637
          frame -1 {
          }
          frame Default {
            n783 = To Variant(anything=w1646) -> (Variant=w1645:variant)
            n784 = call "FGV_USER_EDITOR_records_display.vi"("options"=FGV_USER_EDITOR_records_display."discard_changes", "error_in"=w1644, "input"=w1645) -> ("error_out"=w1643:errorcluster)  [unwired: 5 in, 3 out]
          }
        }
      }
      event "USER_EDIT_insert_update": Value Change {
        n785 = event-data() -> ()  [unwired: 1 in, 6 out]
        n786 = local read "USER_EDIT_records"() -> (w1647:i32)
        n787 = case shown="Default" w1647 {
          selector: w1647 -> [_ w1662]
          tunnel: w1650 -> [_ w1666]
          tunnel: [w1657 w1665] -> w1649
          tunnel: w1648 -> [_ w1664]
          frame -1 {
            n788 = call-poly "Get Localized Phrase Compact Interface.vi"("Key"="No record selected for INSERT / UPDATE" ("source")) -> ("Translated Phrase"=w1653:string)
            n789 = Bundle By Name(cluster=errorcluster {"status"=FALSE, "code"=503, "source"=""} ("error out"), "source"=w1653) -> (w1652:errorcluster)
            n790 = call "FGV_ARCH_EDITOR_status_display.vi"("options"=FGV_ARCH_EDITOR_status_display."display", "error_in"=w1652, "display_source"="INSERT / UPDATE") -> ("error_out"=w1657:errorcluster)  [unwired: 8 in]
          }
          frame Default {
            n791 = call "FGV_USER_EDITOR_records_display.vi"("options"=FGV_USER_EDITOR_records_display."get_all_info") -> ("all_info"=w1659:T49)  [unwired: 7 in, 3 out]
            n792 = Unbundle By Name(w1659) -> ("USER_record_states"=w1663:T44[])
            n793 = Index Array(array=w1663, index=w1662) -> (element=w1661:T44)
            n794 = case shown="\"Equal\"" w1661 {
              tunnel: w1666 -> [_ w1677 w1682]
              tunnel: [w1673 w1676 w1681] -> w1665
              tunnel: w1664 -> [_ w1675 w1680]
              frame "Equal" {
                n795 = call-poly "Get Localized Phrase Compact Interface.vi"("Key"="Record is already up to date with database" ("source")) -> ("Translated Phrase"=w1669:string)
                n796 = Bundle By Name(cluster=errorcluster {"status"=FALSE, "code"=502, "source"=""} ("error out"), "source"=w1669) -> (w1667:errorcluster)
                n797 = call "FGV_USER_EDITOR_status_display.vi"("options"=FGV_USER_EDITOR_status_display."display", "error_in"=w1667, "display_source"="INSERT / UPDATE") -> ("error_out"=w1673:errorcluster)  [unwired: 8 in]
              }
              frame "Added", "Deleted" {
                n798 = Unbundle By Name(w1675) -> ("queue_refnums.SQL_EDITOR_queue"=w1678:refnum<queue>)
                n799 = Enqueue Element(queue=w1678, element=T32 {"state"=enum."USER_insert_record", "variable"=variant}, error in (no error)=w1677) -> (error out=w1676:errorcluster)  [unwired: 1 in, 2 out]
              }
              frame "Edited" {
                n800 = Unbundle By Name(w1680) -> ("queue_refnums.SQL_EDITOR_queue"=w1683:refnum<queue>)
                n801 = Enqueue Element(queue=w1683, element=T32 {"state"=enum."USER_update_record", "variable"=variant}, error in (no error)=w1682) -> (error out=w1681:errorcluster)  [unwired: 1 in, 2 out]
              }
            }
          }
        }
      }
      event "USER_EDIT_records": Double Click {
        # "Workaround for delay of editting multicolumn listbox (without this editting possible after two clicks with 1sec. break between them)"
        n802 = event-data() -> ("CtlRef"=w1687:refnum<vi>, "Coords"=w1686:T45)  [unwired: 1 in, 4 out]
        n803 = invoke class="MCListbox (strict)" method="Point To Row Column"(reference=w1687, "Point"=w1686) -> (reference out=w1690:refnum<vi>, error out=w1689:errorcluster, "CellPosition"=w1688:T36)  [unwired: 5 in, 4 out]
        n804 = property class="MCListbox (strict)"(reference=w1690, error in=w1689, "EditPos"=w1688) -> ()  [unwired: 2 out]
      }
      event "USER_EDIT_records": Edit Cell {
        n805 = event-data() -> ("Coords.Row"=w1693:i32)  [unwired: 1 in]
        n806 = call "FGV_USER_EDITOR_records_display.vi"("options"=FGV_USER_EDITOR_records_display."get_all_info") -> ("all_info"=w1691:T49)  [unwired: 7 in, 3 out]
        n807 = Unbundle By Name(w1691) -> ("size.SQL_rows"=w1694:i32)
        n808 = local write "USER_EDIT_records"(w1693) -> ()
        n809 = Greater Or Equal?(x=w1693, y=w1694) -> (x >= y?=w1695:bool)
        n810 = case shown="True" w1695 {
          tunnel: w1693 -> [w1700 w1703]
          frame False {
            n811 = To Variant(anything=w1700) -> (Variant=w1699:variant)
            n812 = call "FGV_USER_EDITOR_records_display.vi"("options"=FGV_USER_EDITOR_records_display."record_edited?", "input"=w1699) -> ()  [unwired: 6 in, 4 out]
          }
          frame True {
            n813 = To Variant(anything=w1703) -> (Variant=w1702:variant)
            n814 = call "FGV_USER_EDITOR_records_display.vi"("options"=FGV_USER_EDITOR_records_display."record_added?", "input"=w1702) -> ()  [unwired: 6 in, 4 out]
          }
        }
      }
      event "USER_EDIT_records": Key Down? {
        n815 = event-data() -> ("CtlRef"=w1708:refnum<vi>, "ScanCode"=w1710:i16, "PlatMods.Shift"=w1706:bool)  [unwired: 1 in, 1 out]
        n816 = call "FGV_USER_EDITOR_records_display.vi"("options"=FGV_USER_EDITOR_records_display."get_all_info") -> ("all_info"=w1705:T49)  [unwired: 7 in, 3 out]
        n817 = case shown="72" w1710 {
          tunnel: [_ TRUE w1719 w1730 w1741 w1752] -> w1709
          tunnel: w1708 -> [_ w1716 w1721 w1732 w1743 w1754]
          tunnel: w1706 -> [_ _ w1720 w1731 w1742 w1753]
          tunnel: w1705 -> [_ w1712 w1718 w1729 w1740 w1751]
          frame Default {
          }
          frame 15 {
            # "15 = Tab"
            n818 = Unbundle By Name(w1712) -> ("editable_columns"=w1714:i32[], "size.SQL_rows"=w1713:i32)
            n819 = call "EDITORS_calculate_next_pos_for_keyboard_events.vi"("direction"=directions."RIGHT", "SQL_rows"=w1713, "editable_columns"=w1714, "reference"=w1716) -> ()  [unwired: 8 in]
          }
          frame 75 {
            # "75 = Left Arrow"
            n820 = case shown="True" w1720 {
              tunnel: w1721 -> [_ w1728]
              tunnel: [FALSE TRUE] -> w1719
              tunnel: w1718 -> [_ w1723]
              frame False {
              }
              frame True {
                n821 = Unbundle By Name(w1723) -> ("editable_columns"=w1725:i32[], "size.SQL_rows"=w1724:i32)
                n822 = call "EDITORS_calculate_next_pos_for_keyboard_events.vi"("direction"=directions."LEFT", "SQL_rows"=w1724, "editable_columns"=w1725, "reference"=w1728) -> ()  [unwired: 8 in]
              }
            }
          }
          frame 77 {
            # "77 = Right Arrow"
            n823 = case shown="True" w1731 {
              tunnel: w1732 -> [_ w1739]
              tunnel: [FALSE TRUE] -> w1730
              tunnel: w1729 -> [_ w1734]
              frame False {
              }
              frame True {
                n824 = Unbundle By Name(w1734) -> ("editable_columns"=w1736:i32[], "size.SQL_rows"=w1735:i32)
                n825 = call "EDITORS_calculate_next_pos_for_keyboard_events.vi"("direction"=directions."RIGHT", "SQL_rows"=w1735, "editable_columns"=w1736, "reference"=w1739) -> ()  [unwired: 8 in]
              }
            }
          }
          frame 72 {
            # "72 = Up Arrow"
            n826 = case shown="True" w1742 {
              tunnel: w1743 -> [_ w1750]
              tunnel: [FALSE TRUE] -> w1741
              tunnel: w1740 -> [_ w1745]
              frame False {
              }
              frame True {
                n827 = Unbundle By Name(w1745) -> ("editable_columns"=w1747:i32[], "size.SQL_rows"=w1746:i32)
                n828 = call "EDITORS_calculate_next_pos_for_keyboard_events.vi"("direction"=directions."UP", "SQL_rows"=w1746, "editable_columns"=w1747, "reference"=w1750) -> ()  [unwired: 8 in]
              }
            }
          }
          frame 80 {
            # "80 = Down Arrow"
            n829 = case shown="True" w1753 {
              tunnel: w1754 -> [_ w1761]
              tunnel: [FALSE TRUE] -> w1752
              tunnel: w1751 -> [_ w1756]
              frame False {
              }
              frame True {
                n830 = Unbundle By Name(w1756) -> ("editable_columns"=w1758:i32[], "size.SQL_rows"=w1757:i32)
                n831 = call "EDITORS_calculate_next_pos_for_keyboard_events.vi"("direction"=directions."DOWN", "SQL_rows"=w1757, "editable_columns"=w1758, "reference"=w1761) -> ()  [unwired: 8 in]
              }
            }
          }
        }
        n832 = event-data("Discard?"=w1709) -> ()  [unwired: 1 in, 1 out]
      }
      event "USER_EDIT_records": Mouse Down? {
        n833 = event-data() -> ("CtlRef"=w1770:refnum<vi>, "Coords"=w1769:T45)  [unwired: 1 in]
        n834 = invoke class="MCListbox (strict)" method="Point To Row Column"(reference=w1770, "Point"=w1769) -> ("InBounds"=w1762:bool, "CellPosition"=w1764:T36)  [unwired: 5 in, 5 out]
        n835 = local read "USER_EDIT_records"() -> (w1767:i32)
        n836 = Bundle By Name(cluster=w1768, "USER_EDIT_selected_row"=w1767) -> (w1765:T21)
        n837 = case shown="True" w1762 {
          selector: w1762 -> [w1773 _]
          tunnel: [w1772 w1777] -> w1766
          tunnel: w1765 -> [w1772 w1776]
          tunnel: w1764 -> [_ w1775]
          tunnel: [w1773 w1774] -> w1763
          frame False {
          }
          frame True {
            n838 = call "USER_EDITOR_records_click_discard.vi"("CellPosition"=w1775, "event_structure_shift_register_in"=w1776) -> ("Discard?"=w1774:bool, "event_structure_shift_register_out"=w1777:T21)  [unwired: 8 in]
          }
        }
        n839 = event-data("Discard?"=w1763) -> ()  [unwired: 1 in, 1 out]
      }
      event "USER_EDIT_refresh": Value Change {
        n840 = event-data() -> ()  [unwired: 1 in, 6 out]
        n841 = Unbundle By Name(w1783) -> ("queue_refnums.SQL_EDITOR_queue"=w1781:refnum<queue>)
        n842 = Enqueue Element(queue=w1781, element=T32 {"state"=enum."USER_select_records", "variable"=variant}, error in (no error)=w1779) -> (error out=w1782:errorcluster)  [unwired: 1 in, 2 out]
      }
      event "USER_EDIT_update_barcode": Value Change {
        n843 = event-data() -> ()  [unwired: 1 in, 6 out]
        n844 = local read "USER_EDIT_records"() -> (w1787:i32)
        n845 = case shown="-1" w1787 {
          tunnel: w1785 -> [_ w1800]
          tunnel: [w1795 w1801] -> w1786
          tunnel: w1784 -> [_ w1798]
          frame -1 {
            n846 = call-poly "Get Localized Phrase Compact Interface.vi"("Key"="No record selected for barcode update" ("source")) -> ("Translated Phrase"=w1789:string)
            n847 = Bundle By Name(cluster=errorcluster {"status"=FALSE, "code"=503, "source"=""} ("error out"), "source"=w1789) -> (w1792:errorcluster)
            n848 = call "FGV_USER_EDITOR_status_display.vi"("options"=FGV_USER_EDITOR_status_display."display", "error_in"=w1792, "display_source"="UPDATE BARCODE") -> ("error_out"=w1795:errorcluster)  [unwired: 8 in]
          }
          frame Default {
            n849 = call "USER_EDITOR_scan_barcode.vi"("error_in"=w1800, "all_config_info"=w1798) -> ("error_out"=w1799:errorcluster, "Canceled?"=w1796:bool, "barcode"=w1797:string)  [unwired: 7 in]
            n850 = case shown="False" w1796 {
              tunnel: [w1808 w1810] -> w1801
              tunnel: w1799 -> [w1807 w1810]
              tunnel: w1798 -> [w1806 _]
              tunnel: w1797 -> [w1802 _]
              frame False {
                n851 = Unbundle By Name(w1806) -> ("queue_refnums.SQL_EDITOR_queue"=w1809:refnum<queue>)
                n852 = To Variant(anything=w1802) -> (Variant=w1803:variant)
                n853 = Bundle By Name(cluster=T32 {"state"=enum."USER_update_barcode", "variable"=variant} ("element"), "variable"=w1803) -> (w1804:T32)
                n854 = Enqueue Element(queue=w1809, element=w1804, error in (no error)=w1807) -> (error out=w1808:errorcluster)  [unwired: 1 in, 2 out]
              }
              frame True {
              }
            }
          }
        }
      }
      event "USER_login_logout": Value Change {
        n855 = event-data() -> ()  [unwired: 1 in, 6 out]
        n856 = local read "current_access_level"() -> (w1812:i32)
        n857 = case shown="0" w1812 {
          tunnel: [w1816 w1835] -> w1814
          tunnel: w1811 -> [w1818 w1833]
          tunnel: w1813 -> [w1817 w1832]
          frame 0 {
            n858 = call "LOGIN_scan_barcode.vi"("error_in"=w1818, "all_config_info"=w1817) -> ("error_out"=w1821:errorcluster, "Canceled?"=w1819:bool, "barcode"=w1820:string)  [unwired: 7 in]
            n859 = case shown="False" w1819 {
              tunnel: [w1829 w1830] -> w1816
              tunnel: w1821 -> [w1826 w1830]
              tunnel: w1817 -> [w1825 _]
              tunnel: w1820 -> [w1824 _]
              frame False {
                n860 = Unbundle By Name(w1825) -> ("queue_refnums.SQL_EDITOR_queue"=w1828:refnum<queue>)
                n861 = To Variant(anything=w1824) -> (Variant=w1827:variant)
                n862 = Bundle By Name(cluster=T32 {"state"=enum."USER_login", "variable"=variant} ("element"), "variable"=w1827) -> (w1822:T32)
                n863 = Enqueue Element(queue=w1828, element=w1822, error in (no error)=w1826) -> (error out=w1829:errorcluster)  [unwired: 1 in, 2 out]
              }
              frame True {
              }
            }
          }
          frame Default {
            n864 = Unbundle By Name(w1832) -> ("queue_refnums.SQL_EDITOR_queue"=w1834:refnum<queue>)
            n865 = Enqueue Element(queue=w1834, element=T32 {"state"=enum."USER_logout", "variable"=variant}, error in (no error)=w1833) -> (error out=w1835:errorcluster)  [unwired: 1 in, 2 out]
          }
        }
      }
      event Menu Selection (User) {
        n866 = event-data() -> ("ItemTag"=w1837:string)  [unwired: 1 in, 6 out]
        n867 = call "Get Key For Phrase.vi"("Phrase"=w1837) -> ("Key"=w1836:string)  [unwired: 9 in, 1 out]
        n868 = case shown="\"Exit\"" w1836 {
          selector: w1836 -> [_ w1842 _ _]
          frame Default {
          }
          frame "Language - English", "Language - Russian" {
            n869 = case shown="\"Language - Russian\"" w1842 {
              tunnel: ["Russian" ("Target Language (current lang)") "English" ("Target Language (current lang)")] -> w1843
              frame "Language - Russian" {
              }
              frame "Language - English", Default {
              }
            }
            n870 = call "Set Language.vi"("Target Language (current lang)"=w1843) -> ("error out"=w1840:errorcluster)  [unwired: 9 in, 1 out]
            n871 = Current VI's Menubar() -> (w1841:refnum<k9>)
            n872 = call "CLIENT_create_menu_bar.vi"("error_in"=w1840, "menu_bar_refnum"=w1841) -> ()  [unwired: 9 in, 1 out]
          }
          frame "About" {
            n873 = disable-structure shown="Default" {
              disable-tunnel: [w1852 w1855] -> w1848
              disable-tunnel: [w1853 w1855] -> w1847
              frame condition #0 {
                n874 = vi-ref "get_exe_compilation_date.vi"() -> (w1854:refnum<vi>)
                n875 = call-by-ref "?"(reference=w1854) -> ("compilation_time"=w1852:string, "compilation_date"=w1853:string)  [unwired: 10 in, 3 out]
              }
              frame condition #1 (active) {
                n876 = call-poly "Get Localized Phrase Compact Interface.vi"("Key"="NOT COMPILED!" ("compilation_date")) -> ("Translated Phrase"=w1855:string)
              }
            }
            n877 = call-poly "Get Localized Phrase Compact Interface.vi"("Key"="SQL Client Application\nMSG Assembly Line\nA603A00\n\nAumatic sp. z o.o.\nPilsudskiego 22\n32-050 Skawina\nPOLAND\n\nCOMPILATION DATE: %s\nCOMPILATION TIME: %s\nJakub Longa, 2021\n\n+48 (12) 256-77-90\naumatic.com" ("about_string")) -> ("Translated Phrase"=w1846:string)
            n878 = Format Into String(format string=w1846, w1847, w1848) -> (resulting string=w1851:string)  [unwired: 2 in, 1 out]
            n879 = call "about_window.vi"("lines_to_bold"=i32[] [0, 1, 4, 9], "about_string"=w1851) -> ()  [unwired: 9 in, 1 out]
          }
          frame "Exit" {
            n880 = property on="STOP" class="Bool (strict)"("Val(Sgnl)"=TRUE ("Value (Signaling)")) -> ()  [unwired: 2 in, 2 out]
          }
        }
      }
      event Panel Close? {
        n881 = event-data() -> ()  [unwired: 1 in, 4 out]
        n882 = property on="STOP" class="Bool (strict)"("Val(Sgnl)"=TRUE ("Value (Signaling)")) -> ()  [unwired: 2 in, 2 out]
        n883 = event-data("Discard?"=TRUE) -> ()  [unwired: 1 in, 1 out]
      }
      event Timeout {
        n884 = event-data() -> ()  [unwired: 1 in, 3 out]
        n885 = local read "current_access_level"() -> (w1862:i32)
        n886 = case shown="Default" w1862 {
          tunnel: w1864 -> [w1866 w1874]
          tunnel: [w1866 w1870] -> w1863
          frame 0 {
          }
          frame Default {
            n887 = call "FGV_login.vi"("options"=FGV_login."logout", "error_in"=w1874) -> ("error_out"=w1871:errorcluster)  [unwired: 7 in, 2 out]
            n888 = call "message_popup.vi"("Warning(T)/Info(F)"=TRUE, "error_in"=w1871, "Message"="Automatic user logout was performed due to inactivity", "Title"="Automatic Logout", "Button Label"="OK") -> ("error_out"=w1870:errorcluster)  [unwired: 6 in]
          }
        }
      }
    }
  }
  n889 = while {
    shift-right: [w1881] -> _
    shift-left: CLIENT_REF_CHG_sequence_state."initialize" ("SCANNER_sequence_state") -> [w1884]
    shift-right: [w1882] -> w20
    shift-left: w15 -> [w1883]
    tunnel: w21 -> [w1879]
    shift-right: [w1878] -> _
    shift-left: refnum<k5> refnum ("connection ID") -> [w1877]
    shift-right: [w1876] -> _
    shift-left: _ -> [w1875]
    stop <- w1880 stop-if-true
    # "REFERENCE CHANGED TCP CONNECTION TO PLC PROXY APP"
    n890 = case shown="\"error\"" w1884 {
      tunnel: w1883 -> [w1892 w1905 w1917 w1925 w1930 w1955]
      tunnel: [w1896 w1908 w1920 w1928 w1933 w1950] -> w1882
      tunnel: [w1894 w1907 w1919 w1927 w1940 CLIENT_REF_CHG_sequence_state."stop" ("state")] -> w1881
      tunnel: [_ _ _ _ _ TRUE] -> w1880
      tunnel: w1879 -> [w1893 w1903 _ _ w1943 _]
      tunnel: [w1888 w1906 w1915 w1923 refnum<k5> refnum ("connection ID") refnum<k5> refnum ("connection ID")] -> w1878
      tunnel: w1877 -> [_ w1906 w1915 w1923 w1935 w1951]
      tunnel: [_ w1899 _ _ _ _] -> w1876
      tunnel: w1875 -> [_ _ _ _ _ _]
      frame "initialize" {
        n891 = Unbundle By Name(w1893) -> ("main_ini_file.REF CHG connection IP"=w1891:string, "main_ini_file.REF CHG remote port"=w1890:i32, "main_ini_file.REF CHG local port"=w1886:i32)
        n892 = TCP Open Connection(address=w1891, remote port or service name=w1890, timeout ms (60000)=5000, local port=w1886, error in (no error)=w1892) -> (connection ID=w1888:refnum<k5>, error out=w1887:errorcluster)
        n893 = Unbundle By Name(w1887) -> ("status"=w1885:bool)
        n894 = property on="PLC_PROXY_connection_indicator" class="Bool (strict)"("Val(Sgnl)"=w1885) -> ()  [unwired: 2 in, 2 out]
        n895 = call "CLIENT_REF_CHG_check_for_error.vi"("CLIENT_REF_CHG_sequence_state_in"=CLIENT_REF_CHG_sequence_state."get_next_state" ("SQL_EDITOR_sequence_state"), "error_in"=w1887) -> ("CLIENT_REF_CHG_sequence_state_out"=w1894:T9, "error_out"=w1896:errorcluster)  [unwired: 8 in]
      }
      frame "get_next_state" {
        n896 = Unbundle By Name(w1903) -> ("queue_refnums.CLIENT_REF_CHG_queue"=w1902:refnum<queue>)
        n897 = Dequeue Element(queue=w1902, timeout in ms (-1)=2000, error in (no error)=w1905) -> (element=w1901:T41, timed out?=w1897:bool, error out=w1904:errorcluster)  [unwired: 1 out]
        n898 = case shown="True" w1897 {
          tunnel: w1901 -> [w1911 _]
          tunnel: [w1910 CLIENT_REF_CHG_sequence_state."ping" ("state")] -> w1900
          tunnel: [w1909 _] -> w1899
          frame False {
            n899 = Unbundle By Name(w1911) -> ("variable"=w1909:variant, "state"=w1910:T9)
          }
          frame True {
          }
        }
        n900 = call "CLIENT_REF_CHG_check_for_error.vi"("CLIENT_REF_CHG_sequence_state_in"=w1900, "error_in"=w1904) -> ("CLIENT_REF_CHG_sequence_state_out"=w1907:T9, "error_out"=w1908:errorcluster)  [unwired: 8 in]
      }
      frame "reference_changed" {
        n901 = TCP Write(connection ID=w1915, data in="reference_changed", error in (no error)=w1917, 9:2000 ("timeout ms (25000)")) -> (error out=w1916:errorcluster)  [unwired: 2 out]
        n902 = call "CLIENT_REF_CHG_check_for_error.vi"("CLIENT_REF_CHG_sequence_state_in"=CLIENT_REF_CHG_sequence_state."get_next_state" ("SCANNER_loop_state_in"), "error_in"=w1916) -> ("CLIENT_REF_CHG_sequence_state_out"=w1919:T9, "error_out"=w1920:errorcluster)  [unwired: 8 in]
      }
      frame "ping" {
        n903 = TCP Write(connection ID=w1923, data in="ping", error in (no error)=w1925, 9:2000 ("timeout ms (25000)")) -> (error out=w1924:errorcluster)  [unwired: 2 out]
        n904 = call "CLIENT_REF_CHG_check_for_error.vi"("CLIENT_REF_CHG_sequence_state_in"=CLIENT_REF_CHG_sequence_state."get_next_state" ("SCANNER_loop_state_in"), "error_in"=w1924) -> ("CLIENT_REF_CHG_sequence_state_out"=w1927:T9, "error_out"=w1928:errorcluster)  [unwired: 8 in]
      }
      frame "error" {
        n905 = Unbundle By Name(w1943) -> ("queue_refnums.CLIENT_REF_CHG_queue"=w1942:refnum<queue>)
        n906 = call-poly "Get Localized Phrase Compact Interface.vi"("Key"="Error in connection to PLC Proxy Application.\nReference change not possible until connection is restored.") -> ("Translated Phrase"=w1929:string)
        n907 = Bundle By Name(cluster=w1930, "source"=w1929) -> (w1938:errorcluster)
        n908 = Unbundle By Name(w1930) -> ("status"=w1931:bool)
        n909 = property on="PLC_PROXY_connection_indicator" class="Bool (strict)"("Val(Sgnl)"=w1931) -> ()  [unwired: 2 in, 2 out]
        n910 = call "FGV_CLIENT_error_buffer.vi"("thread"=thread_name."MAIN", "option"=FGV_CLIENT_error_buffer."display", "error_in"=w1938) -> ("error_out"=w1941:errorcluster)  [unwired: 7 in, 1 out]
        n911 = Preview Queue Element(queue=w1942, timeout in ms (-1)=0, error in (no error)=w1941) -> (element=w1946:T41, error out=w1936:errorcluster)  [unwired: 2 out]
        n912 = Unbundle By Name(w1946) -> ("state"=w1944:T9)
        n913 = TCP Close Connection(connection ID=w1935, error in (no error)=w1936) -> (error out=w1934:errorcluster)  [unwired: 1 in, 1 out]
        n914 = call <vilib>:"Clear Errors.vi"("error in (no error)"=w1934) -> ("error out"=w1933:errorcluster)  [unwired: 5 in, 1 out]
        n915 = case shown="Default" w1944 {
          tunnel: [CLIENT_REF_CHG_sequence_state."initialize" ("state") CLIENT_REF_CHG_sequence_state."stop" ("state")] -> w1940
          frame Default {
          }
          frame "stop" {
          }
        }
        n916 = call "wait_on_initialization.vi"("state"=w1940) -> ()  [unwired: 11 in]
      }
      frame "stop" {
        n917 = call <vilib>:"Clear Errors.vi"("error in (no error)"=w1955) -> ("error out"=w1952:errorcluster)  [unwired: 5 in, 1 out]
        n918 = TCP Close Connection(connection ID=w1951, error in (no error)=w1952) -> (error out=w1950:errorcluster)  [unwired: 1 in, 1 out]
      }
    }
  }
  n919 = while {
    shift-right: [w1965] -> _
    shift-left: SCANNER_sequence_state."initialize" ("SQL_EDITOR_sequence_state") -> [w1968]
    shift-right: [w1966] -> w85
    shift-left: w15 -> [w1967]
    tunnel: w21 -> [w1963]
    shift-right: [w1962] -> _
    shift-left: _ -> [w1961]
    shift-right: [w1959] -> _
    shift-left: FALSE -> [w1960]
    shift-right: [w1957] -> _
    shift-left: "" -> [w1958]
    stop <- w1964 stop-if-true
    # "COGNEX SCANNER"
    n920 = case shown="\"initialize\"" w1968 {
      tunnel: w1967 -> [w1985 w2001 w2031 w2068 w2084 w2094]
      tunnel: [w1988 w1999 w2034 w2069 w2074 w2092] -> w1966
      tunnel: [w1986 w1994 w2032 w2067 w2073 SCANNER_sequence_state."stop" ("state")] -> w1965
      tunnel: [_ _ _ _ _ TRUE] -> w1964
      tunnel: w1963 -> [w1983 w2000 w2024 _ w2077 _]
      tunnel: [w1972 w1990 w2030 w2071 w2085 refnum<visa-resource-name> refnum ("VISA resource name out")] -> w1962
      tunnel: w1961 -> [_ w1990 w2030 w2071 w2085 w2091]
      tunnel: w1960 -> [_ w1998 _ _ _ _]
      tunnel: [FALSE w1998 w2025 FALSE FALSE FALSE] -> w1959
      tunnel: w1958 -> [_ w1996 w2020 _ _ _]
      tunnel: ["" w1996 w2022 "" "" ""] -> w1957
      frame "initialize" {
        n921 = Unbundle By Name(w1983) -> ("main_ini_file.SCANNER Termination char"=w1973:u8, "main_ini_file.SCANNER COM port"=w1982:u16, "main_ini_file.SCANNER Baud rate"=w1978:u32, "main_ini_file.SCANNER Data bits"=w1977:u16, "main_ini_file.SCANNER Pairity"=w1976:enum16{"None", "Odd", "Even", "Mark", "Space"}, "main_ini_file.SCANNER Stop bits"=w1975:u16, "main_ini_file.SCANNER Flow control"=w1974:u16)
        n922 = Number To Decimal String(number=w1982) -> (decimal integer string=w1981:string)  [unwired: 1 in]
        n923 = Concatenate Strings("COM" ("string"), w1981) -> (w1979:string)
        n924 = call-poly "VISA Configure Serial Port"("VISA resource name"=w1979, "timeout (10sec)"=u32 150, "termination char\n(0xA = '\\n' = LF)"=w1973, "baud rate (9600)"=w1978, "data bits (8)"=w1977, "parity (0:none)"=w1976, "error in (no error)"=w1985, "stop bits (10: 1 bit)"=w1975, "flow control (0:none)"=w1974) -> ("VISA resource name out"=w1972:refnum<visa-resource-name>, "error out"=w1984:errorcluster)  [unwired: 1 in, 4 out]
        n925 = call "SCANNER_check_for_error.vi"("SCANNER_loop_state_in"=SCANNER_sequence_state."get_next_state" ("SQL_EDITOR_sequence_state"), "error_in"=w1984) -> ("SCANNER_loop_state_out"=w1986:T18, "error_out"=w1988:errorcluster)  [unwired: 8 in]
      }
      frame "get_next_state" {
        n926 = Unbundle By Name(w2000) -> ("queue_refnums.SCANNER_queue"=w2002:refnum<queue>)
        n927 = case shown="True" w1998 {
          tunnel: [-1 ("timeout in ms (-1)") 0 ("timeout in ms (-1)")] -> w1997
          frame False {
          }
          frame True {
          }
        }
        n928 = Dequeue Element(queue=w2002, timeout in ms (-1)=w1997, error in (no error)=w2001) -> (element=w1989:T42, timed out?=w1991:bool, error out=w1993:errorcluster)  [unwired: 1 out]
        n929 = case shown="False" w1991 {
          tunnel: w1989 -> [w2003 _]
          tunnel: [w2004 SCANNER_sequence_state."read" ("state")] -> w1995
          tunnel: [w2007 w2015] -> w1992
          tunnel: w1993 -> [w2008 w2015]
          tunnel: w1990 -> [w2006 _]
          frame False {
            # "clear buffers\non read start"
            n930 = Unbundle By Name(w2003) -> ("state"=w2005:T18)
            n931 = case shown="\"read\"" w2005 {
              selector: w2005 -> [w2010 w2011]
              tunnel: w2008 -> [w2009 w2014]
              tunnel: [w2009 w2013] -> w2007
              tunnel: w2006 -> [_ w2012]
              tunnel: [w2010 w2011] -> w2004
              frame Default {
              }
              frame "read" {
                n932 = VISA Clear(VISA resource name=w2012, error in (no error)=w2014) -> (error out=w2013:errorcluster)  [unwired: 1 out]
              }
            }
          }
          frame True {
          }
        }
        n933 = call "SCANNER_check_for_error.vi"("SCANNER_loop_state_in"=w1995, "error_in"=w1992) -> ("SCANNER_loop_state_out"=w1994:T18, "error_out"=w1999:errorcluster)  [unwired: 8 in]
      }
      frame "read" {
        # "timeout"
        n934 = VISA Read(VISA resource name=w2030, byte count=u32 9999, error in (no error)=w2031) -> (read buffer=w2023:string, return count=w2026:u32, error out=w2021:errorcluster)  [unwired: 1 out]
        n935 = case shown="No Error" w2021 {
          tunnel: w2026 -> [_ w2058]
          tunnel: [w2043 w2057] -> w2025
          tunnel: w2024 -> [w2042 w2056]
          tunnel: w2023 -> [w2037 w2055]
          tunnel: [w2041 w2054] -> w2022
          tunnel: w2020 -> [w2038 w2053]
          tunnel: TRUE -> [w2040 w2052]
          frame No Error {
            # "no (timeout) error means that termination character was encountered"
            n936 = Concatenate Strings(w2038, w2037) -> (w2036:string)
            n937 = Not Equal?(x=w2036, y="NoRead\r\n" ("x")) -> (x != y?=w2035:bool)
            n938 = case shown="True" w2035 {
              tunnel: [FALSE w2051] -> w2043
              tunnel: w2042 -> [w2048 _]
              tunnel: ["" ""] -> w2041
              tunnel: w2040 -> [_ w2051]
              tunnel: w2036 -> [w2044 _]
              frame True {
                # "read successful - send data and stop reading"
                n939 = call <vilib>:"Trim Whitespace.vi"("string"=w2044) -> ("trimmed string"=w2045:string)  [unwired: 1 in]
                n940 = Unbundle By Name(w2048) -> ("queue_refnums.SCANNER_data"=w2047:refnum<queue>)
                n941 = Lossy Enqueue Element(queue=w2047, element=w2045) -> ()  [unwired: 1 in, 4 out]
              }
              frame False {
                # "read completed, but unsuccessful - clear buffer and start read again"
              }
            }
          }
          frame Error {
            # "(timeout) error and some bytes read means that timeout occured before encountering termination character"
            n942 = case shown="Default" w2058 {
              tunnel: [w2062 w2063] -> w2057
              tunnel: w2056 -> [_ _]
              tunnel: w2055 -> [w2060 _]
              tunnel: [w2059 w2064] -> w2054
              tunnel: w2053 -> [w2061 w2064]
              tunnel: w2052 -> [w2062 w2063]
              frame Default {
                # "if error and some bytes read, append new bytes (probably timeout, if not error case will take care of it)"
                n943 = Concatenate Strings(w2061, w2060) -> (w2059:string)
              }
              frame 0 {
                # "if error and no bytes read, do nothing (probably timeout, if not error case will take care of it)"
                # "if error and no bytes read, do nothing (probably timeout, if not error case takes care of it"
              }
            }
          }
        }
        n944 = call <vilib>:"Clear Errors.vi"("error in (no error)"=w2021, "specific error code to clear (0: all)"=-1073807339) -> ("error out"=w2028:errorcluster)  [unwired: 4 in, 1 out]
        n945 = call "SCANNER_check_for_error.vi"("SCANNER_loop_state_in"=SCANNER_sequence_state."get_next_state" ("state"), "error_in"=w2028) -> ("SCANNER_loop_state_out"=w2032:T18, "error_out"=w2034:errorcluster)  [unwired: 8 in]
      }
      frame "cancel_read" {
        n946 = call "SCANNER_check_for_error.vi"("SCANNER_loop_state_in"=SCANNER_sequence_state."get_next_state", "error_in"=w2068) -> ("SCANNER_loop_state_out"=w2067:T18, "error_out"=w2069:errorcluster)  [unwired: 8 in]
      }
      frame "error" {
        n947 = Unbundle By Name(w2077) -> ("queue_refnums.SCANNER_queue"=w2076:refnum<queue>)
        n948 = call "FGV_CLIENT_error_buffer.vi"("thread"=thread_name."MAIN", "option"=FGV_CLIENT_error_buffer."display", "error_in"=w2084) -> ("error_out"=w2075:errorcluster)  [unwired: 7 in, 1 out]
        n949 = Preview Queue Element(queue=w2076, timeout in ms (-1)=0, error in (no error)=w2075) -> (element=w2080:T42, error out=w2074:errorcluster)  [unwired: 2 out]
        n950 = Unbundle By Name(w2080) -> ("state"=w2078:T18)
        n951 = case shown="Default" w2078 {
          tunnel: [SCANNER_sequence_state."initialize" ("state") SCANNER_sequence_state."stop" ("state")] -> w2073
          frame Default {
          }
          frame "stop" {
          }
        }
        n952 = call "wait_on_initialization.vi"("state"=w2073) -> ()  [unwired: 11 in]
      }
      frame "stop" {
        # "1. takes so long to close it\nmaybe its not needed?\n2. works faster on server and is needed\nerrors after restart if not closed properly"
        n953 = call <vilib>:"Clear Errors.vi"("error in (no error)"=w2094) -> ("error out"=w2093:errorcluster)  [unwired: 5 in, 1 out]
        n954 = VISA Close(VISA resource name=w2091, error in (no error)=w2093) -> (error out=w2092:errorcluster)
      }
    }
  }
  n955 = while {
    tunnel: w21 -> [w2101]
    shift-right: [w2103] -> w145
    shift-left: w15 -> [w2104]
    shift-right: [w2100] -> _
    shift-left: SQL_EDITOR_sequence_state."initialize" ("SQL_EDITOR_sequence_state") -> [w2102]
    shift-right: [w2098] -> _
    shift-left: _ -> [w2097]
    stop <- w2099 stop-if-true
    # "SQL MANUAL EDITORS"
    n956 = case shown="\"REPORT_save_pdf\"" w2102 {
      tunnel: [w2121 w2125 w2133 w2153 w2173 w2191 w2208 w2226 w2259 w2270 w2285 w2302 w2320 w2337 w2355 w2386 w2407 w2420 w2439 w2455 w2504 w2536 w2561 w2576 w2598 w2614 w2630 w2647 w2661 w2690 w2698 w2722 w2754 w2776 w2807 w2835 w2865 w2890 w2922 w2952 w2960 w2977 w2985 w3000 w3006 w3038 w3072 w3085] -> w2103
      tunnel: w2104 -> [w2118 w2130 w2134 w2155 w2175 w2192 w2209 w2227 w2256 w2271 w2287 w2304 w2321 w2338 w2356 w2387 w2404 w2421 w2440 w2456 w2490 w2532 w2558 w2565 w2594 w2600 w2617 w2633 w2654 w2687 w2694 w2716 w2744 w2767 w2782 w2813 w2844 w2870 w2898 w2932 w2956 w2967 w2981 w2990 w3002 w3034 w3076 w3085]
      tunnel: w2101 -> [w2106 w2129 _ w2154 _ _ _ _ w2253 _ w2286 _ _ _ _ _ _ _ _ _ _ w2525 _ _ _ _ _ _ _ _ _ _ _ _ _ _ _ _ _ _ _ _ _ _ _ _ w3068 _]
      tunnel: [w2120 w2124 w2132 w2152 w2172 w2189 w2206 w2223 w2258 w2269 w2284 w2301 w2318 w2335 w2352 w2385 w2406 w2418 w2437 w2452 w2502 w2535 w2560 w2575 w2597 w2613 w2629 w2646 w2660 w2689 w2697 w2721 w2753 w2775 w2806 w2834 w2864 w2889 w2921 w2951 w2959 w2976 w2984 w2999 w3005 w3037 w3064 SQL_EDITOR_sequence_state."stop" ("ST_TCP_sequence_state")] -> w2100
      tunnel: [_ _ _ _ _ _ _ _ _ _ _ _ _ _ _ _ _ _ _ _ _ _ _ _ _ _ _ _ _ _ _ _ _ _ _ _ _ _ _ _ _ _ _ _ _ _ _ TRUE] -> w2099
      tunnel: [_ w2122 _ _ _ _ _ _ _ _ _ _ _ _ _ _ _ _ _ _ _ _ _ _ _ _ _ _ _ _ _ _ _ _ _ _ _ _ _ _ _ _ _ _ _ _ _ _] -> w2098
      tunnel: w2097 -> [_ _ _ _ _ _ _ _ _ _ _ _ _ _ _ _ _ _ _ _ w2491 w2533 _ _ _ _ _ _ _ _ w2695 _ _ _ _ _ _ _ _ _ w2957 _ w2982 _ _ _ _ _]
      frame "initialize" {
        n957 = call "FGV_CLIENT_SQL_connection.vi"("options"=FGV_CLIENT_SQL_connection."connect", "error_in"=w2118) -> ("error_out"=w2110:errorcluster)  [unwired: 5 in, 4 out]
        n958 = Unbundle By Name(w2110) -> ("status"=w2111:bool)
        n959 = To Variant(anything=w2106) -> (Variant=w2116:variant)
        n960 = local write "SQL_connection_indicator"(w2111) -> ()
        n961 = call "FGV_REF_EDITOR_records_display.vi"("options"=FGV_REF_EDITOR_records_display."set_reference_tables_names", "error_in"=w2110, "input"=w2116) -> ("error_out"=w2113:errorcluster)  [unwired: 5 in, 3 out]
        n962 = To Variant(anything=w2106) -> (Variant=w2112:variant)
        n963 = call "FGV_ARCH_EDITOR_records_display.vi"("options"=FGV_ARCH_EDITOR_records_display."set_arch_cfg_tables_names", "error_in"=w2113, "input"=w2112) -> ("error_out"=w2109:errorcluster)  [unwired: 5 in, 3 out]
        n964 = To Variant(anything=w2106) -> (Variant=w2107:variant)
        n965 = call "FGV_USER_EDITOR_records_display.vi"("options"=FGV_USER_EDITOR_records_display."set_user_edit_tables_names", "error_in"=w2109, "input"=w2107) -> ("error_out"=w2105:errorcluster)  [unwired: 5 in, 3 out]
        n966 = call "SQL_EDITOR_check_for_error.vi"("SQL_EDITOR_loop_state_in"=SQL_EDITOR_sequence_state."get_next_state" ("SQL_EDITOR_sequence_state"), "error_in"=w2105) -> ("SQL_EDITOR_loop_state_out"=w2120:T25, "error_out"=w2121:errorcluster)  [unwired: 8 in]
      }
      frame "get_next_state" {
        n967 = Unbundle By Name(w2129) -> ("queue_refnums.SQL_EDITOR_queue"=w2128:refnum<queue>)
        n968 = Dequeue Element(queue=w2128, error in (no error)=w2130) -> (element=w2127:T32, error out=w2126:errorcluster)  [unwired: 1 in, 2 out]
        n969 = Unbundle By Name(w2127) -> ("variable"=w2122:variant, "state"=w2123:T25)
        n970 = call "SQL_EDITOR_check_for_error.vi"("SQL_EDITOR_loop_state_in"=w2123, "error_in"=w2126) -> ("SQL_EDITOR_loop_state_out"=w2124:T25, "error_out"=w2125:errorcluster)  [unwired: 8 in]
      }
      frame "REF_read_columns" {
        n971 = call "FGV_REF_EDITOR_records_display.vi"("options"=FGV_REF_EDITOR_records_display."get_ref_table_name", "error_in"=w2134) -> ("error_out"=w2147:errorcluster, "string_param_output"=w2149:string)  [unwired: 6 in, 2 out]
        n972 = call "FGV_CLIENT_SQL_connection.vi"("options"=FGV_CLIENT_SQL_connection."read_columns", "error_in"=w2147, "SQL_statement"=w2149) -> ("error_out"=w2139:errorcluster, "SQL_result"=w2140:variant)  [unwired: 4 in, 3 out]
        n973 = Variant To Data(error in=w2139, type=string[] [], Variant=w2140) -> (data=w2142:string[], error out=w2145:errorcluster)
        n974 = To Variant(anything=w2142) -> (Variant=w2143:variant)
        n975 = call "FGV_REF_EDITOR_records_display.vi"("options"=FGV_REF_EDITOR_records_display."set_headers", "error_in"=w2145, "input"=w2143) -> ("error_out"=w2146:errorcluster)  [unwired: 5 in, 3 out]
        n976 = call "FGV_REF_EDITOR_status_display.vi"("options"=FGV_REF_EDITOR_status_display."display", "error_in"=w2146, "display_source"="COLUMN NAMES READ") -> ("error_out"=w2135:errorcluster)  [unwired: 8 in]
        n977 = call "SQL_EDITOR_check_for_error.vi"("SQL_EDITOR_loop_state_in"=SQL_EDITOR_sequence_state."REF_read_stations", "error_in"=w2135) -> ("SQL_EDITOR_loop_state_out"=w2132:T25, "error_out"=w2133:errorcluster)  [unwired: 8 in]
      }
      frame "REF_read_stations" {
        # "to select the same station as\nbefore after refresh"
        # "ensures that NULL value (if exists) is last"
        n978 = Unbundle By Name(w2154) -> ("main_ini_file.Reference table"=w2162:string)
        n979 = Format Into String(format string="select STATION_NMB\nfrom (select distinct STATION_NMB\n      from %s\n     ) tmp\norder by (case when STATION_NMB is NULL then 1 else 0 end), STATION_NMB asc", w2162) -> (resulting string=w2163:string)  [unwired: 2 in, 1 out]
        n980 = call "FGV_CLIENT_SQL_connection.vi"("options"=FGV_CLIENT_SQL_connection."SELECT", "error_in"=w2155, "SQL_statement"=w2163) -> ("error_out"=w2159:errorcluster, "SQL_result"=w2160:variant)  [unwired: 4 in, 3 out]
        n981 = Variant To Data(error in=w2159, type=string[][] [], Variant=w2160) -> (data=w2164:string[][], error out=w2169:errorcluster)
        n982 = Index Array(array=w2164, index (col)=0 ("disabled index (col)")) -> (element=w2166:string[])  [unwired: 1 in]
        n983 = local read "REF_EDIT_station"() -> (w2170:u16)
        n984 = property on="REF_EDIT_station" class="Ring (strict)"("Strings []"=w2166) -> (error out=w2168:errorcluster)  [unwired: 2 in, 1 out]
        n985 = property on="REF_EDIT_station" class="Ring (strict)"(error in=w2168, "Val(Sgnl)"=w2170) -> ()  [unwired: 1 in, 2 out]
        n986 = call "FGV_REF_EDITOR_status_display.vi"("options"=FGV_REF_EDITOR_status_display."display", "error_in"=w2169, "display_source"="STATION NUMBERS READ") -> ("error_out"=w2151:errorcluster)  [unwired: 8 in]
        n987 = call "SQL_EDITOR_check_for_error.vi"("SQL_EDITOR_loop_state_in"=SQL_EDITOR_sequence_state."get_next_state", "error_in"=w2151) -> ("SQL_EDITOR_loop_state_out"=w2152:T25, "error_out"=w2153:errorcluster)  [unwired: 8 in]
      }
      frame "REF_select_station_records" {
        n988 = call "REF_EDITOR_prepare_SELECT_statement.vi"("nmb_of_top_rows (all)"=200, "error_in"=w2175) -> ("error_out"=w2184:errorcluster, "SELECT_statement"=w2186:string)  [unwired: 8 in]
        n989 = call "FGV_CLIENT_SQL_connection.vi"("options"=FGV_CLIENT_SQL_connection."SELECT", "error_in"=w2184, "SQL_statement"=w2186) -> ("error_out"=w2180:errorcluster, "SQL_result"=w2182:variant, "executed_SQL_statement"=w2181:string)  [unwired: 4 in, 2 out]
        n990 = call "FGV_REF_EDITOR_records_display.vi"("options"=FGV_REF_EDITOR_records_display."set_records", "error_in"=w2180, "input"=w2182) -> ("error_out"=w2176:errorcluster)  [unwired: 5 in, 3 out]
        n991 = call "FGV_REF_EDITOR_status_display.vi"("options"=FGV_REF_EDITOR_status_display."display", "error_in"=w2176, "SQL_statement"=w2181, "display_source"="SELECT STATION RECORDS") -> ("error_out"=w2174:errorcluster)  [unwired: 7 in]
        n992 = call "SQL_EDITOR_check_for_error.vi"("SQL_EDITOR_loop_state_in"=SQL_EDITOR_sequence_state."get_next_state", "error_in"=w2174) -> ("SQL_EDITOR_loop_state_out"=w2172:T25, "error_out"=w2173:errorcluster)  [unwired: 8 in]
      }
      frame "REF_insert_record" {
        n993 = local read "REF_EDIT_records"() -> (w2203:i32)
        n994 = property on="REF_EDIT_records" class="MCListbox (strict)"() -> ("ItemNames"=w2202:string[][])  [unwired: 2 in, 2 out]
        n995 = call "REF_EDITOR_prepare_INSERT_statement.vi"("error_in"=w2192, "selected_record"=w2203, "REF_EDIT_records"=w2202) -> ("error_out"=w2200:errorcluster, "INSERT_statement"=w2201:string)  [unwired: 7 in]
        n996 = call "FGV_CLIENT_SQL_connection.vi"("options"=FGV_CLIENT_SQL_connection."INSERT", "error_in"=w2200, "SQL_statement"=w2201) -> ("error_out"=w2197:errorcluster, "SQL_result"=w2187:variant, "executed_SQL_statement"=w2198:string)  [unwired: 4 in, 2 out]
        n997 = call "FGV_REF_EDITOR_records_display.vi"("options"=FGV_REF_EDITOR_records_display."record_inserted?", "error_in"=w2197, "input"=w2187) -> ("error_out"=w2193:errorcluster)  [unwired: 5 in, 3 out]
        n998 = call "FGV_REF_EDITOR_status_display.vi"("options"=FGV_REF_EDITOR_status_display."display", "error_in"=w2193, "SQL_statement"=w2198, "display_source"="INSERT RECORD") -> ("error_out"=w2190:errorcluster)  [unwired: 7 in]
        n999 = call "SQL_EDITOR_check_for_error.vi"("SQL_EDITOR_loop_state_in"=SQL_EDITOR_sequence_state."REF_send_reference_updated_to_PLC", "error_in"=w2190) -> ("SQL_EDITOR_loop_state_out"=w2189:T25, "error_out"=w2191:errorcluster)  [unwired: 8 in]
      }
      frame "REF_update_record" {
        # "TO ENSURE THAT NEW UNIQUE ID IS GENERATED\nUPDATE IS PERFORMED AS\nCOPY TO ARCHIVE - DELETE OLD - INSERT NEW\nTRANSACTION"
        # "whatever happens, \nupdate only one record"
        n1000 = property on="REF_EDIT_records" class="MCListbox (strict)"() -> ("ItemNames"=w2221:string[][])  [unwired: 2 in, 2 out]
        n1001 = local read "REF_EDIT_records"() -> (w2220:i32)
        n1002 = call "REF_EDITOR_prepare_UPDATE_transaction.vi"("nmb_of_top_rows (all)"=1, "error_in"=w2209, "selected_record"=w2220, "REF_EDIT_records"=w2221) -> ("error_out"=w2215:errorcluster, "UPDATE_transaction"=w2219:string[])  [unwired: 6 in]
        n1003 = call "FGV_CLIENT_SQL_connection.vi"("options"=FGV_CLIENT_SQL_connection."TRANSACTION", "error_in"=w2215, "SQL_transaction"=w2219) -> ("error_out"=w2216:errorcluster, "SQL_result"=w2204:variant, "executed_SQL_statement"=w2217:string)  [unwired: 4 in, 2 out]
        n1004 = call "FGV_REF_EDITOR_records_display.vi"("options"=FGV_REF_EDITOR_records_display."record_updated?", "error_in"=w2216, "input"=w2204) -> ("error_out"=w2210:errorcluster)  [unwired: 5 in, 3 out]
        n1005 = call "FGV_REF_EDITOR_status_display.vi"("options"=FGV_REF_EDITOR_status_display."display", "error_in"=w2210, "SQL_statement"=w2217, "display_source"="UPDATE RECORD") -> ("error_out"=w2207:errorcluster)  [unwired: 7 in]
        n1006 = call "SQL_EDITOR_check_for_error.vi"("SQL_EDITOR_loop_state_in"=SQL_EDITOR_sequence_state."REF_send_reference_updated_to_PLC", "error_in"=w2207) -> ("SQL_EDITOR_loop_state_out"=w2206:T25, "error_out"=w2208:errorcluster)  [unwired: 8 in]
      }
      frame "REF_delete_record" {
        n1007 = call "FGV_REF_EDITOR_records_display.vi"("options"=FGV_REF_EDITOR_records_display."get_all_info") -> ("all_info"=w2228:T47)  [unwired: 7 in, 3 out]
        n1008 = local read "REF_EDIT_records"() -> (w2231:i32)
        n1009 = Unbundle By Name(w2228) -> ("REF_record_states"=w2229:T44[])
        n1010 = Index Array(array=w2229, index=w2231) -> (element=w2230:T44)
        n1011 = case shown="Default" w2230 {
          tunnel: w2231 -> [w2237 _]
          tunnel: w2227 -> [w2239 _]
          tunnel: [w2246 w2247] -> w2232
          tunnel: [w2242 ""] -> w2235
          frame "Equal" {
            # "whatever happens, \ndelete only one record"
            n1012 = property on="REF_EDIT_records" class="MCListbox (strict)"() -> ("ItemNames"=w2236:string[][])  [unwired: 2 in, 2 out]
            n1013 = call "REF_EDITOR_prepare_DELETE_transaction.vi"("nmb_of_top_rows (all)"=1, "error_in"=w2239, "selected_record"=w2237, "REF_EDIT_records"=w2236) -> ("error_out"=w2241:errorcluster, "DELETE_transaction"=w2238:string[])  [unwired: 6 in]
            n1014 = call "FGV_CLIENT_SQL_connection.vi"("options"=FGV_CLIENT_SQL_connection."TRANSACTION", "error_in"=w2241, "SQL_transaction"=w2238) -> ("error_out"=w2243:errorcluster, "executed_SQL_statement"=w2242:string)  [unwired: 4 in, 3 out]
            n1015 = call "FGV_REF_EDITOR_records_display.vi"("options"=FGV_REF_EDITOR_records_display."record_deleted?", "error_in"=w2243) -> ("error_out"=w2246:errorcluster)  [unwired: 6 in, 3 out]
          }
          frame Default {
            n1016 = call-poly "Get Localized Phrase Compact Interface.vi"("Key"="Record that is not synchronised with database can not be deleted" ("source")) -> ("Translated Phrase"=w2248:string)
            n1017 = Bundle By Name(cluster=errorcluster {"status"=FALSE, "code"=501, "source"=""} ("error out"), "source"=w2248) -> (w2247:errorcluster)
          }
        }
        n1018 = call "FGV_REF_EDITOR_status_display.vi"("options"=FGV_REF_EDITOR_status_display."display", "error_in"=w2232, "SQL_statement"=w2235, "display_source"="DELETE RECORD") -> ("error_out"=w2225:errorcluster)  [unwired: 7 in]
        n1019 = call "SQL_EDITOR_check_for_error.vi"("SQL_EDITOR_loop_state_in"=SQL_EDITOR_sequence_state."REF_send_reference_updated_to_PLC", "error_in"=w2225) -> ("SQL_EDITOR_loop_state_out"=w2223:T25, "error_out"=w2226:errorcluster)  [unwired: 8 in]
      }
      frame "REF_send_reference_updated_to_PLC" {
        n1020 = Unbundle By Name(w2253) -> ("queue_refnums.CLIENT_REF_CHG_queue"=w2254:refnum<queue>)
        n1021 = Enqueue Element(queue=w2254, element=T41 {"state"=enum."reference_changed", "variable"=variant}, error in (no error)=w2256) -> (error out=w2255:errorcluster)  [unwired: 1 in, 2 out]
        n1022 = call "SQL_EDITOR_check_for_error.vi"("SQL_EDITOR_loop_state_in"=SQL_EDITOR_sequence_state."get_next_state", "error_in"=w2255) -> ("SQL_EDITOR_loop_state_out"=w2258:T25, "error_out"=w2259:errorcluster)  [unwired: 8 in]
      }
      frame "ARCH_read_columns" {
        n1023 = call "FGV_ARCH_EDITOR_records_display.vi"("options"=FGV_ARCH_EDITOR_records_display."get_arch_cfg_table_name", "error_in"=w2271) -> ("error_out"=w2277:errorcluster, "string_param_output"=w2278:string)  [unwired: 6 in, 2 out]
        n1024 = call "FGV_CLIENT_SQL_connection.vi"("options"=FGV_CLIENT_SQL_connection."read_columns", "error_in"=w2277, "SQL_statement"=w2278) -> ("error_out"=w2273:errorcluster, "SQL_result"=w2274:variant)  [unwired: 4 in, 3 out]
        n1025 = Variant To Data(error in=w2273, type=string[] [], Variant=w2274) -> (data=w2276:string[], error out=w2266:errorcluster)
        n1026 = To Variant(anything=w2276) -> (Variant=w2264:variant)
        n1027 = call "FGV_ARCH_EDITOR_records_display.vi"("options"=FGV_ARCH_EDITOR_records_display."set_headers", "error_in"=w2266, "input"=w2264) -> ("error_out"=w2262:errorcluster)  [unwired: 5 in, 3 out]
        n1028 = call "FGV_ARCH_EDITOR_status_display.vi"("options"=FGV_ARCH_EDITOR_status_display."clear", "error_in"=w2262, "display_source"="COLUMN NAMES READ") -> ("error_out"=w2261:errorcluster)  [unwired: 8 in]
        n1029 = call "SQL_EDITOR_check_for_error.vi"("SQL_EDITOR_loop_state_in"=SQL_EDITOR_sequence_state."ARCH_read_stations", "error_in"=w2261) -> ("SQL_EDITOR_loop_state_out"=w2269:T25, "error_out"=w2270:errorcluster)  [unwired: 8 in]
      }
      frame "ARCH_read_stations" {
        # "to select the same station as\nbefore after refresh"
        # "so complicated, but ensures that NULL value (if exists) is last"
        n1030 = Unbundle By Name(w2286) -> ("main_ini_file.Archivisation CFG table"=w2292:string)
        n1031 = Format Into String(format string="select STATION_NMB\nfrom (select distinct STATION_NMB\n      from %s\n     ) tmp\norder by (case when STATION_NMB is NULL then 1 else 0 end), STATION_NMB asc", w2292) -> (resulting string=w2293:string)  [unwired: 2 in, 1 out]
        n1032 = call "FGV_CLIENT_SQL_connection.vi"("options"=FGV_CLIENT_SQL_connection."SELECT", "error_in"=w2287, "SQL_statement"=w2293) -> ("error_out"=w2289:errorcluster, "SQL_result"=w2290:variant)  [unwired: 4 in, 3 out]
        n1033 = Variant To Data(error in=w2289, type=string[][] [], Variant=w2290) -> (data=w2294:string[][], error out=w2280:errorcluster)
        n1034 = Index Array(array=w2294, index (col)=0 ("disabled index (col)")) -> (element=w2296:string[])  [unwired: 1 in]
        n1035 = local read "ARCH_EDIT_station"() -> (w2299:u16)
        n1036 = property on="ARCH_EDIT_station" class="Ring (strict)"("Strings []"=w2296) -> (error out=w2298:errorcluster)  [unwired: 2 in, 1 out]
        n1037 = property on="ARCH_EDIT_station" class="Ring (strict)"(error in=w2298, "Val(Sgnl)"=w2299) -> ()  [unwired: 1 in, 2 out]
        n1038 = call "FGV_ARCH_EDITOR_status_display.vi"("options"=FGV_ARCH_EDITOR_status_display."clear", "error_in"=w2280, "display_source"="STATION NUMBERS READ") -> ("error_out"=w2281:errorcluster)  [unwired: 8 in]
        n1039 = call "SQL_EDITOR_check_for_error.vi"("SQL_EDITOR_loop_state_in"=SQL_EDITOR_sequence_state."get_next_state", "error_in"=w2281) -> ("SQL_EDITOR_loop_state_out"=w2284:T25, "error_out"=w2285:errorcluster)  [unwired: 8 in]
      }
      frame "ARCH_select_station_records" {
        n1040 = call "ARCH_EDITOR_prepare_SELECT_statement.vi"("nmb_of_top_rows (all)"=200, "error_in"=w2304) -> ("error_out"=w2313:errorcluster, "SELECT_statement"=w2315:string)  [unwired: 8 in]
        n1041 = call "FGV_CLIENT_SQL_connection.vi"("options"=FGV_CLIENT_SQL_connection."SELECT", "error_in"=w2313, "SQL_statement"=w2315) -> ("error_out"=w2309:errorcluster, "SQL_result"=w2311:variant, "executed_SQL_statement"=w2310:string)  [unwired: 4 in, 2 out]
        n1042 = call "FGV_ARCH_EDITOR_records_display.vi"("options"=FGV_ARCH_EDITOR_records_display."set_records", "error_in"=w2309, "input"=w2311) -> ("error_out"=w2305:errorcluster)  [unwired: 5 in, 3 out]
        n1043 = call "FGV_ARCH_EDITOR_status_display.vi"("options"=FGV_ARCH_EDITOR_status_display."display", "error_in"=w2305, "SQL_statement"=w2310, "display_source"="SELECT STATION RECORDS") -> ("error_out"=w2303:errorcluster)  [unwired: 7 in]
        n1044 = call "SQL_EDITOR_check_for_error.vi"("SQL_EDITOR_loop_state_in"=SQL_EDITOR_sequence_state."get_next_state", "error_in"=w2303) -> ("SQL_EDITOR_loop_state_out"=w2301:T25, "error_out"=w2302:errorcluster)  [unwired: 8 in]
      }
      frame "ARCH_insert_record" {
        n1045 = local read "ARCH_EDIT_records"() -> (w2332:i32)
        n1046 = property on="ARCH_EDIT_records" class="MCListbox (strict)"() -> ("ItemNames"=w2331:string[][])  [unwired: 2 in, 2 out]
        n1047 = call "ARCH_EDITOR_prepare_INSERT_statement.vi"("error_in"=w2321, "selected_record"=w2332, "ARCH_EDIT_records"=w2331) -> ("error_out"=w2329:errorcluster, "INSERT_statement"=w2330:string)  [unwired: 7 in]
        n1048 = call "FGV_CLIENT_SQL_connection.vi"("options"=FGV_CLIENT_SQL_connection."INSERT", "error_in"=w2329, "SQL_statement"=w2330) -> ("error_out"=w2326:errorcluster, "SQL_result"=w2316:variant, "executed_SQL_statement"=w2327:string)  [unwired: 4 in, 2 out]
        n1049 = call "FGV_ARCH_EDITOR_records_display.vi"("options"=FGV_ARCH_EDITOR_records_display."record_inserted?", "error_in"=w2326, "input"=w2316) -> ("error_out"=w2322:errorcluster)  [unwired: 5 in, 3 out]
        n1050 = call "FGV_ARCH_EDITOR_status_display.vi"("options"=FGV_ARCH_EDITOR_status_display."display", "error_in"=w2322, "SQL_statement"=w2327, "display_source"="INSERT RECORD") -> ("error_out"=w2319:errorcluster)  [unwired: 7 in]
        n1051 = call "SQL_EDITOR_check_for_error.vi"("SQL_EDITOR_loop_state_in"=SQL_EDITOR_sequence_state."get_next_state", "error_in"=w2319) -> ("SQL_EDITOR_loop_state_out"=w2318:T25, "error_out"=w2320:errorcluster)  [unwired: 8 in]
      }
      frame "ARCH_update_record" {
        # "TO ENSURE THAT NEW UNIQUE ID IS GENERATED\nUPDATE IS PERFORMED AS\nCOPY TO ARCHIVE - DELETE OLD - INSERT NEW\nTRANSACTION"
        # "whatever happens, \nupdate only one record"
        n1052 = property on="ARCH_EDIT_records" class="MCListbox (strict)"() -> ("ItemNames"=w2350:string[][])  [unwired: 2 in, 2 out]
        n1053 = local read "ARCH_EDIT_records"() -> (w2349:i32)
        n1054 = call "ARCH_EDITOR_prepare_UPDATE_transaction.vi"("nmb_of_top_rows (all)"=1, "error_in"=w2338, "selected_record"=w2349, "ARCH_EDIT_records"=w2350) -> ("error_out"=w2344:errorcluster, "UPDATE_transaction"=w2348:string[])  [unwired: 6 in]
        n1055 = call "FGV_CLIENT_SQL_connection.vi"("options"=FGV_CLIENT_SQL_connection."TRANSACTION", "error_in"=w2344, "SQL_transaction"=w2348) -> ("error_out"=w2345:errorcluster, "SQL_result"=w2333:variant, "executed_SQL_statement"=w2346:string)  [unwired: 4 in, 2 out]
        n1056 = call "FGV_ARCH_EDITOR_records_display.vi"("options"=FGV_ARCH_EDITOR_records_display."record_updated?", "error_in"=w2345, "input"=w2333) -> ("error_out"=w2339:errorcluster)  [unwired: 5 in, 3 out]
        n1057 = call "FGV_ARCH_EDITOR_status_display.vi"("options"=FGV_ARCH_EDITOR_status_display."display", "error_in"=w2339, "SQL_statement"=w2346, "display_source"="UPDATE RECORD") -> ("error_out"=w2336:errorcluster)  [unwired: 7 in]
        n1058 = call "SQL_EDITOR_check_for_error.vi"("SQL_EDITOR_loop_state_in"=SQL_EDITOR_sequence_state."get_next_state", "error_in"=w2336) -> ("SQL_EDITOR_loop_state_out"=w2335:T25, "error_out"=w2337:errorcluster)  [unwired: 8 in]
      }
      frame "ARCH_delete_record" {
        n1059 = call "FGV_ARCH_EDITOR_records_display.vi"("options"=FGV_ARCH_EDITOR_records_display."get_all_info") -> ("all_info"=w2357:T43)  [unwired: 7 in, 3 out]
        n1060 = local read "ARCH_EDIT_records"() -> (w2360:i32)
        n1061 = Unbundle By Name(w2357) -> ("ARCH_record_states"=w2358:T44[])
        n1062 = Index Array(array=w2358, index=w2360) -> (element=w2359:T44)
        n1063 = case shown="Default" w2359 {
          tunnel: w2360 -> [w2366 _]
          tunnel: w2356 -> [w2368 _]
          tunnel: [w2375 w2376] -> w2361
          tunnel: [w2371 ""] -> w2364
          frame "Equal" {
            # "whatever happens, \ndelete only one record"
            n1064 = property on="ARCH_EDIT_records" class="MCListbox (strict)"() -> ("ItemNames"=w2365:string[][])  [unwired: 2 in, 2 out]
            n1065 = call "ARCH_EDITOR_prepare_DELETE_transaction.vi"("nmb_of_top_rows (all)"=1, "error_in"=w2368, "selected_record"=w2366, "ARCH_EDIT_records"=w2365) -> ("error_out"=w2370:errorcluster, "DELETE_transaction"=w2367:string[])  [unwired: 6 in]
            n1066 = call "FGV_CLIENT_SQL_connection.vi"("options"=FGV_CLIENT_SQL_connection."TRANSACTION", "error_in"=w2370, "SQL_transaction"=w2367) -> ("error_out"=w2372:errorcluster, "executed_SQL_statement"=w2371:string)  [unwired: 4 in, 3 out]
            n1067 = call "FGV_ARCH_EDITOR_records_display.vi"("options"=FGV_ARCH_EDITOR_records_display."record_deleted?", "error_in"=w2372) -> ("error_out"=w2375:errorcluster)  [unwired: 6 in, 3 out]
          }
          frame Default {
            n1068 = call-poly "Get Localized Phrase Compact Interface.vi"("Key"="Record that is not synchronised with database can not be deleted" ("source")) -> ("Translated Phrase"=w2377:string)
            n1069 = Bundle By Name(cluster=errorcluster {"status"=FALSE, "code"=501, "source"=""} ("error out"), "source"=w2377) -> (w2376:errorcluster)
          }
        }
        n1070 = call "FGV_ARCH_EDITOR_status_display.vi"("options"=FGV_ARCH_EDITOR_status_display."display", "error_in"=w2361, "SQL_statement"=w2364, "display_source"="DELETE RECORD") -> ("error_out"=w2354:errorcluster)  [unwired: 7 in]
        n1071 = call "SQL_EDITOR_check_for_error.vi"("SQL_EDITOR_loop_state_in"=SQL_EDITOR_sequence_state."get_next_state", "error_in"=w2354) -> ("SQL_EDITOR_loop_state_out"=w2352:T25, "error_out"=w2355:errorcluster)  [unwired: 8 in]
      }
      frame "USER_read_columns" {
        n1072 = call "FGV_USER_EDITOR_records_display.vi"("options"=FGV_USER_EDITOR_records_display."get_user_edit_table_name", "error_in"=w2387) -> ("error_out"=w2398:errorcluster, "string_param_output"=w2399:string)  [unwired: 6 in, 2 out]
        n1073 = call "FGV_CLIENT_SQL_connection.vi"("options"=FGV_CLIENT_SQL_connection."read_columns", "error_in"=w2398, "SQL_statement"=w2399) -> ("error_out"=w2391:errorcluster, "SQL_result"=w2392:variant)  [unwired: 4 in, 3 out]
        n1074 = Variant To Data(error in=w2391, type=string[] [], Variant=w2392) -> (data=w2394:string[], error out=w2396:errorcluster)
        n1075 = To Variant(anything=w2394) -> (Variant=w2395:variant)
        n1076 = call "FGV_USER_EDITOR_records_display.vi"("options"=FGV_USER_EDITOR_records_display."set_headers", "error_in"=w2396, "input"=w2395) -> ("error_out"=w2397:errorcluster)  [unwired: 5 in, 3 out]
        n1077 = call "FGV_USER_EDITOR_status_display.vi"("options"=FGV_USER_EDITOR_status_display."display", "error_in"=w2397, "display_source"="COLUMN NAMES READ") -> ("error_out"=w2388:errorcluster)  [unwired: 8 in]
        n1078 = call "SQL_EDITOR_check_for_error.vi"("SQL_EDITOR_loop_state_in"=SQL_EDITOR_sequence_state."USER_select_records", "error_in"=w2388) -> ("SQL_EDITOR_loop_state_out"=w2385:T25, "error_out"=w2386:errorcluster)  [unwired: 8 in]
      }
      frame "USER_select_records" {
        n1079 = call "USER_EDITOR_prepare_SELECT_statement.vi"("error_in"=w2404) -> ("error_out"=w2403:errorcluster, "SELECT_statement"=w2402:string)  [unwired: 9 in]
        n1080 = call "FGV_CLIENT_SQL_connection.vi"("options"=FGV_CLIENT_SQL_connection."SELECT", "error_in"=w2403, "SQL_statement"=w2402) -> ("error_out"=w2412:errorcluster, "SQL_result"=w2414:variant, "executed_SQL_statement"=w2413:string)  [unwired: 4 in, 2 out]
        n1081 = call "FGV_USER_EDITOR_records_display.vi"("options"=FGV_USER_EDITOR_records_display."set_records", "error_in"=w2412, "input"=w2414) -> ("error_out"=w2409:errorcluster)  [unwired: 5 in, 3 out]
        n1082 = call "FGV_USER_EDITOR_status_display.vi"("options"=FGV_USER_EDITOR_status_display."display", "error_in"=w2409, "SQL_statement"=w2413, "display_source"="SELECT STATION RECORDS") -> ("error_out"=w2408:errorcluster)  [unwired: 7 in]
        n1083 = call "SQL_EDITOR_check_for_error.vi"("SQL_EDITOR_loop_state_in"=SQL_EDITOR_sequence_state."get_next_state", "error_in"=w2408) -> ("SQL_EDITOR_loop_state_out"=w2406:T25, "error_out"=w2407:errorcluster)  [unwired: 8 in]
      }
      frame "USER_insert_record" {
        n1084 = local read "USER_EDIT_records"() -> (w2416:i32)
        n1085 = property on="USER_EDIT_records" class="MCListbox (strict)"() -> ("ItemNames"=w2431:string[][])  [unwired: 2 in, 2 out]
        n1086 = call "USER_EDITOR_prepare_INSERT_statement.vi"("error_in"=w2421, "selected_record"=w2416, "USER_EDIT_records"=w2431) -> ("error_out"=w2429:errorcluster, "INSERT_statement"=w2430:string)  [unwired: 7 in]
        n1087 = call "FGV_CLIENT_SQL_connection.vi"("options"=FGV_CLIENT_SQL_connection."INSERT", "error_in"=w2429, "SQL_statement"=w2430) -> ("error_out"=w2426:errorcluster, "SQL_result"=w2415:variant, "executed_SQL_statement"=w2427:string)  [unwired: 4 in, 2 out]
        n1088 = call "FGV_USER_EDITOR_records_display.vi"("options"=FGV_USER_EDITOR_records_display."record_inserted?", "error_in"=w2426, "input"=w2415) -> ("error_out"=w2422:errorcluster)  [unwired: 5 in, 3 out]
        n1089 = call "FGV_USER_EDITOR_status_display.vi"("options"=FGV_USER_EDITOR_status_display."display", "error_in"=w2422, "SQL_statement"=w2427, "display_source"="INSERT RECORD") -> ("error_out"=w2419:errorcluster)  [unwired: 7 in]
        n1090 = call "SQL_EDITOR_check_for_error.vi"("SQL_EDITOR_loop_state_in"=SQL_EDITOR_sequence_state."get_next_state", "error_in"=w2419) -> ("SQL_EDITOR_loop_state_out"=w2418:T25, "error_out"=w2420:errorcluster)  [unwired: 8 in]
      }
      frame "USER_update_record" {
        # "TO ENSURE THAT NEW UNIQUE ID IS GENERATED\nUPDATE IS PERFORMED AS\nCOPY TO ARCHIVE - DELETE OLD - INSERT NEW\nTRANSACTION"
        # "whatever happens, \nupdate only one record"
        n1091 = property on="USER_EDIT_records" class="MCListbox (strict)"() -> ("ItemNames"=w2449:string[][])  [unwired: 2 in, 2 out]
        n1092 = local read "USER_EDIT_records"() -> (w2448:i32)
        n1093 = call "USER_EDITOR_prepare_UPDATE_transaction.vi"("nmb_of_top_rows (all)"=1, "error_in"=w2440, "selected_record"=w2448, "USER_EDIT_records"=w2449) -> ("error_out"=w2444:errorcluster, "UPDATE_transaction"=w2447:string[])  [unwired: 6 in]
        n1094 = call "FGV_CLIENT_SQL_connection.vi"("options"=FGV_CLIENT_SQL_connection."TRANSACTION", "error_in"=w2444, "SQL_transaction"=w2447) -> ("error_out"=w2434:errorcluster, "SQL_result"=w2432:variant, "executed_SQL_statement"=w2445:string)  [unwired: 4 in, 2 out]
        n1095 = call "FGV_USER_EDITOR_records_display.vi"("options"=FGV_USER_EDITOR_records_display."record_updated?", "error_in"=w2434, "input"=w2432) -> ("error_out"=w2433:errorcluster)  [unwired: 5 in, 3 out]
        n1096 = call "FGV_USER_EDITOR_status_display.vi"("options"=FGV_USER_EDITOR_status_display."display", "error_in"=w2433, "SQL_statement"=w2445, "display_source"="UPDATE RECORD") -> ("error_out"=w2438:errorcluster)  [unwired: 7 in]
        n1097 = call "SQL_EDITOR_check_for_error.vi"("SQL_EDITOR_loop_state_in"=SQL_EDITOR_sequence_state."get_next_state", "error_in"=w2438) -> ("SQL_EDITOR_loop_state_out"=w2437:T25, "error_out"=w2439:errorcluster)  [unwired: 8 in]
      }
      frame "USER_delete_record" {
        n1098 = call "FGV_USER_EDITOR_records_display.vi"("options"=FGV_USER_EDITOR_records_display."get_all_info") -> ("all_info"=w2450:T49)  [unwired: 7 in, 3 out]
        n1099 = local read "USER_EDIT_records"() -> (w2459:i32)
        n1100 = Unbundle By Name(w2450) -> ("USER_record_states"=w2457:T44[])
        n1101 = Index Array(array=w2457, index=w2459) -> (element=w2458:T44)
        n1102 = case shown="Default" w2458 {
          tunnel: w2459 -> [w2465 _]
          tunnel: w2456 -> [w2467 _]
          tunnel: [w2474 w2475] -> w2460
          tunnel: [w2470 ""] -> w2463
          frame "Equal" {
            # "whatever happens, \ndelete only one record"
            n1103 = property on="USER_EDIT_records" class="MCListbox (strict)"() -> ("ItemNames"=w2464:string[][])  [unwired: 2 in, 2 out]
            n1104 = call "USER_EDITOR_prepare_DELETE_transaction.vi"("nmb_of_top_rows (all)"=1, "error_in"=w2467, "selected_record"=w2465, "USER_EDIT_records"=w2464) -> ("error_out"=w2469:errorcluster, "DELETE_transaction"=w2466:string[])  [unwired: 6 in]
            n1105 = call "FGV_CLIENT_SQL_connection.vi"("options"=FGV_CLIENT_SQL_connection."TRANSACTION", "error_in"=w2469, "SQL_transaction"=w2466) -> ("error_out"=w2471:errorcluster, "executed_SQL_statement"=w2470:string)  [unwired: 4 in, 3 out]
            n1106 = call "FGV_USER_EDITOR_records_display.vi"("options"=FGV_USER_EDITOR_records_display."record_deleted?", "error_in"=w2471) -> ("error_out"=w2474:errorcluster)  [unwired: 6 in, 3 out]
          }
          frame Default {
            n1107 = call-poly "Get Localized Phrase Compact Interface.vi"("Key"="Record that is not synchronised with database can not be deleted" ("source")) -> ("Translated Phrase"=w2476:string)
            n1108 = Bundle By Name(cluster=errorcluster {"status"=FALSE, "code"=501, "source"=""} ("error out"), "source"=w2476) -> (w2475:errorcluster)
          }
        }
        n1109 = call "FGV_USER_EDITOR_status_display.vi"("options"=FGV_USER_EDITOR_status_display."display", "error_in"=w2460, "SQL_statement"=w2463, "display_source"="DELETE RECORD") -> ("error_out"=w2454:errorcluster)  [unwired: 7 in]
        n1110 = call "SQL_EDITOR_check_for_error.vi"("SQL_EDITOR_loop_state_in"=SQL_EDITOR_sequence_state."get_next_state", "error_in"=w2454) -> ("SQL_EDITOR_loop_state_out"=w2452:T25, "error_out"=w2455:errorcluster)  [unwired: 8 in]
      }
      frame "USER_update_barcode" {
        n1111 = Variant To Data(error in=w2490, type="", Variant=w2491) -> (data=w2482:string, error out=w2486:errorcluster)
        n1112 = call "Hash String with SHA-256.vi"("error_n"=w2486, "string"=w2482) -> ("error_out"=w2485:errorcluster, "hash"=w2481:string)  [unwired: 8 in]
        n1113 = call "FGV_USER_EDITOR_records_display.vi"("options"=FGV_USER_EDITOR_records_display."get_all_info") -> ("all_info"=w2499:T49)  [unwired: 7 in, 3 out]
        n1114 = local read "USER_EDIT_records"() -> (w2492:i32)
        n1115 = property on="USER_EDIT_records" class="MCListbox (strict)"(error in=w2485) -> ("ItemNames"=w2493:string[][])  [unwired: 1 in, 2 out]
        n1116 = Unbundle By Name(w2499) -> ("size.SQL_rows"=w2494:i32)
        n1117 = Replace Array Subset(array=w2493, new element=w2481, index (row)=w2492, index (col)=23 ("disabled index (col)")) -> (w2487:string[][])
        n1118 = Less?(x=w2494, y=w2492) -> (x < y?=w2495:bool)
        n1119 = property on="USER_EDIT_records" class="MCListbox (strict)"("ItemNames"=w2487) -> (error out=w2496:errorcluster)  [unwired: 2 in, 1 out]
        n1120 = call-poly "Get Localized Phrase Compact Interface.vi"("Key"="UPDATE BARCODE - NEW CODE: %s - HASH: %s" ("display_source")) -> ("Translated Phrase"=w2480:string)
        n1121 = case shown="True" w2495 {
          tunnel: w2492 -> [w2509 w2514]
          tunnel: [w2506 w2511] -> w2497
          tunnel: w2496 -> [w2505 w2510]
          frame False {
            n1122 = To Variant(anything=w2509) -> (Variant=w2508:variant)
            n1123 = call "FGV_USER_EDITOR_records_display.vi"("options"=FGV_USER_EDITOR_records_display."record_edited?", "error_in"=w2505, "input"=w2508) -> ("error_out"=w2506:errorcluster)  [unwired: 5 in, 3 out]
          }
          frame True {
            n1124 = To Variant(anything=w2514) -> (Variant=w2513:variant)
            n1125 = call "FGV_USER_EDITOR_records_display.vi"("options"=FGV_USER_EDITOR_records_display."record_added?", "error_in"=w2510, "input"=w2513) -> ("error_out"=w2511:errorcluster)  [unwired: 5 in, 3 out]
          }
        }
        n1126 = Format Into String(format string=w2480, w2482, w2481) -> (resulting string=w2483:string)  [unwired: 2 in, 1 out]
        n1127 = call "FGV_USER_EDITOR_status_display.vi"("options"=FGV_USER_EDITOR_status_display."display", "error_in"=w2497, "display_source"=w2483) -> ("error_out"=w2503:errorcluster)  [unwired: 8 in]
        n1128 = call "SQL_EDITOR_check_for_error.vi"("SQL_EDITOR_loop_state_in"=SQL_EDITOR_sequence_state."get_next_state", "error_in"=w2503) -> ("SQL_EDITOR_loop_state_out"=w2502:T25, "error_out"=w2504:errorcluster)  [unwired: 8 in]
      }
      frame "USER_login" {
        n1129 = Variant To Data(error in=w2532, type="", Variant=w2533) -> (data=w2516:string, error out=w2530:errorcluster)
        n1130 = Unbundle By Name(w2525) -> ("main_ini_file.User table"=w2524:string)
        n1131 = call "Hash String with SHA-256.vi"("error_n"=w2530, "string"=w2516) -> ("error_out"=w2526:errorcluster, "hash"=w2515:string)  [unwired: 8 in]
        n1132 = Format Into String(format string="select USER_NAME, PROXY_APP\nfrom %s\nwhere BARCODE_HASH = '%s'\norder by ID desc", w2524, w2515) -> (resulting string=w2529:string)  [unwired: 2 in, 1 out]
        n1133 = call "FGV_CLIENT_SQL_connection.vi"("options"=FGV_CLIENT_SQL_connection."SELECT", "error_in"=w2526, "SQL_statement"=w2529) -> ("error_out"=w2528:errorcluster, "SQL_result"=w2521:variant)  [unwired: 4 in, 3 out]
        n1134 = Variant To Data(error in=w2528, type=string[][] [], Variant=w2521) -> (data=w2518:string[][], error out=w2519:errorcluster)
        n1135 = Empty Array?(array=w2518) -> (empty?=w2517:bool)
        n1136 = case shown="True" w2517 {
          tunnel: [w2545 w2553] -> w2522
          tunnel: w2519 -> [w2542 w2554]
          tunnel: w2518 -> [w2537 _]
          tunnel: w2516 -> [_ w2549]
          tunnel: w2515 -> [_ w2548]
          frame False {
            w2544 = 0 ("index (row)")
            n1137 = Index Array(array=w2537, index (row) #1=w2544, index (col) #1=w2544, index (row) #2=w2544, index (col) #2=1 ("disabled index (col)")) -> (element #1=w2541:string, element #2=w2539:string)
            n1138 = Decimal String To Number(string=w2539) -> (number=w2538:i32)  [unwired: 2 in, 1 out]
            n1139 = call "FGV_login.vi"("options"=FGV_login."login", "error_in"=w2542, "access_level_in"=w2538, "username_in"=w2541) -> ("error_out"=w2545:errorcluster)  [unwired: 5 in, 2 out]
          }
          frame True {
            n1140 = call-poly "Get Localized Phrase Compact Interface.vi"("Key"="Scanned card not in database!\nCard: %s\nHash: %s" ("Message")) -> ("Translated Phrase"=w2546:string)
            n1141 = Format Into String(format string=w2546, w2549, w2548) -> (resulting string=w2547:string)  [unwired: 2 in, 1 out]
            n1142 = call "message_popup.vi"("Warning(T)/Info(F)"=TRUE, "error_in"=w2554, "Message"=w2547, "Title"="Login", "Button Label"="OK") -> ("error_out"=w2553:errorcluster)  [unwired: 6 in]
          }
        }
        n1143 = call "SQL_EDITOR_check_for_error.vi"("SQL_EDITOR_loop_state_in"=SQL_EDITOR_sequence_state."get_next_state", "error_in"=w2522) -> ("SQL_EDITOR_loop_state_out"=w2535:T25, "error_out"=w2536:errorcluster)  [unwired: 8 in]
      }
      frame "USER_logout" {
        n1144 = call "FGV_login.vi"("options"=FGV_login."logout", "error_in"=w2558) -> ("error_out"=w2557:errorcluster)  [unwired: 7 in, 2 out]
        n1145 = call "SQL_EDITOR_check_for_error.vi"("SQL_EDITOR_loop_state_in"=SQL_EDITOR_sequence_state."get_next_state", "error_in"=w2557) -> ("SQL_EDITOR_loop_state_out"=w2560:T25, "error_out"=w2561:errorcluster)  [unwired: 8 in]
      }
      frame "SQL_read_tables" {
        n1146 = call "FGV_CLIENT_SQL_connection.vi"("options"=FGV_CLIENT_SQL_connection."read_tables", "error_in"=w2565) -> ("error_out"=w2569:errorcluster, "SQL_result"=w2567:variant)  [unwired: 5 in, 3 out]
        n1147 = Variant To Data(error in=w2569, type=string[] [], Variant=w2567) -> (data=w2564:string[], error out=w2568:errorcluster)
        n1148 = property on="SQL_EDIT_table" class="Ring (strict)"("Strings []"=w2564) -> (error out=w2563:errorcluster)  [unwired: 2 in, 1 out]
        n1149 = local read "SQL_EDIT_table"() -> (w2562:u16)
        n1150 = property on="SQL_EDIT_table" class="Ring (strict)"(error in=w2563, "Val(Sgnl)"=w2562) -> ()  [unwired: 1 in, 2 out]
        n1151 = call "FGV_SQL_EDITOR_status_display.vi"("options"=FGV_SQL_EDITOR_status_display."display", "error_in"=w2568, "display_source"="TABLES READ") -> ("error_out"=w2574:errorcluster)  [unwired: 8 in]
        n1152 = call "SQL_EDITOR_check_for_error.vi"("SQL_EDITOR_loop_state_in"=SQL_EDITOR_sequence_state."get_next_state" ("SQL_EDITOR_sequence_state"), "error_in"=w2574) -> ("SQL_EDITOR_loop_state_out"=w2575:T25, "error_out"=w2576:errorcluster)  [unwired: 8 in]
      }
      frame "SQL_read_columns" {
        n1153 = call "FGV_SQL_EDITOR_records_display.vi"("options"=FGV_SQL_EDITOR_records_display."get_table_name", "error_in"=w2594) -> ("error_out"=w2584:errorcluster, "string_param_output"=w2583:string)  [unwired: 6 in, 2 out]
        n1154 = call "FGV_CLIENT_SQL_connection.vi"("options"=FGV_CLIENT_SQL_connection."read_columns", "error_in"=w2584, "SQL_statement"=w2583) -> ("error_out"=w2581:errorcluster, "SQL_result"=w2579:variant)  [unwired: 4 in, 3 out]
        n1155 = Variant To Data(error in=w2581, type=string[] [], Variant=w2579) -> (data=w2577:string[], error out=w2580:errorcluster)
        n1156 = To Variant(anything=w2577) -> (Variant=w2591:variant)
        n1157 = property on="SQL_EDIT_column" class="Ring (strict)"("Strings []"=w2577) -> (error out=w2595:errorcluster)  [unwired: 2 in, 1 out]
        n1158 = property on="SQL_EDIT_order_by" class="Ring (strict)"("Strings []"=w2577) -> (error out=w2586:errorcluster)  [unwired: 2 in, 1 out]
        n1159 = call "FGV_SQL_EDITOR_records_display.vi"("options"=FGV_SQL_EDITOR_records_display."set_headers", "input"=w2591) -> ()  [unwired: 6 in, 4 out]
        n1160 = property on="SQL_EDIT_column" class="Ring (strict)"(error in=w2595, "Val(Sgnl)"=u16 0) -> ()  [unwired: 1 in, 2 out]
        n1161 = property on="SQL_EDIT_order_by" class="Ring (strict)"(error in=w2586, "Val(Sgnl)"=u16 0) -> ()  [unwired: 1 in, 2 out]
        n1162 = call "FGV_SQL_EDITOR_status_display.vi"("options"=FGV_SQL_EDITOR_status_display."display", "error_in"=w2580, "display_source"="COLUMN NAMES READ") -> ("error_out"=w2590:errorcluster)  [unwired: 8 in]
        n1163 = call "SQL_EDITOR_check_for_error.vi"("SQL_EDITOR_loop_state_in"=SQL_EDITOR_sequence_state."get_next_state" ("SQL_EDITOR_sequence_state"), "error_in"=w2590) -> ("SQL_EDITOR_loop_state_out"=w2597:T25, "error_out"=w2598:errorcluster)  [unwired: 8 in]
      }
      frame "SQL_select_records" {
        n1164 = call "SQL_EDITOR_prepare_SELECT_statement.vi"("nmb_of_top_rows (all)"=500, "error_in"=w2600) -> ("error_out"=w2601:errorcluster, "SELECT_statement"=w2602:string)  [unwired: 8 in]
        n1165 = call "FGV_CLIENT_SQL_connection.vi"("options"=FGV_CLIENT_SQL_connection."SELECT", "error_in"=w2601, "SQL_statement"=w2602) -> ("error_out"=w2605:errorcluster, "SQL_result"=w2603:variant, "executed_SQL_statement"=w2604:string)  [unwired: 4 in, 2 out]
        n1166 = call "FGV_SQL_EDITOR_records_display.vi"("options"=FGV_SQL_EDITOR_records_display."set_records", "error_in"=w2605, "input"=w2603) -> ("error_out"=w2611:errorcluster)  [unwired: 5 in, 3 out]
        n1167 = call "FGV_SQL_EDITOR_status_display.vi"("options"=FGV_SQL_EDITOR_status_display."display", "error_in"=w2611, "SQL_statement"=w2604, "display_source"="SELECT RECORDS") -> ("error_out"=w2610:errorcluster)  [unwired: 7 in]
        n1168 = call "SQL_EDITOR_check_for_error.vi"("SQL_EDITOR_loop_state_in"=SQL_EDITOR_sequence_state."get_next_state" ("MAIN_SQL_loop_state_in"), "error_in"=w2610) -> ("SQL_EDITOR_loop_state_out"=w2613:T25, "error_out"=w2614:errorcluster)  [unwired: 8 in]
      }
      frame "SQL_insert_record" {
        n1169 = local read "SQL_EDIT_records"() -> (w2615:i32)
        n1170 = property on="SQL_EDIT_records" class="MCListbox (strict)"() -> ("ItemNames"=w2616:string[][])  [unwired: 2 in, 2 out]
        n1171 = call "SQL_EDITOR_prepare_INSERT_statement.vi"("error_in"=w2617, "selected_record"=w2615, "SQL_EDIT_records"=w2616) -> ("error_out"=w2619:errorcluster, "INSERT_statement"=w2618:string)  [unwired: 7 in]
        n1172 = call "FGV_CLIENT_SQL_connection.vi"("options"=FGV_CLIENT_SQL_connection."INSERT", "error_in"=w2619, "SQL_statement"=w2618) -> ("error_out"=w2622:errorcluster, "executed_SQL_statement"=w2621:string)  [unwired: 4 in, 3 out]
        n1173 = call "FGV_SQL_EDITOR_records_display.vi"("options"=FGV_SQL_EDITOR_records_display."record_inserted?", "error_in"=w2622) -> ("error_out"=w2628:errorcluster)  [unwired: 6 in, 3 out]
        n1174 = call "FGV_SQL_EDITOR_status_display.vi"("options"=FGV_SQL_EDITOR_status_display."display", "error_in"=w2628, "SQL_statement"=w2621, "display_source"="INSERT RECORD") -> ("error_out"=w2627:errorcluster)  [unwired: 7 in]
        n1175 = call "SQL_EDITOR_check_for_error.vi"("SQL_EDITOR_loop_state_in"=SQL_EDITOR_sequence_state."get_next_state" ("MAIN_SQL_loop_state_in"), "error_in"=w2627) -> ("SQL_EDITOR_loop_state_out"=w2629:T25, "error_out"=w2630:errorcluster)  [unwired: 8 in]
      }
      frame "SQL_update_record" {
        # "whatever happens, \nupdate only one record"
        n1176 = property on="SQL_EDIT_records" class="MCListbox (strict)"() -> ("ItemNames"=w2631:string[][])  [unwired: 2 in, 2 out]
        n1177 = local read "SQL_EDIT_records"() -> (w2632:i32)
        n1178 = call "SQL_EDITOR_prepare_UPDATE_statement.vi"("nmb_of_top_rows (all)"=1, "error_in"=w2633, "selected_record"=w2632, "REF_EDIT_records"=w2631) -> ("error_out"=w2638:errorcluster, "UPDATE_statement"=w2634:string)  [unwired: 6 in]
        n1179 = call "FGV_CLIENT_SQL_connection.vi"("options"=FGV_CLIENT_SQL_connection."UPDATE", "error_in"=w2638, "SQL_statement"=w2634) -> ("error_out"=w2637:errorcluster, "executed_SQL_statement"=w2636:string)  [unwired: 4 in, 3 out]
        n1180 = call "FGV_SQL_EDITOR_records_display.vi"("options"=FGV_SQL_EDITOR_records_display."record_updated?", "error_in"=w2637) -> ("error_out"=w2645:errorcluster)  [unwired: 6 in, 3 out]
        n1181 = call "FGV_SQL_EDITOR_status_display.vi"("options"=FGV_SQL_EDITOR_status_display."display", "error_in"=w2645, "SQL_statement"=w2636, "display_source"="UPDATE RECORD") -> ("error_out"=w2644:errorcluster)  [unwired: 7 in]
        n1182 = call "SQL_EDITOR_check_for_error.vi"("SQL_EDITOR_loop_state_in"=SQL_EDITOR_sequence_state."get_next_state" ("MAIN_SQL_loop_state_in"), "error_in"=w2644) -> ("SQL_EDITOR_loop_state_out"=w2646:T25, "error_out"=w2647:errorcluster)  [unwired: 8 in]
      }
      frame "SQL_delete_record" {
        n1183 = call "FGV_SQL_EDITOR_records_display.vi"("options"=FGV_SQL_EDITOR_records_display."get_all_info") -> ("all_info"=w2658:T48)  [unwired: 7 in, 3 out]
        n1184 = Unbundle By Name(w2658) -> ("SQL_record_states"=w2657:T44[])
        n1185 = local read "SQL_EDIT_records"() -> (w2655:i32)
        n1186 = Index Array(array=w2657, index=w2655) -> (element=w2656:T44)
        n1187 = case shown="Default" w2656 {
          tunnel: w2655 -> [w2663 _]
          tunnel: w2654 -> [w2664 _]
          tunnel: [w2672 w2675] -> w2653
          tunnel: [w2669 ""] -> w2649
          frame "Equal" {
            # "whatever happens, \ndelete only one record"
            n1188 = property on="SQL_EDIT_records" class="MCListbox (strict)"() -> ("ItemNames"=w2662:string[][])  [unwired: 2 in, 2 out]
            n1189 = call "SQL_EDITOR_prepare_DELETE_statement.vi"("nmb_of_top_rows (all)"=1, "error_in"=w2664, "selected_record"=w2663, "SQL_EDIT_records"=w2662) -> ("error_out"=w2665:errorcluster, "DELETE_statement"=w2668:string)  [unwired: 6 in]
            n1190 = call "FGV_CLIENT_SQL_connection.vi"("options"=FGV_CLIENT_SQL_connection."DELETE", "error_in"=w2665, "SQL_statement"=w2668) -> ("error_out"=w2670:errorcluster, "executed_SQL_statement"=w2669:string)  [unwired: 4 in, 3 out]
            n1191 = call "FGV_SQL_EDITOR_records_display.vi"("options"=FGV_SQL_EDITOR_records_display."record_deleted?", "error_in"=w2670) -> ("error_out"=w2672:errorcluster)  [unwired: 6 in, 3 out]
          }
          frame Default {
            n1192 = call-poly "Get Localized Phrase Compact Interface.vi"("Key"="Record that is not synchronised with database can not be deleted" ("source")) -> ("Translated Phrase"=w2673:string)
            n1193 = Bundle By Name(cluster=errorcluster {"status"=FALSE, "code"=501, "source"=""} ("error out"), "source"=w2673) -> (w2675:errorcluster)
          }
        }
        n1194 = call "FGV_SQL_EDITOR_status_display.vi"("options"=FGV_SQL_EDITOR_status_display."display", "error_in"=w2653, "SQL_statement"=w2649, "display_source"="DELETE RECORD") -> ("error_out"=w2652:errorcluster)  [unwired: 7 in]
        n1195 = call "SQL_EDITOR_check_for_error.vi"("SQL_EDITOR_loop_state_in"=SQL_EDITOR_sequence_state."get_next_state" ("MAIN_SQL_loop_state_in"), "error_in"=w2652) -> ("SQL_EDITOR_loop_state_out"=w2660:T25, "error_out"=w2661:errorcluster)  [unwired: 8 in]
      }
      frame "SQL_TEXT_execute" {
        n1196 = call "FGV_CLIENT_SQL_connection.vi"("options"=FGV_CLIENT_SQL_connection."EXEC + headers", "error_in"=w2687, "SQL_statement"="SQL_TEXT_input") -> ("error_out"=w2680:errorcluster, "SQL_result"=w2678:variant, "executed_SQL_statement"=w2682:string)  [unwired: 4 in, 2 out]
        n1197 = call "FGV_SQL_TEXT_records_display.vi"("options"=FGV_SQL_TEXT_records_display."set", "error_in"=w2680, "input"=w2678) -> ("error_out"=w2679:errorcluster)  [unwired: 8 in]
        n1198 = call "FGV_SQL_TEXT_status_display.vi"("options"=FGV_SQL_TEXT_status_display."display", "error_in"=w2679, "SQL_statement"=w2682) -> ("error_out"=w2684:errorcluster)  [unwired: 8 in]
        n1199 = call "SQL_EDITOR_check_for_error.vi"("SQL_EDITOR_loop_state_in"=SQL_EDITOR_sequence_state."get_next_state" ("MAIN_SQL_loop_state_in"), "error_in"=w2684) -> ("SQL_EDITOR_loop_state_out"=w2689:T25, "error_out"=w2690:errorcluster)  [unwired: 8 in]
      }
      frame "REPORT_GEAR_scan_barcode" {
        n1200 = Variant To Data(error in=w2694, type="", Variant=w2695) -> (data=w2692:string, error out=w2691:errorcluster)
        n1201 = local write "REPORT_GEAR_serial"(w2692) -> ()
        n1202 = call "SQL_EDITOR_check_for_error.vi"("SQL_EDITOR_loop_state_in"=SQL_EDITOR_sequence_state."get_next_state", "error_in"=w2691) -> ("SQL_EDITOR_loop_state_out"=w2697:T25, "error_out"=w2698:errorcluster)  [unwired: 8 in]
      }
      frame "REPORT_GEAR_get" {
        n1203 = local read "REPORT_GEAR_serial"() -> (w2699:string)
        n1204 = To Variant(anything=w2699) -> (Variant=w2701:variant)
        n1205 = Format Into String(format string="select top 1 PRODUCTION_PARTS.ID, PRODUCTION_PARTS.CREATION_TIME, PRODUCTION_PARTS.LAST_STATION_NMB, PRODUCTION_PARTS.LAST_STATUS, PRODUCTION_PINIONS.PINION_SERIAL, DOCK_AUDIT_BATCHES.BATCH_CODE, PRODUCTION_PARTS.PINION_ID, PRODUCTION_PARTS.BATCH_ID\nfrom PRODUCTION_PARTS \nleft join PRODUCTION_PINIONS on PRODUCTION_PARTS.PINION_ID = PRODUCTION_PINIONS.ID\nleft join DOCK_AUDIT_BATCHES on PRODUCTION_PARTS.BATCH_ID = DOCK_AUDIT_BATCHES.ID\nwhere PART_SERIAL = '%s'", w2699) -> (resulting string=w2712:string)  [unwired: 2 in, 1 out]
        n1206 = call "FGV_REPORTS_records_display.vi"("options"=FGV_REPORTS_records_display."GEAR_set_serial", "input"=w2701) -> ()  [unwired: 8 in, 2 out]
        n1207 = call "FGV_CLIENT_SQL_connection.vi"("options"=FGV_CLIENT_SQL_connection."SELECT", "error_in"=w2716, "SQL_statement"=w2712) -> ("error_out"=w2714:errorcluster, "SQL_result"=w2709:variant, "executed_SQL_statement"=w2700:string)  [unwired: 4 in, 2 out]
        n1208 = local write "REPORT_GEAR_serial_display"(w2699) -> ()
        n1209 = call "FGV_REPORTS_records_display.vi"("options"=FGV_REPORTS_records_display."GEAR_set_header", "error_in"=w2714, "input"=w2709) -> ("error_out"=w2711:errorcluster)  [unwired: 7 in, 1 out]
        n1210 = call "REPORT_GEAR_get_operations_and_results.vi"("executed_SQL_statement_in"=w2700, "error_in"=w2711, "SQL_result"=w2709) -> ("error_out"=w2706:errorcluster, "executed_SQL_statement_out"=w2710:string)  [unwired: 7 in]
        n1211 = local read "REPORT_GEAR_station"() -> (w2703:T3)
        n1212 = To Variant(anything=w2703) -> (Variant=w2704:variant)
        n1213 = call "FGV_REPORTS_records_display.vi"("options"=FGV_REPORTS_records_display."GEAR_display", "error_in"=w2706, "input"=w2704) -> ("error_out"=w2705:errorcluster)  [unwired: 7 in, 1 out]
        n1214 = call "FGV_REPORTS_status_display.vi"("options"=FGV_REPORTS_status_display."display", "error_in"=w2705, "SQL_statement"=w2710, "display_source"="GEAR REPORT") -> ("error_out"=w2717:errorcluster)  [unwired: 7 in]
        n1215 = call "SQL_EDITOR_check_for_error.vi"("SQL_EDITOR_loop_state_in"=SQL_EDITOR_sequence_state."get_next_state", "error_in"=w2717) -> ("SQL_EDITOR_loop_state_out"=w2721:T25, "error_out"=w2722:errorcluster)  [unwired: 8 in]
      }
      frame "REPORT_DATES_get" {
        w2723 = "%Y-%m-%d %H:%M:%S" ("time format string (%c)")
        w2740 = "%H:%M:%S" ("time format string (%c)")
        n1216 = local read "REPORT_DATES_time_start"() -> (w2742:timestamp)
        n1217 = local read "REPORT_DATES_time_end"() -> (w2741:timestamp)
        n1218 = local read "REPORT_DATES_start"() -> (w2743:timestamp)
        n1219 = local read "REPORT_DATES_end"() -> (w2748:timestamp)
        n1220 = Format Date/Time String(time format string (%c)=w2723, seconds (now)=w2743) -> (date/time string=w2727:string)  [unwired: 1 in]
        n1221 = Format Date/Time String(time format string (%c)=w2723, seconds (now)=w2748) -> (date/time string=w2726:string)  [unwired: 1 in]
        n1222 = Format Date/Time String(time format string (%c)=w2740, seconds (now)=w2742) -> (date/time string=w2725:string)  [unwired: 1 in]
        n1223 = Format Date/Time String(time format string (%c)=w2740, seconds (now)=w2741) -> (date/time string=w2724:string)  [unwired: 1 in]
        n1224 = Format Into String(format string="SELECT PRODUCTION_PARTS.ID, PRODUCTION_PARTS.CREATION_TIME, PRODUCTION_PARTS.PART_SERIAL, PRODUCTION_PARTS.LAST_STATION_NMB, PRODUCTION_PARTS.LAST_STATUS, PRODUCTION_PINIONS.PINION_SERIAL, DOCK_AUDIT_BATCHES.BATCH_CODE\nFROM PRODUCTION_PARTS\nleft join PRODUCTION_PINIONS on PRODUCTION_PARTS.PINION_ID = PRODUCTION_PINIONS.ID\nleft join DOCK_AUDIT_BATCHES on PRODUCTION_PARTS.BATCH_ID = DOCK_AUDIT_BATCHES.ID\nWHERE (PRODUCTION_PARTS.CREATION_TIME BETWEEN '%s' AND '%s') \nAND (CAST(PRODUCTION_PARTS.CREATION_TIME as time) BETWEEN '%s' AND '%s')\nORDER BY CREATION_TIME", w2727, w2726, w2725, w2724) -> (resulting string=w2745:string)  [unwired: 2 in, 1 out]
        n1225 = Build Array(w2727, w2726, w2725, w2724) -> (w2728:string[])
        n1226 = To Variant(anything=w2728) -> (Variant=w2729:variant)
        n1227 = call "FGV_REPORTS_records_display.vi"("options"=FGV_REPORTS_records_display."DATES_set_dates", "input"=w2729) -> ()  [unwired: 8 in, 2 out]
        n1228 = call "FGV_CLIENT_SQL_connection.vi"("options"=FGV_CLIENT_SQL_connection."SELECT", "error_in"=w2744, "SQL_statement"=w2745) -> ("error_out"=w2738:errorcluster, "SQL_result"=w2736:variant, "executed_SQL_statement"=w2739:string)  [unwired: 4 in, 2 out]
        n1229 = call "FGV_REPORTS_records_display.vi"("options"=FGV_REPORTS_records_display."DATES_set_gears", "error_in"=w2738, "input"=w2736) -> ("error_out"=w2734:errorcluster)  [unwired: 7 in, 1 out]
        n1230 = local read "REPORT_DATES_order_selection"() -> (w2731:enum32{"old_to_new", "new_to_old"})
        n1231 = To Variant(anything=w2731) -> (Variant=w2732:variant)
        n1232 = call "FGV_REPORTS_records_display.vi"("options"=FGV_REPORTS_records_display."DATES_display", "error_in"=w2734, "input"=w2732) -> ("error_out"=w2733:errorcluster)  [unwired: 7 in, 1 out]
        n1233 = call "FGV_REPORTS_status_display.vi"("options"=FGV_REPORTS_status_display."display", "error_in"=w2733, "SQL_statement"=w2739, "display_source"="DATES REPORT") -> ("error_out"=w2750:errorcluster)  [unwired: 7 in]
        n1234 = call "SQL_EDITOR_check_for_error.vi"("SQL_EDITOR_loop_state_in"=SQL_EDITOR_sequence_state."get_next_state", "error_in"=w2750) -> ("SQL_EDITOR_loop_state_out"=w2753:T25, "error_out"=w2754:errorcluster)  [unwired: 8 in]
      }
      frame "REPORT_PBATCH_get" {
        n1235 = local read "REPORT_PBATCH_batch_no"() -> (w2760:string)
        n1236 = To Variant(anything=w2760) -> (Variant=w2761:variant)
        n1237 = Format Into String(format string="with cte_operation_id_station as(\nSELECT DISTINCT PART_ID, STATION_NMB FROM PRODUCTION_PARTS_OPERATIONS\nWHERE ID IN\n(SELECT DISTINCT OPERATION_ID FROM PRODUCTION_BATCHES_OPERATIONS\nWHERE BATCH_ID IN\n(SELECT DISTINCT ID FROM PRODUCTION_BATCHES\nWHERE BATCH_NUMBER = '%s')))\n\nSELECT PRODUCTION_PARTS.ID, PRODUCTION_PARTS.CREATION_TIME, PRODUCTION_PARTS.PART_SERIAL, PRODUCTION_PARTS.LAST_STATION_NMB, PRODUCTION_PARTS.LAST_STATUS, PRODUCTION_PINIONS.PINION_SERIAL, DOCK_AUDIT_BATCHES.BATCH_CODE, cte_operation_id_station.STATION_NMB\nFROM cte_operation_id_station, PRODUCTION_PARTS \nleft join PRODUCTION_PINIONS on PRODUCTION_PARTS.PINION_ID = PRODUCTION_PINIONS.ID\nleft join DOCK_AUDIT_BATCHES on PRODUCTION_PARTS.BATCH_ID = DOCK_AUDIT_BATCHES.ID\nWHERE (PRODUCTION_PARTS.ID IN (cte_operation_id_station.PART_ID) AND cte_operation_id_station.STATION_NMB <> 30) OR (PRODUCTION_PARTS.PINION_ID IN (cte_operation_id_station.PART_ID) AND cte_operation_id_station.STATION_NMB = 30)\nORDER BY CREATION_TIME", w2760) -> (resulting string=w2768:string)  [unwired: 2 in, 1 out]
        n1238 = call "FGV_REPORTS_records_display.vi"("options"=FGV_REPORTS_records_display."PBATCH_set_batch_no", "input"=w2761) -> ()  [unwired: 8 in, 2 out]
        n1239 = call "FGV_CLIENT_SQL_connection.vi"("options"=FGV_CLIENT_SQL_connection."EXEC", "error_in"=w2767, "SQL_statement"=w2768) -> ("error_out"=w2764:errorcluster, "SQL_result"=w2763:variant, "executed_SQL_statement"=w2766:string)  [unwired: 4 in, 2 out]
        n1240 = call "FGV_REPORTS_records_display.vi"("options"=FGV_REPORTS_records_display."PBATCH_set_gears", "error_in"=w2764, "input"=w2763) -> ("error_out"=w2758:errorcluster)  [unwired: 7 in, 1 out]
        n1241 = local read "REPORT_PBATCH_order_selection"() -> (w2755:enum32{"old_to_new", "new_to_old"})
        n1242 = To Variant(anything=w2755) -> (Variant=w2756:variant)
        n1243 = call "FGV_REPORTS_records_display.vi"("options"=FGV_REPORTS_records_display."PBATCH_display", "error_in"=w2758, "input"=w2756) -> ("error_out"=w2757:errorcluster)  [unwired: 7 in, 1 out]
        n1244 = call "FGV_REPORTS_status_display.vi"("options"=FGV_REPORTS_status_display."display", "error_in"=w2757, "SQL_statement"=w2766, "display_source"="PRODUCTION BATCH REPORT") -> ("error_out"=w2772:errorcluster)  [unwired: 7 in]
        n1245 = call "SQL_EDITOR_check_for_error.vi"("SQL_EDITOR_loop_state_in"=SQL_EDITOR_sequence_state."get_next_state", "error_in"=w2772) -> ("SQL_EDITOR_loop_state_out"=w2775:T25, "error_out"=w2776:errorcluster)  [unwired: 8 in]
      }
      frame "REPORT_OPRTN_get" {
        w2786 = "%Y-%m-%d %H:%M:%S" ("time format string (%c)")
        w2797 = "%H:%M:%S" ("time format string (%c)")
        n1246 = local read "REPORT_OPRTN_time_start"() -> (w2799:timestamp)
        n1247 = local read "REPORT_OPRTN_time_end"() -> (w2798:timestamp)
        n1248 = local read "REPORT_OPRTN_operation"() -> (w2783:T5)
        n1249 = local read "REPORT_OPRTN_start"() -> (w2800:timestamp)
        n1250 = local read "REPORT_OPRTN_end"() -> (w2801:timestamp)
        n1251 = Format Date/Time String(time format string (%c)=w2786, seconds (now)=w2800) -> (date/time string=w2790:string)  [unwired: 1 in]
        n1252 = Format Date/Time String(time format string (%c)=w2786, seconds (now)=w2801) -> (date/time string=w2789:string)  [unwired: 1 in]
        n1253 = Format Date/Time String(time format string (%c)=w2797, seconds (now)=w2799) -> (date/time string=w2788:string)  [unwired: 1 in]
        n1254 = Format Date/Time String(time format string (%c)=w2797, seconds (now)=w2798) -> (date/time string=w2787:string)  [unwired: 1 in]
        n1255 = Build Array(w2790, w2789, w2788, w2787) -> (w2778:string[])
        n1256 = Number To Decimal String(number=w2783) -> (decimal integer string=w2777:string)  [unwired: 1 in]
        n1257 = call "REPORT_OPRTN_get_data_from_SQL.vi"("operation"=w2777, "error_in"=w2782, "dates_array"=w2778) -> ("error_out"=w2781:errorcluster, "SQL_result"=w2779:variant, "executed_SQL_statement"=w2780:string)  [unwired: 6 in]
        n1258 = To Variant(anything=w2777) -> (Variant=w2784:variant)
        n1259 = call "FGV_REPORTS_records_display.vi"("options"=FGV_REPORTS_records_display."OPRTN_set_OP", "input"=w2784) -> ()  [unwired: 8 in, 2 out]
        n1260 = call "FGV_REPORTS_records_display.vi"("options"=FGV_REPORTS_records_display."OPRTN_set_gears", "error_in"=w2781, "input"=w2779) -> ("error_out"=w2794:errorcluster)  [unwired: 7 in, 1 out]
        n1261 = local read "REPORT_OPRTN_order_selection"() -> (w2791:enum32{"old_to_new", "new_to_old"})
        n1262 = To Variant(anything=w2791) -> (Variant=w2792:variant)
        n1263 = call "FGV_REPORTS_records_display.vi"("options"=FGV_REPORTS_records_display."OPRTN_display", "error_in"=w2794, "input"=w2792) -> ("error_out"=w2793:errorcluster)  [unwired: 7 in, 1 out]
        n1264 = call "FGV_REPORTS_status_display.vi"("options"=FGV_REPORTS_status_display."display", "error_in"=w2793, "SQL_statement"=w2780, "display_source"="OPERATION REPORT") -> ("error_out"=w2803:errorcluster)  [unwired: 7 in]
        n1265 = call "SQL_EDITOR_check_for_error.vi"("SQL_EDITOR_loop_state_in"=SQL_EDITOR_sequence_state."get_next_state", "error_in"=w2803) -> ("SQL_EDITOR_loop_state_out"=w2806:T25, "error_out"=w2807:errorcluster)  [unwired: 8 in]
      }
      frame "REPORT_CFG_get" {
        w2814 = "%Y-%m-%d %H:%M:%S" ("time format string (%c)")
        w2825 = "%H:%M:%S" ("time format string (%c)")
        n1266 = local read "REPORT_CFG_time_start"() -> (w2827:timestamp)
        n1267 = local read "REPORT_CFG_time_end"() -> (w2826:timestamp)
        n1268 = local read "REPORT_CFG_type"() -> (w2808:T6)
        n1269 = local read "REPORT_CFG_start"() -> (w2828:timestamp)
        n1270 = local read "REPORT_CFG_end"() -> (w2829:timestamp)
        n1271 = Format Date/Time String(time format string (%c)=w2814, seconds (now)=w2828) -> (date/time string=w2818:string)  [unwired: 1 in]
        n1272 = Format Date/Time String(time format string (%c)=w2814, seconds (now)=w2829) -> (date/time string=w2817:string)  [unwired: 1 in]
        n1273 = Format Date/Time String(time format string (%c)=w2825, seconds (now)=w2827) -> (date/time string=w2816:string)  [unwired: 1 in]
        n1274 = Format Date/Time String(time format string (%c)=w2825, seconds (now)=w2826) -> (date/time string=w2815:string)  [unwired: 1 in]
        n1275 = Build Array(w2818, w2817, w2816, w2815) -> (w2809:string[])
        n1276 = call "REPORT_CFG_get_data_from_SQL.vi"("type"=w2808, "error_in"=w2813, "dates_array"=w2809) -> ("error_out"=w2812:errorcluster, "SQL_result"=w2810:variant, "executed_SQL_statement"=w2811:string)  [unwired: 6 in]
        n1277 = call "FGV_REPORTS_records_display.vi"("options"=FGV_REPORTS_records_display."CFG_set_records", "error_in"=w2812, "input"=w2810) -> ("error_out"=w2822:errorcluster)  [unwired: 7 in, 1 out]
        n1278 = local read "REPORT_CFG_order_selection"() -> (w2819:enum32{"old_to_new", "new_to_old"})
        n1279 = To Variant(anything=w2819) -> (Variant=w2820:variant)
        n1280 = call "FGV_REPORTS_records_display.vi"("options"=FGV_REPORTS_records_display."CFG_display", "error_in"=w2822, "input"=w2820) -> ("error_out"=w2821:errorcluster)  [unwired: 7 in, 1 out]
        n1281 = call "FGV_REPORTS_status_display.vi"("options"=FGV_REPORTS_status_display."display", "error_in"=w2821, "SQL_statement"=w2811, "display_source"="CONFIG HISTORY REPORT") -> ("error_out"=w2831:errorcluster)  [unwired: 7 in]
        n1282 = call "SQL_EDITOR_check_for_error.vi"("SQL_EDITOR_loop_state_in"=SQL_EDITOR_sequence_state."get_next_state", "error_in"=w2831) -> ("SQL_EDITOR_loop_state_out"=w2834:T25, "error_out"=w2835:errorcluster)  [unwired: 8 in]
      }
      frame "REPORT_AUDIT_get" {
        w2845 = "%Y-%m-%d %H:%M:%S" ("time format string (%c)")
        w2855 = "%H:%M:%S" ("time format string (%c)")
        n1283 = local read "REPORT_AUDIT_time_start"() -> (w2857:timestamp)
        n1284 = local read "REPORT_AUDIT_time_end"() -> (w2856:timestamp)
        n1285 = local read "REPORT_AUDIT_start"() -> (w2858:timestamp)
        n1286 = local read "REPORT_AUDIT_end"() -> (w2859:timestamp)
        n1287 = Format Date/Time String(time format string (%c)=w2845, seconds (now)=w2858) -> (date/time string=w2849:string)  [unwired: 1 in]
        n1288 = Format Date/Time String(time format string (%c)=w2845, seconds (now)=w2859) -> (date/time string=w2848:string)  [unwired: 1 in]
        n1289 = Format Date/Time String(time format string (%c)=w2855, seconds (now)=w2857) -> (date/time string=w2847:string)  [unwired: 1 in]
        n1290 = Format Date/Time String(time format string (%c)=w2855, seconds (now)=w2856) -> (date/time string=w2846:string)  [unwired: 1 in]
        n1291 = Build Array(w2849, w2848, w2847, w2846) -> (w2841:string[])
        n1292 = call "REPORT_AUDIT_get_data_from_SQL.vi"("error_in"=w2844, "dates_array"=w2841) -> ("error_out"=w2843:errorcluster, "SQL_result"=w2842:variant, "executed_SQL_statement"=w2838:string)  [unwired: 7 in]
        n1293 = call "FGV_REPORTS_records_display.vi"("options"=FGV_REPORTS_records_display."AUDIT_set_records", "error_in"=w2843, "input"=w2842) -> ("error_out"=w2839:errorcluster, "output"=w2840:variant)  [unwired: 7 in]
        n1294 = call "REPORT_AUDIT_get_data_results.vi"("executed_SQL_statement_in"=w2838, "error_in"=w2839, "SQL_result"=w2840) -> ("error_out"=w2836:errorcluster, "executed_SQL_statement_out"=w2837:string)  [unwired: 7 in]
        n1295 = local read "REPORT_CFG_order_selection"() -> (w2850:enum32{"old_to_new", "new_to_old"})
        n1296 = To Variant(anything=w2850) -> (Variant=w2851:variant)
        n1297 = call "FGV_REPORTS_records_display.vi"("options"=FGV_REPORTS_records_display."AUDIT_display", "error_in"=w2836, "input"=w2851) -> ("error_out"=w2852:errorcluster)  [unwired: 7 in, 1 out]
        n1298 = call "FGV_REPORTS_status_display.vi"("options"=FGV_REPORTS_status_display."display", "error_in"=w2852, "SQL_statement"=w2837, "display_source"="AUDIT HISTOTY REPORT") -> ("error_out"=w2861:errorcluster)  [unwired: 7 in]
        n1299 = call "SQL_EDITOR_check_for_error.vi"("SQL_EDITOR_loop_state_in"=SQL_EDITOR_sequence_state."get_next_state", "error_in"=w2861) -> ("SQL_EDITOR_loop_state_out"=w2864:T25, "error_out"=w2865:errorcluster)  [unwired: 8 in]
      }
      frame "REPORT_OKNOK_get" {
        w2871 = "%Y-%m-%d %H:%M:%S" ("time format string (%c)")
        w2880 = "%H:%M:%S" ("time format string (%c)")
        n1300 = local read "REPORT_OKNOK_time_start"() -> (w2882:timestamp)
        n1301 = local read "REPORT_OKNOK_time_end"() -> (w2881:timestamp)
        n1302 = local read "REPORT_OKNOK_start"() -> (w2883:timestamp)
        n1303 = local read "REPORT_OKNOK_end"() -> (w2884:timestamp)
        n1304 = Format Date/Time String(time format string (%c)=w2871, seconds (now)=w2883) -> (date/time string=w2875:string)  [unwired: 1 in]
        n1305 = Format Date/Time String(time format string (%c)=w2871, seconds (now)=w2884) -> (date/time string=w2874:string)  [unwired: 1 in]
        n1306 = Format Date/Time String(time format string (%c)=w2880, seconds (now)=w2882) -> (date/time string=w2873:string)  [unwired: 1 in]
        n1307 = Format Date/Time String(time format string (%c)=w2880, seconds (now)=w2881) -> (date/time string=w2872:string)  [unwired: 1 in]
        n1308 = Build Array(w2875, w2874, w2873, w2872) -> (w2866:string[])
        n1309 = call "REPORT_OKNOK_get_data_from_SQL.vi"("error_in"=w2870, "dates_array"=w2866) -> ("error_out"=w2869:errorcluster, "SQL_result"=w2867:variant, "executed_SQL_statement"=w2868:string)  [unwired: 7 in]
        n1310 = call "FGV_REPORTS_records_display.vi"("options"=FGV_REPORTS_records_display."OKNOK_set_records", "error_in"=w2869, "input"=w2867) -> ("error_out"=w2877:errorcluster)  [unwired: 7 in, 1 out]
        n1311 = call "FGV_REPORTS_records_display.vi"("options"=FGV_REPORTS_records_display."OKNOK_display", "error_in"=w2877) -> ("error_out"=w2876:errorcluster)  [unwired: 8 in, 1 out]
        n1312 = call "FGV_REPORTS_status_display.vi"("options"=FGV_REPORTS_status_display."display", "error_in"=w2876, "SQL_statement"=w2868, "display_source"="OK NOK COUNT REPORT") -> ("error_out"=w2886:errorcluster)  [unwired: 7 in]
        n1313 = call "SQL_EDITOR_check_for_error.vi"("SQL_EDITOR_loop_state_in"=SQL_EDITOR_sequence_state."get_next_state", "error_in"=w2886) -> ("SQL_EDITOR_loop_state_out"=w2889:T25, "error_out"=w2890:errorcluster)  [unwired: 8 in]
      }
      frame "REPORT_REWORKS_get" {
        w2901 = "%Y-%m-%d %H:%M:%S" ("time format string (%c)")
        w2912 = "%H:%M:%S" ("time format string (%c)")
        n1314 = local read "REPORT_REWORKS_time_start"() -> (w2914:timestamp)
        n1315 = local read "REPORT_REWORKS_time_end"() -> (w2913:timestamp)
        n1316 = local read "REPORT_REWORKS_start"() -> (w2915:timestamp)
        n1317 = local read "REPORT_REWORKS_end"() -> (w2916:timestamp)
        n1318 = local read "REPORT_REWORKS_from_OP"() -> (w2893:T7)
        n1319 = local read "REPORT_REWORKS_to_OP"() -> (w2892:T7)
        n1320 = Format Date/Time String(time format string (%c)=w2901, seconds (now)=w2915) -> (date/time string=w2905:string)  [unwired: 1 in]
        n1321 = Format Date/Time String(time format string (%c)=w2901, seconds (now)=w2916) -> (date/time string=w2904:string)  [unwired: 1 in]
        n1322 = Format Date/Time String(time format string (%c)=w2912, seconds (now)=w2914) -> (date/time string=w2903:string)  [unwired: 1 in]
        n1323 = Format Date/Time String(time format string (%c)=w2912, seconds (now)=w2913) -> (date/time string=w2902:string)  [unwired: 1 in]
        n1324 = Build Array(w2893, w2892) -> (w2891:T7[])
        n1325 = Build Array(w2905, w2904, w2903, w2902) -> (w2894:string[])
        n1326 = call "REPORT_REWORKS_get_data_from_SQL.vi"("from_OP_to_OP"=w2891, "error_in"=w2898, "dates_array"=w2894) -> ("error_out"=w2897:errorcluster, "SQL_result"=w2895:variant, "executed_SQL_statement"=w2896:string)  [unwired: 6 in]
        n1327 = To Variant(anything=w2891) -> (Variant=w2899:variant)
        n1328 = call "FGV_REPORTS_records_display.vi"("options"=FGV_REPORTS_records_display."REWORKS_set_from_to", "input"=w2899) -> ()  [unwired: 8 in, 2 out]
        n1329 = call "FGV_REPORTS_records_display.vi"("options"=FGV_REPORTS_records_display."REWORKS_set_records", "error_in"=w2897, "input"=w2895) -> ("error_out"=w2909:errorcluster)  [unwired: 7 in, 1 out]
        n1330 = local read "REPORT_REWORKS_order_selection"() -> (w2906:enum32{"old_to_new", "new_to_old"})
        n1331 = To Variant(anything=w2906) -> (Variant=w2907:variant)
        n1332 = call "FGV_REPORTS_records_display.vi"("options"=FGV_REPORTS_records_display."REWORKS_display", "error_in"=w2909, "input"=w2907) -> ("error_out"=w2908:errorcluster)  [unwired: 7 in, 1 out]
        n1333 = call "FGV_REPORTS_status_display.vi"("options"=FGV_REPORTS_status_display."display", "error_in"=w2908, "SQL_statement"=w2896, "display_source"="REWORKS REPORT") -> ("error_out"=w2918:errorcluster)  [unwired: 7 in]
        n1334 = call "SQL_EDITOR_check_for_error.vi"("SQL_EDITOR_loop_state_in"=SQL_EDITOR_sequence_state."get_next_state", "error_in"=w2918) -> ("SQL_EDITOR_loop_state_out"=w2921:T25, "error_out"=w2922:errorcluster)  [unwired: 8 in]
      }
      frame "REPORT_PACE_get" {
        w2933 = "%Y-%m-%d %H:%M:%S" ("time format string (%c)")
        w2942 = "%H:%M:%S" ("time format string (%c)")
        n1335 = local read "REPORT_PACE_time_start"() -> (w2944:timestamp)
        n1336 = local read "REPORT_PACE_time_end"() -> (w2943:timestamp)
        n1337 = local read "REPORT_PACE_high_limit"() -> (w2926:u16)
        n1338 = local read "REPORT_PACE_low_limit"() -> (w2927:u16)
        n1339 = local read "REPORT_PACE_start"() -> (w2945:timestamp)
        n1340 = local read "REPORT_PACE_end"() -> (w2946:timestamp)
        n1341 = Format Date/Time String(time format string (%c)=w2933, seconds (now)=w2945) -> (date/time string=w2937:string)  [unwired: 1 in]
        n1342 = Format Date/Time String(time format string (%c)=w2933, seconds (now)=w2946) -> (date/time string=w2936:string)  [unwired: 1 in]
        n1343 = Format Date/Time String(time format string (%c)=w2942, seconds (now)=w2944) -> (date/time string=w2935:string)  [unwired: 1 in]
        n1344 = Format Date/Time String(time format string (%c)=w2942, seconds (now)=w2943) -> (date/time string=w2934:string)  [unwired: 1 in]
        n1345 = Build Array(w2937, w2936, w2935, w2934) -> (w2928:string[])
        n1346 = Build Array(w2927, w2926) -> (w2924:u16[])
        n1347 = call "REPORT_PACE_get_data_from_SQL.vi"("low_limit_high_limit"=w2924, "error_in"=w2932, "dates_array"=w2928) -> ("error_out"=w2931:errorcluster, "SQL_result"=w2929:variant, "executed_SQL_statement"=w2930:string)  [unwired: 6 in]
        n1348 = To Variant(anything=w2924) -> (Variant=w2923:variant)
        n1349 = call "FGV_REPORTS_records_display.vi"("options"=FGV_REPORTS_records_display."PACE_set_limits", "input"=w2923) -> ()  [unwired: 8 in, 2 out]
        n1350 = call "FGV_REPORTS_records_display.vi"("options"=FGV_REPORTS_records_display."PACE_set_records", "error_in"=w2931, "input"=w2929) -> ("error_out"=w2939:errorcluster)  [unwired: 7 in, 1 out]
        n1351 = call "FGV_REPORTS_records_display.vi"("options"=FGV_REPORTS_records_display."PACE_display", "error_in"=w2939) -> ("error_out"=w2938:errorcluster)  [unwired: 8 in, 1 out]
        n1352 = call "FGV_REPORTS_status_display.vi"("options"=FGV_REPORTS_status_display."display", "error_in"=w2938, "SQL_statement"=w2930, "display_source"="PACE REPORT") -> ("error_out"=w2948:errorcluster)  [unwired: 7 in]
        n1353 = call "SQL_EDITOR_check_for_error.vi"("SQL_EDITOR_loop_state_in"=SQL_EDITOR_sequence_state."get_next_state", "error_in"=w2948) -> ("SQL_EDITOR_loop_state_out"=w2951:T25, "error_out"=w2952:errorcluster)  [unwired: 8 in]
      }
      frame "REPORT_CBATCH_scan_barcode" {
        n1354 = Variant To Data(error in=w2956, type="", Variant=w2957) -> (data=w2953:string, error out=w2954:errorcluster)
        n1355 = local write "REPORT_CBATCH_batch_code"(w2953) -> ()
        n1356 = call "SQL_EDITOR_check_for_error.vi"("SQL_EDITOR_loop_state_in"=SQL_EDITOR_sequence_state."get_next_state", "error_in"=w2954) -> ("SQL_EDITOR_loop_state_out"=w2959:T25, "error_out"=w2960:errorcluster)  [unwired: 8 in]
      }
      frame "REPORT_CBATCH_get" {
        n1357 = local read "REPORT_CBATCH_batch_code"() -> (w2963:string)
        n1358 = call "REPORT_CBATCH_get_data_from_SQL.vi"("error_in"=w2967, "cbatch_code"=w2963) -> ("error_out"=w2966:errorcluster, "SQL_result"=w2964:variant, "executed_SQL_statement"=w2965:string)  [unwired: 7 in]
        n1359 = call "FGV_REPORTS_records_display.vi"("options"=FGV_REPORTS_records_display."CBATCH_set_records", "error_in"=w2966, "input"=w2964) -> ("error_out"=w2969:errorcluster)  [unwired: 7 in, 1 out]
        n1360 = local read "REPORT_CBATCH_order_selection"() -> (w2961:enum32{"old_to_new", "new_to_old"})
        n1361 = To Variant(anything=w2961) -> (Variant=w2962:variant)
        n1362 = call "FGV_REPORTS_records_display.vi"("options"=FGV_REPORTS_records_display."CBATCH_display", "error_in"=w2969, "input"=w2962) -> ("error_out"=w2968:errorcluster)  [unwired: 7 in, 1 out]
        n1363 = call "FGV_REPORTS_status_display.vi"("options"=FGV_REPORTS_status_display."display", "error_in"=w2968, "SQL_statement"=w2965, "display_source"="CUSTOMER BATCH REPORT") -> ("error_out"=w2973:errorcluster)  [unwired: 7 in]
        n1364 = call "SQL_EDITOR_check_for_error.vi"("SQL_EDITOR_loop_state_in"=SQL_EDITOR_sequence_state."get_next_state", "error_in"=w2973) -> ("SQL_EDITOR_loop_state_out"=w2976:T25, "error_out"=w2977:errorcluster)  [unwired: 8 in]
      }
      frame "REPORT_CMPNT_scan_barcode" {
        n1365 = Variant To Data(error in=w2981, type="", Variant=w2982) -> (data=w2978:string, error out=w2979:errorcluster)
        n1366 = local write "REPORT_CMPNT_gear_serial"(w2978) -> ()
        n1367 = call "SQL_EDITOR_check_for_error.vi"("SQL_EDITOR_loop_state_in"=SQL_EDITOR_sequence_state."get_next_state", "error_in"=w2979) -> ("SQL_EDITOR_loop_state_out"=w2984:T25, "error_out"=w2985:errorcluster)  [unwired: 8 in]
      }
      frame "REPORT_CMPNT_get" {
        n1368 = local read "REPORT_CMPNT_gear_serial"() -> (w2986:string)
        n1369 = call "REPORT_CMPNT_get_data_from_SQL.vi"("error_in"=w2990, "gear_serial"=w2986) -> ("error_out"=w2989:errorcluster, "SQL_result"=w2987:variant, "executed_SQL_statement"=w2988:string)  [unwired: 7 in]
        n1370 = call "FGV_REPORTS_records_display.vi"("options"=FGV_REPORTS_records_display."CMPNT_set_records", "error_in"=w2989, "input"=w2987) -> ("error_out"=w2992:errorcluster)  [unwired: 7 in, 1 out]
        n1371 = call "FGV_REPORTS_records_display.vi"("options"=FGV_REPORTS_records_display."CMPNT_display", "error_in"=w2992) -> ("error_out"=w2991:errorcluster)  [unwired: 8 in, 1 out]
        n1372 = call "FGV_REPORTS_status_display.vi"("options"=FGV_REPORTS_status_display."display", "error_in"=w2991, "SQL_statement"=w2988, "display_source"="GEAR COMPONENTS REPORT") -> ("error_out"=w2996:errorcluster)  [unwired: 7 in]
        n1373 = call "SQL_EDITOR_check_for_error.vi"("SQL_EDITOR_loop_state_in"=SQL_EDITOR_sequence_state."get_next_state", "error_in"=w2996) -> ("SQL_EDITOR_loop_state_out"=w2999:T25, "error_out"=w3000:errorcluster)  [unwired: 8 in]
      }
      frame "REPORT_save_pdf" {
        n1374 = local read "REPORT_filters"() -> (w3001:T2)
        n1375 = case shown="\"Audits\"" w3001 {
          tunnel: [w3008 w3009 w3011 w3013 w3016 w3017 w3019 w3021 w3023 w3025 w3030 w3032] -> w3003
          tunnel: w3002 -> [w3007 w3010 w3012 w3014 w3015 w3018 w3020 w3022 w3024 w3026 w3031 w3032]
          frame "Gear" {
            n1376 = call "REPORT_GEAR_save_pdf.vi"("error_in"=w3007) -> ("error_out"=w3008:errorcluster)  [unwired: 10 in]
          }
          frame "Dates" {
            n1377 = call "REPORT_DATES_save_pdf.vi"("error_in"=w3010) -> ("error_out"=w3009:errorcluster)  [unwired: 10 in]
          }
          frame "Production Batch" {
            n1378 = call "REPORT_PBATCH_save_pdf.vi"("error_in"=w3012) -> ("error_out"=w3011:errorcluster)  [unwired: 10 in]
          }
          frame "Config History" {
            n1379 = call "REPORT_CFG_save_pdf.vi"("error_in"=w3014) -> ("error_out"=w3013:errorcluster)  [unwired: 10 in]
          }
          frame "Audits" {
            n1380 = call "REPORT_AUDIT_save_pdf.vi"("error_in"=w3015) -> ("error_out"=w3016:errorcluster)  [unwired: 10 in]
          }
          frame "OK/NOK Count" {
            n1381 = call "REPORT_OKNOK_save_pdf.vi"("error_in"=w3018) -> ("error_out"=w3017:errorcluster)  [unwired: 10 in]
          }
          frame "Reworks" {
            n1382 = call "REPORT_REWORKS_save_pdf.vi"("error_in"=w3020) -> ("error_out"=w3019:errorcluster)  [unwired: 10 in]
          }
          frame "Pace" {
            n1383 = call "REPORT_PACE_save_pdf.vi"("error_in"=w3022) -> ("error_out"=w3021:errorcluster)  [unwired: 10 in]
          }
          frame "Customer Batch" {
            n1384 = call "REPORT_CBATCH_save_pdf.vi"("error_in"=w3024) -> ("error_out"=w3023:errorcluster)  [unwired: 10 in]
          }
          frame "Gear Components" {
            n1385 = call "REPORT_CMPNT_save_pdf.vi"("error_in"=w3026) -> ("error_out"=w3025:errorcluster)  [unwired: 10 in]
          }
          frame "Operation" {
            n1386 = call "message_popup.vi"("error_in"=w3031, "Message"="Due to it's size PDF version of Operation report cannot be generated. Please generate CSV report instead.", "Title"="REPORT CANNOT BE GENERATED ", "Button Label"="OK") -> ("error_out"=w3030:errorcluster)  [unwired: 7 in]
          }
          frame Default {
          }
        }
        n1387 = call "SQL_EDITOR_check_for_error.vi"("SQL_EDITOR_loop_state_in"=SQL_EDITOR_sequence_state."get_next_state", "error_in"=w3003) -> ("SQL_EDITOR_loop_state_out"=w3005:T25, "error_out"=w3006:errorcluster)  [unwired: 8 in]
      }
      frame "REPORT_save_csv" {
        n1388 = local read "REPORT_filters"() -> (w3033:T2)
        n1389 = case shown="\"Audits\"" w3033 {
          tunnel: [w3040 w3041 w3043 w3045 w3047 w3049 w3051 w3053 w3055 w3057 w3059 w3061] -> w3035
          tunnel: w3034 -> [w3039 w3042 w3044 w3046 w3048 w3050 w3052 w3054 w3056 w3058 w3060 w3061]
          frame "Gear" {
            n1390 = call "REPORT_GEAR_save_csv.vi"("error_in"=w3039) -> ("error_out"=w3040:errorcluster)  [unwired: 10 in]
          }
          frame "Dates" {
            n1391 = call "REPORT_DATES_save_csv.vi"("error_in"=w3042) -> ("error_out"=w3041:errorcluster)  [unwired: 10 in]
          }
          frame "Production Batch" {
            n1392 = call "REPORT_PBATCH_save_csv.vi"("error_in"=w3044) -> ("error_out"=w3043:errorcluster)  [unwired: 10 in]
          }
          frame "Operation" {
            n1393 = call "REPORT_OPRTN_save_csv.vi"("error_in"=w3046) -> ("error_out"=w3045:errorcluster)  [unwired: 10 in]
          }
          frame "Config History" {
            n1394 = call "REPORT_CFG_save_csv.vi"("error_in"=w3048) -> ("error_out"=w3047:errorcluster)  [unwired: 10 in]
          }
          frame "Audits" {
            n1395 = call "REPORT_AUDIT_save_csv.vi"("error_in"=w3050) -> ("error_out"=w3049:errorcluster)  [unwired: 10 in]
          }
          frame "OK/NOK Count" {
            n1396 = call "REPORT_OKNOK_save_csv.vi"("error_in"=w3052) -> ("error_out"=w3051:errorcluster)  [unwired: 10 in]
          }
          frame "Reworks" {
            n1397 = call "REPORT_REWORKS_save_csv.vi"("error_in"=w3054) -> ("error_out"=w3053:errorcluster)  [unwired: 10 in]
          }
          frame "Pace" {
            n1398 = call "REPORT_PACE_save_csv.vi"("error_in"=w3056) -> ("error_out"=w3055:errorcluster)  [unwired: 10 in]
          }
          frame "Customer Batch" {
            n1399 = call "REPORT_CBATCH_save_csv.vi"("error_in"=w3058) -> ("error_out"=w3057:errorcluster)  [unwired: 10 in]
          }
          frame "Gear Components" {
            n1400 = call "REPORT_CMPNT_save_csv.vi"("error_in"=w3060) -> ("error_out"=w3059:errorcluster)  [unwired: 10 in]
          }
          frame Default {
          }
        }
        n1401 = call "SQL_EDITOR_check_for_error.vi"("SQL_EDITOR_loop_state_in"=SQL_EDITOR_sequence_state."get_next_state", "error_in"=w3035) -> ("SQL_EDITOR_loop_state_out"=w3037:T25, "error_out"=w3038:errorcluster)  [unwired: 8 in]
      }
      frame "error" {
        w3062 = SQL_EDITOR_sequence_state."stop" ("y")
        n1402 = call <vilib>:"Clear Errors.vi"("error in (no error)"=w3076) -> ("error out"=w3075:errorcluster)  [unwired: 5 in, 1 out]
        n1403 = Unbundle By Name(w3068) -> ("queue_refnums.SQL_EDITOR_queue"=w3067:refnum<queue>)
        n1404 = call "FGV_CLIENT_SQL_connection.vi"("options"=FGV_CLIENT_SQL_connection."connection_active?", "error_in"=w3075) -> ("error_out"=w3073:errorcluster, "connection_active?"=w3071:bool)  [unwired: 5 in, 3 out]
        n1405 = case shown="False" w3071 {
          tunnel: [SQL_EDITOR_sequence_state."initialize" ("ST_TCP_sequence_state") SQL_EDITOR_sequence_state."get_next_state" ("ST_TCP_sequence_state")] -> w3065
          tunnel: [w3081 w3083] -> w3072
          tunnel: w3073 -> [w3077 w3083]
          frame False {
            # "ERROR WITH CONNECTION"
            n1406 = Unbundle By Name(w3077) -> ("status"=w3078:bool)
            n1407 = local write "SQL_connection_indicator"(w3078) -> ()
            n1408 = call "FGV_CLIENT_SQL_connection.vi"("options"=FGV_CLIENT_SQL_connection."disconnect", "error_in"=w3077) -> ("error_out"=w3080:errorcluster)  [unwired: 5 in, 4 out]
            n1409 = call <vilib>:"Clear Errors.vi"("error in (no error)"=w3080) -> ("error out"=w3081:errorcluster)  [unwired: 5 in, 1 out]
          }
          frame True {
            # "ERROR WITH SQL STATEMENT OR SIMILAR"
          }
        }
        n1410 = Preview Queue Element(queue=w3067, timeout in ms (-1)=0) -> (element=w3070:T32)  [unwired: 1 in, 3 out]
        n1411 = Unbundle By Name(w3070) -> ("state"=w3063:T25)
        n1412 = Equal?(x=w3062, y=w3063) -> (x = y?=w3066:bool)
        n1413 = Select(t=w3062, s=w3066, f=w3065) -> (s? t:f=w3064:T25)
        n1414 = call "wait_on_initialization.vi"("state"=w3064) -> ()  [unwired: 11 in]
      }
      frame "stop" {
      }
    }
  }
  n1415 = Merge Errors(w146, w145, w85, w20) -> (w137:errorcluster)
  n1416 = call "FGV_CLIENT_SQL_connection.vi"("options"=FGV_CLIENT_SQL_connection."disconnect", "error_in"=w137) -> ("error_out"=w136:errorcluster)  [unwired: 5 in, 4 out]
  n1417 = control-ref of="This VI"() -> (w150:refnum<vi>)
  n1418 = call "CLIENT_destroy_queues.vi"("error_in"=w136, "all_config_info"=w21) -> ("error_out"=w151:errorcluster)  [unwired: 9 in]
  n1419 = call "close_front_panel_in_exe.vi"("error_in"=w151, "vi_reference_in"=w150) -> ("error_out"=w149:errorcluster)  [unwired: 9 in]
  n1420 = call <vilib>:"Clear Errors.vi"("error in (no error)"=w149) -> ()  [unwired: 5 in, 2 out]
